vi "ControlProgram5.3.vi"() -> ()   [LabVIEW 2016]
uses:
  <vilib>/Utility/error.llb/DialogType.ctl
  <vilib>/Utility/miscctls.llb/LVPoint32TypeDef.ctl
  <vilib>/DAQmx/write.llb/DAQmx Write (Digital Bool 1Line 1Point).vi
  <vilib>/DAQmx/create/channels.llb/DAQmx Create Channel (DO-Digital Output).vi
  <vilib>/platform/TimedLoop/XDataNode/XDataNode.xnode
  <vilib>/Platform/TimedLoop/XDataNode/nitl_modes.ctl
  <vilib>/Platform/TimedLoop/XDataNode/XDNodeRunTimeDep.lvlib
  <vilib>/Platform/TimedLoop/XDataNode/wakeup.ctl
  <vilib>/Platform/TimedLoop/XDataNode/timing_clust.ctl
  <vilib>/DAQmx/create/channels.llb/DAQmx Create Channel (AI-Voltage-Basic).vi
  <vilib>/DAQmx/create/channels.llb/DAQmx Create Channel (AO-Voltage-Basic).vi
  <vilib>/DAQmx/write.llb/DAQmx Write (Analog 1D DBL NChan 1Samp).vi
  <resource>/objmgr/daqmx.rc
  <vilib>/Analysis/NI_AALBase.lvlib
  <vilib>/Analysis/baseanly.llb/Mean (DBL).vi
  <vilib>/Instr/_visa.llb/VISA Configure Serial Port (Instr).vi
  <vilib>/DAQmx/read.llb/DAQmx Read (Analog 2D DBL NChan NSamp).vi
  <vilib>/Utility/inputDevices.llb/closeMouse.vi
  <vilib>/Utility/inputDevices.llb/mouseAcquire.vi
  <vilib>/DAQmx/configure/timing.llb/DAQmx Timing (Sample Clock).vi
panel:
  out "Numeric 2":i32
  out "Numeric":i32
  in  "dt":dbl
  out "Flush Sample Start Time":u32
  out "Sample flush time (s)":dbl=100.0
  in  "Inject Sample":bool
  out "Chart Freq (Hz)":dbl
  out "Cal values":T1={"AX alpha"=672.9952101249002, "BX alpha"=822.8320399167465, "AX kappa"=0.3432739170419873, "BX kappa"=0.22087046979741862, "AX offset"=-0.002065833400375715, "BX offset"=0.010483360643544744, "AY alpha"=702.0654168010462, "BY alpha"=773.6701766674906, "AY kappa"=0.33643150106915, "BY kappa"=0.2444549177225145, "AY offset"=-0.1177594339643395, "BY offset"=0.06470506082263472}
  in  "Inject Pump 1":bool
  in  "Inject Pump 2":bool
  in  "Tab Control 2":T2(tab)
  in  "Force FB script":bool
  in  "Got ADig bead":bool
  in  "Move Cap. 2 (ADig Top)":bool
  in  "Dump beads":bool
  in  "Got DNA bead":bool
  in  "Flow on\ncap 2?":bool=TRUE
  in  "Flow on\ncap 1?":bool=TRUE
  in  "Flow on\ndump?":bool=TRUE
  in  "Delta after tether":dbl=2.4
  in  "TA Cancel Save?":bool
  in  "Min fish\ndelta (V)":dbl=2.8 min=0.0 max=10.0 step=0.1
  in  "Max fish\ndelta (V)":dbl=3.8 min=0.0 max=10.0 step=0.1
  in  "Fish Speed (ms)":i32=3000
  in  "Wait (ms)":i32=1500
  in  "# attempts":dbl=10.0
  in  "Cutoff force (pN)":dbl=5.0
  in  "Raster after\n tether?":bool=TRUE
  out "Tether":bool
  out "Attempt #":i32
  in  "Flow on\nwhile fish?":bool=TRUE
  in  "Flow on\nafter raster?":bool=TRUE
  in  "Offset @ Delta (V)":dbl=2.4
  in  "Cal @ Delta (V)":dbl=5.0
  in  "Cal stage position":i32=3
  in  "Conv Y (nm/V)":dbl=505.0
  in  "Conv X (nm/V)":dbl=892.0
  out "Cal Final Sampling Rate":dbl
  in  "Cal Averaging":i32=1
  in  "Wait before dip (s)":dbl=3.0
  in  "Start dipping after?":bool
  in  "Start trap delta (V)":dbl=3.85
  in  "Cancel dwell":bool
  in  "Pause dwell":bool
  in  "Return position":dbl=3.0
  in  "Dip duration":dbl=15.0
  in  "Dip position":dbl=4.0
  in  "Dip":bool
  out "Dip time":i32
  in  "Stop":bool=TRUE
  in  "?":T3(tab)=enum."Mouse control"
  in  "Save N sets":bool
  in  "N sets":i32=200
  in  "Cal sets to save":i32=500
  in  "Reset data stream":bool
  out "Buffer Overflow":bool
  out "Stage moving":bool
  in  "Comment":string="wtUvrD 0.5 uM ATP"
  in  "Raster scan":bool
  out "Saving":bool
  in  "Save cal":bool
  in  "Save Data":bool
  in  "Stop saving":bool
  out "Calibrating":bool
  out "Progress":dbl(slide) scale=0.0..100.0
  in  "Read Cal":bool
  in  "Fish":bool
  in  "Averaging Number":i32=1250
  out "Final Sampling Rate":dbl=100.0
  in  "Trap position":cluster{"X":dbl, "Y":dbl}={"X"=1.6, "Y"=4.95}
  in  "Trap delta":dbl=5.1 min=0.0 max=10.0 step=0.1
  in  "Fixed X":dbl=1.6
  in  "Fixed Y":dbl=0.7
  in  "Shutter 1 (B)":bool
  in  "Shutter 2 (A)":bool
  in  "Pulling direction":bool=TRUE
  out "Raster scanning...":bool
  out "Current file name":path
  in  "AX alpha":dbl format="%#_3p"
  in  "BX alpha":dbl format="%#_3g"
  in  "AX kappa":dbl format="%#_3g"
  in  "BX kappa":dbl format="%#_3g"
  in  "AX offset":dbl format="%#_3g"
  in  "BX offset":dbl format="%#_3g"
  in  "AY alpha":dbl format="%#_3g"
  in  "BY alpha":dbl format="%#_3g"
  in  "AY kappa":dbl format="%#_3g"
  in  "BY kappa":dbl format="%#_3g"
  in  "AY offset":dbl format="%#_3g"
  in  "BY offset":dbl format="%#_3g"
  out "Buffer status":u8(slide) scale=0.0..100.0
  in  "dump spot":string="Dump beads spot"
  in  "up flow spot":string="Upper flow spot"
  in  "low flow spot":string="Lower flow spot"
  in  "up cap":string="Upper capillary (ADig beads)"
  in  "bottom cap":string="Lower capillary (DNA beads)"
  in  "Move to Position 5":bool
  in  "Set Position 5":bool
  in  "Saved stage positions":dbl[][](array[numeric])=[[1.0, 0.0, 0.0, 0.0], [2.0, 0.28481, -2.63158, -0.02256], [3.0, 1.27978, -0.73974, 0.0], [4.0, 1.27978, -2.1978, 0.0], [5.0, 0.03306, -2.63158, -0.02256]]
  in  "Set Position 2":bool
  in  "Move to Position 2":bool
  in  "Set Position 1":bool
  in  "Move to Position 1":bool
  in  "Set Position 4":bool
  in  "Move to Position 4":bool
  in  "Set Position 3":bool
  in  "Move to Position 3":bool
  out "Stage error":errorcluster
  in  "Clear Volume":bool
  out "Sample Flush Meter":u8(slide) scale=0.0..100.0
  out "Flushing Sample":bool
  in  "Flush Sample":bool
  in  "Normal \nRate (ul/hr)  3":dbl=100.0
  in  "Normal \nVolume (ul) 3":dbl=300.0
  in  "Normal \nVolume (ul) 2":dbl
  in  "Normal \nRate (ul/hr)":dbl
  in  "Normal \nVolume (ul)":dbl
  in  "Flush\nRate (ul/min)":dbl
  in  "Flush\nVolume (ul)":dbl
  in  "Flush \nRate (ul/min)  2":dbl
  in  "Flush Pump 2":bool
  in  "Flush\nVolume (ul)  2":dbl
  in  "Flush Pump 1":bool
  in  "Normal \nRate (ul/hr)  2":dbl
  in  "Write Wait":i32=1000
  in  "Flush \nRate (ul/min)  3":dbl=100.0
  in  "Flush\nVolume (ul)  3":dbl=100.0
  out "error out":errorcluster
  in  "Use Mouse to Move Trap?":bool
  in  "Pause Mouse/Mirror Connection":bool
  out "Reference Voltage":cluster{dbl, dbl}={0.0, -0.0}
  out "Saved voltage":cluster{dbl, dbl}
  out "Real Coordinates":cluster{"Horizontal":i32, "Vertical":i32}={"Horizontal"=145, "Vertical"=-1746}
  out "CoordinatesMousePressed":T4
  out "Sum error":dbl(knob) scale=-1.0..1.0
  out "Trap sep":waveform(dbl)[](graph)
  in  "Set reading to\nsetpoint":bool
  in  "Offset Y (nm)":dbl format="%0.2f"
  in  "Offset X (nm)":dbl format="%0.2f"
  in  "Remove offsets":bool
  in  "Force Feedback":bool
  out "Feedback Output Voltage 2":cluster{dbl, dbl} {"?" format="%#_4g"; "?" format="%#_4g"}
  in  "Max value X":dbl=10.0 format="%.1f"
  in  "Min value X":dbl format="%0.1f"
  in  "Max value Y":dbl=10.0 format="%.1f"
  in  "Min value Y":dbl format="%.1g"
  in  "Offset":cluster{"Off Y":dbl, "Off X":dbl}={"Off Y"=1.5, "Off X"=0.17}
  in  "Setpoint voltage":cluster{"SP Y":dbl, "SP X":dbl}={"SP Y"=0.6, "SP X"=0.0}
  in  "Feedback const":T5={"Ki_B_Y"=0.5, "Ki_B_X"=0.0, "Kp Y"=1.0, "Kp X"=0.0}
  out "Mean Trap Pos X 2 (nm)":dbl format="%0.2f"
  out "Mean Trp Pos Y 2 (nm)":dbl format="%0.2f"
  out "T2 X RMS (A)":dbl format="%0.2f"
  out "T2 Y RMS (A)":dbl format="%0.2f"
  in  "Scan range (nm)":dbl=500.0
  in  "Scan speed (nm/s)":dbl=100.0
  in  "Step size (nm)":dbl=1.0
  in  "Save scans":bool=TRUE
  in  "# scans":i32=1
  in  "Load param":bool
  in  "Scan Parameters":T6(array[cluster])=[{"Label"="Offset", "Max delta 2"=3.8, "Start delta 2"=2.4, "Speed (ms) 2"=10000, "# scans 2"=1}]
  in  "Trap delta\nafter":dbl=3.6
  in  "Stop raster":bool
  out "Scan range (V)":dbl
  out "Scan steps (mirror)":u64
  out "Scan increment (V)":dbl
  out "Time per step (ms)":dbl
  out "Total raster time (s)":dbl
  out "N sets to be saved":dbl
  out "Continue to display?":bool
  out "Video Error":errorcluster
  in  "# Samples/channel (in)":i32=40000 format="%.2f"
  out "Buffer size\n(Samples/channel)":u32
  out "DAQ rate\n(Samples/s)":dbl format="%#_6p"
  out "# Samples/channel":i32=1250
  out "# Samples/channel/s":dbl
  out "AvailSampPerChan":u32
  out "Data update period (s/set)":dbl format="%#_6p"
  out "AvailSampPerChan 2":u32
  in  "PC samp per channel":i32=1000
  in  "Sampling Rate":dbl=125000.0 format="%0.0p"
  in  "DAQ Rate2":dbl=1000000.0 format="%#_6p"
  out "Data period (s)":dbl format="%#_6p"
  in  "Tether break\nforce (pN)":dbl=1.0
  in  "Path":path=path "D:/data"
  in  "Save file index":dbl
  out "Mirror task":refnum<k21>
  in  "HWP1":string="Half waveplate 1: differential trap power"
  in  "HWP0":string="Half waveplate 0: total trap power"
  in  "Move 1":bool
  in  "\"Degrees\" 1":dbl
  in  "Move 0":bool
  in  "\"Degrees\" 0":dbl
  out "Chamber":T7(plugin-control)
  out "Deflection":T4
  in  "Sampling Rate":dbl=125000.0 format="%0.2f"
  in  "Averaging Number":i32=12500
  in  "DAQ Rate":dbl=1000000.0
  out "Final Sampling Rate":dbl
  in  "Tab Control":T8(tab)
  in  "Downsamp\nfact":dbl=250.0
  out "Bead sep":waveform(dbl)[](graph)
  out "Force (pN)":waveform(dbl)[](graph)
  out "Mean force (pN)":dbl format="%0.2f"
  out "Force noise (pN)":dbl format="%0.2f"
  out "Mean Bead Sep\n(nm)":dbl format="%0.2f"
  out "Bead Sep Noise\n(A)":dbl format="%0.2f"
  out "PSD 2":cluster{dbl[], dbl[]}(graph)
  out "PSD 1":cluster{dbl[], dbl[]}(graph)
  out "PSD 1 Sum":dbl(slide) scale=0.0..10.0
  out "PSD 2 Sum":dbl(slide) scale=0.0..10.0
  in  "Start":bool
  out "All signals":waveform(dbl)[](graph)
  # "Bead Calibration"
  # "X"
  # "Y"
  # "Pump #1 Controls"
  # "Pump #2 Controls"
  # "Sample Pump Controls"
  # "Retract the pumps manually. Change it back to INFUSE when you're done. Suck it up, don't whine."
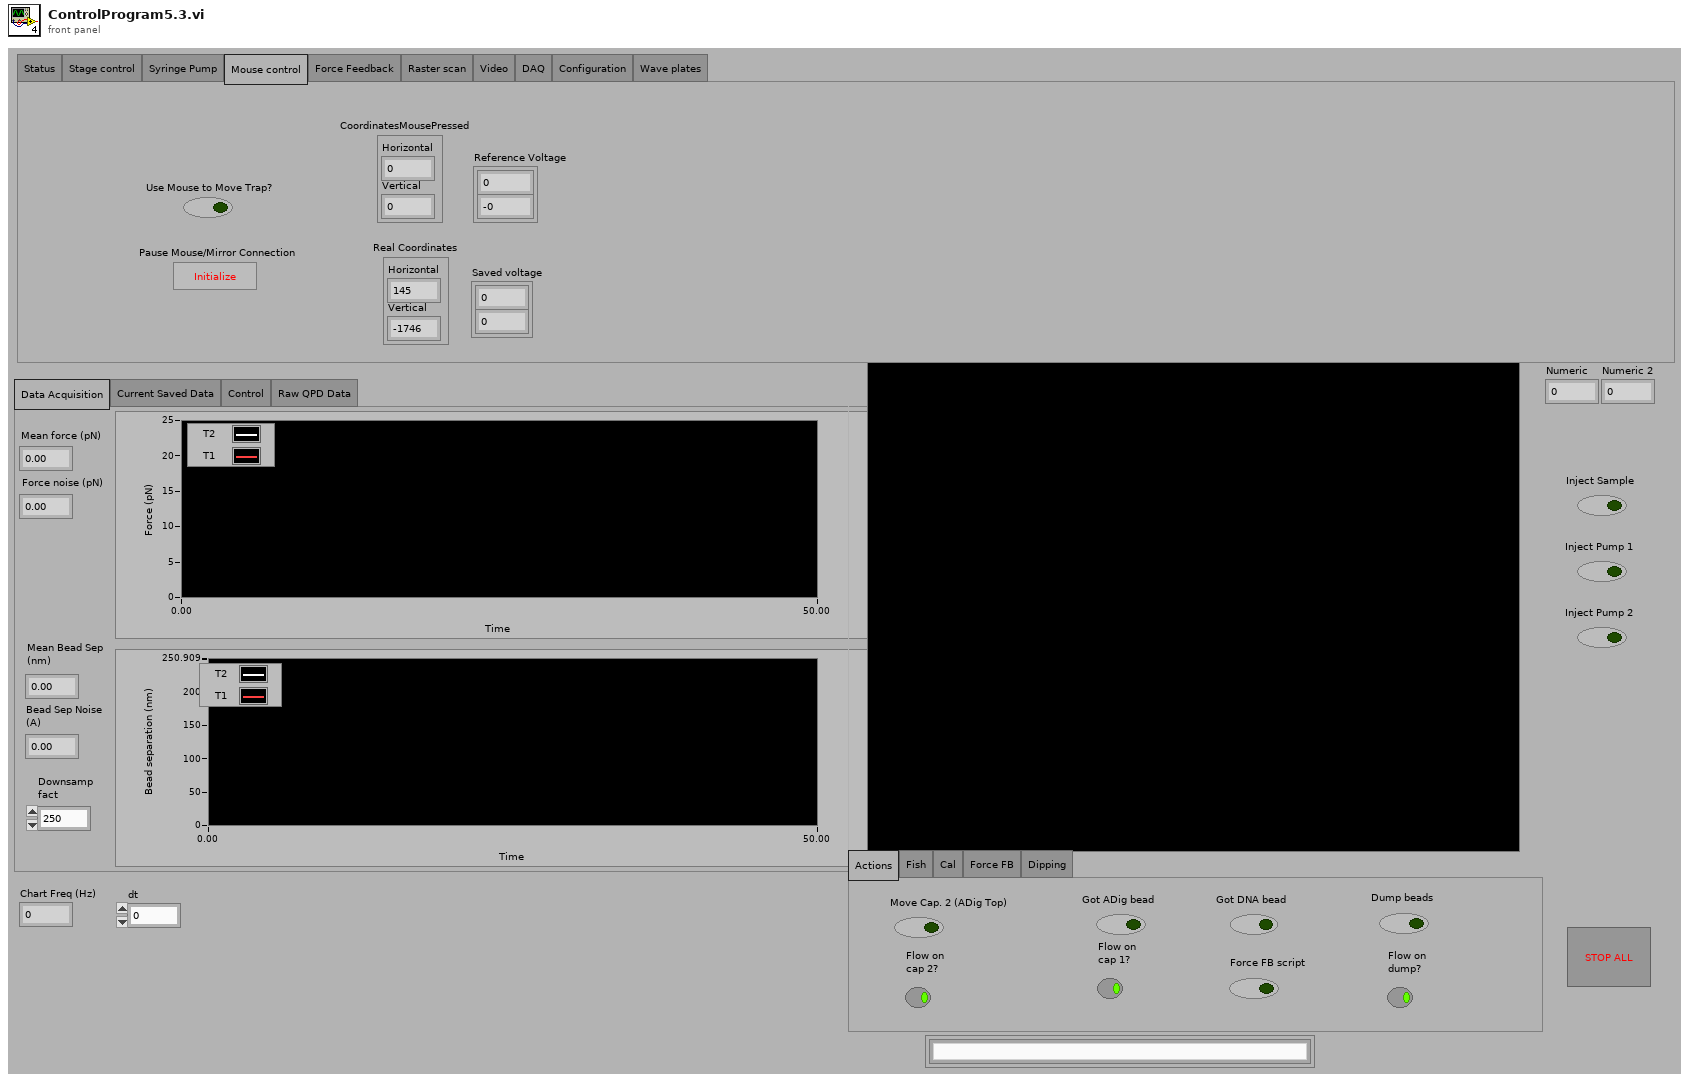
[diagram p1: front panel]
types:
  T1 = cluster{"AX alpha":dbl, "BX alpha":dbl, "AX kappa":dbl, "BX kappa":dbl, "AX offset":dbl, "BX offset":dbl, "AY alpha":dbl, "BY alpha":dbl, "AY kappa":dbl, "BY kappa":dbl, "AY offset":dbl, "BY offset":dbl}
  T2 = enum32{"Actions", "Fish", "Cal", "Force FB", "Dipping"}
  T3 = enum32{"Status", "Stage control", "Syringe Pump", "Mouse control", "Force Feedback", "Raster scan", "Video", "DAQ", "Configuration", "Wave plates"}
  T4 = typedef "LVPoint32TypeDef.ctl" = cluster{"Horizontal":i32, "Vertical":i32}
  T5 = cluster{"Ki_B_Y":dbl, "Ki_B_X":dbl, "Kp Y":dbl, "Kp X":dbl}
  T6 = cluster{"Label":string, "Max delta 2":dbl, "Start delta 2":dbl, "Speed (ms) 2":i32, "# scans 2":i32}[]
  T7 = typedef "IMAQ Image.ctl" = refnum<image>
  T8 = enum32{"Data Acquisition", "Current Saved Data", "Control", "Raw QPD Data"}
  T9 = enum16{"open", "replace", "create", "open or create", "replace or create", "replace or create with confirmation"}
  T10 = enum16{"big-endian, network order", "native, host order", "little-endian"}
  T11 = cluster{string, string, string, string, string, string, string, string}
  T12 = typedef "XDNodeRunTimeDep.lvlib/timing_clust.ctl" = cluster{"Expected End [f-1]":u64, "Actual End [f-1]":u64, "Finished Late? [f-1]":bool, "Expected End [i-1]":u64, "Actual End [i-1]":u64, "Finished Late? [i-1]":bool, "Expected Start [i]":u64, "Actual Start [i]":u64, "Expected Start [f]":u64, "Actual Start [f]":u64, "Source Name":string, "Structure Name":string, "Period":i64, "Deadline":i64, "Offset":i64, "Start":i64, "Priority":i32, "Timeout":i32, "Mode":T13, "Wakeup Reason":T14, "Error":errorcluster, "Source Type":string, "Secondary Source Type":string, "Global End Time":u64, "Global Start Time":u64, "Frame Duration":u64, "Iteration Duration":u64, "Assigned CPU":i32, "I/O Scan Engine Mode":u32}
  T13 = typedef "XDNodeRunTimeDep.lvlib/nitl_modes.ctl" = enum32{"No Change", "Process missed periods, maintain original phase", "Discard missed periods, maintain original phase", "Process missed periods, ignore original phase", "Discard missed periods, ignore original phase"}
  T14 = typedef "XDNodeRunTimeDep.lvlib/wakeup.ctl" = enum32{"Normal", "Aborted", "Asynchronous wakeup", "Timing source error", "Timed loop error", "Timeout"}
  T15 = typedef "DialogType.ctl" = u16
  T16 = cluster{"button 1":bool, "button 2":bool, "button 3":bool, "button 4":bool}
  T17 = cluster{"[0]":dbl, "[1]":dbl, "[2]":dbl, "[3]":dbl, "[4]":dbl, "[5]":dbl, "[6]":dbl, "[7]":dbl, "[8]":dbl, "[9]":dbl, "[10]":dbl, "[11]":dbl}
  T18 = cluster{"Label":string, "Max delta 2":dbl, "Start delta 2":dbl, "Speed (ms) 2":i32, "# scans 2":i32}
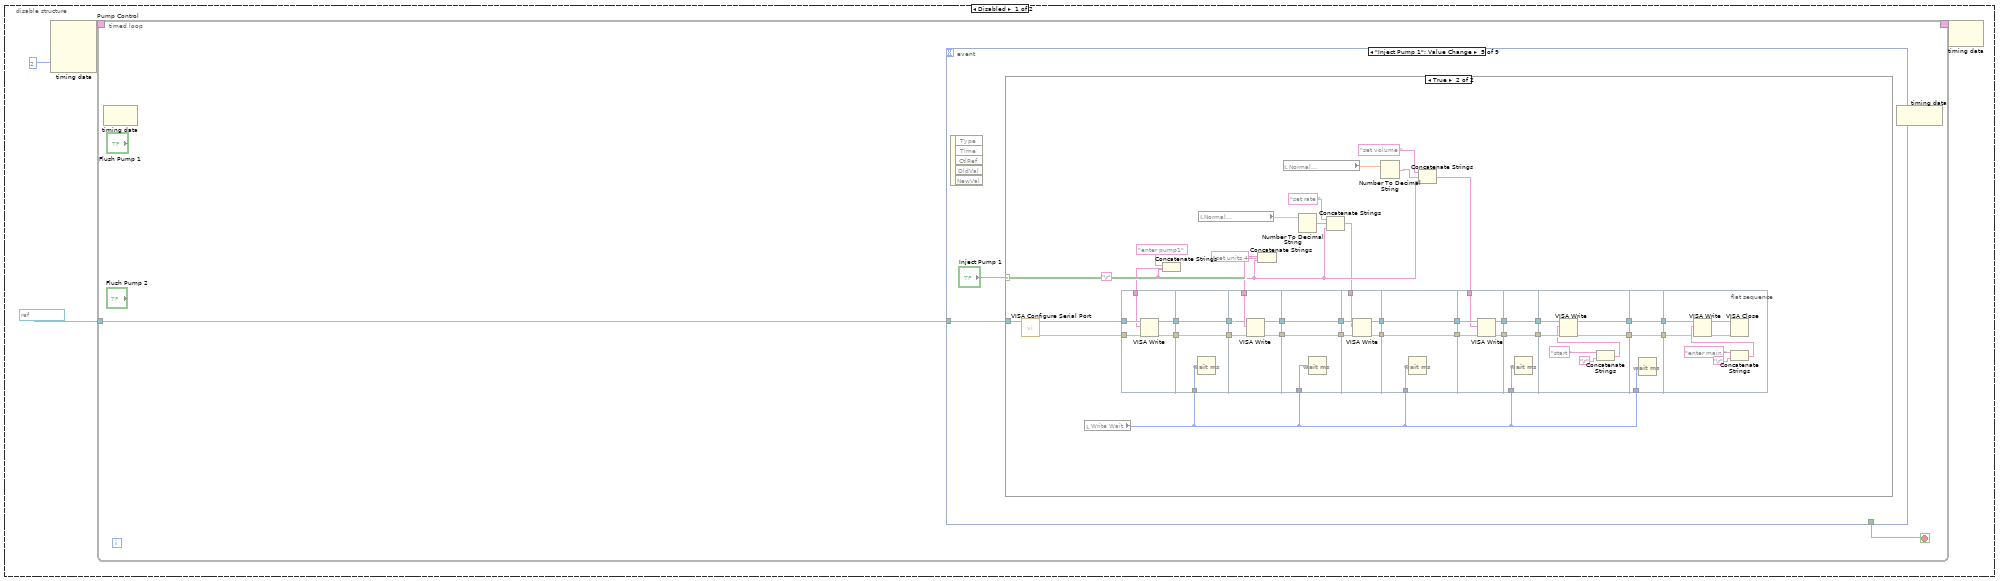
[diagram p2: hidden frame]
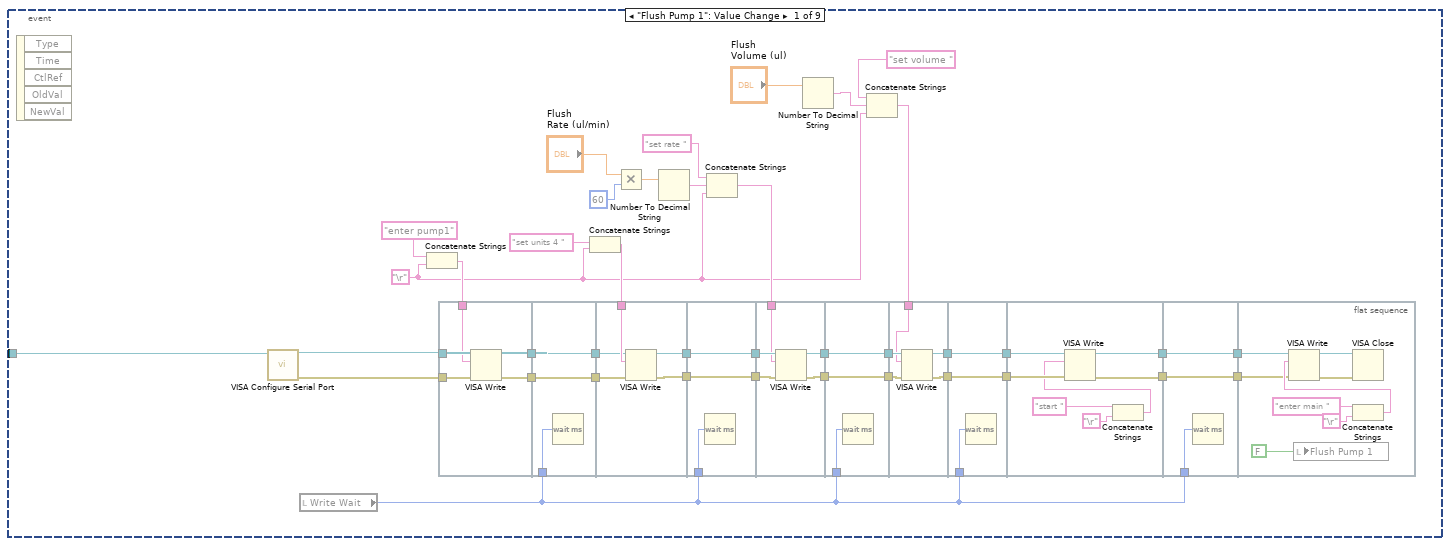
[diagram p3: hidden frame]
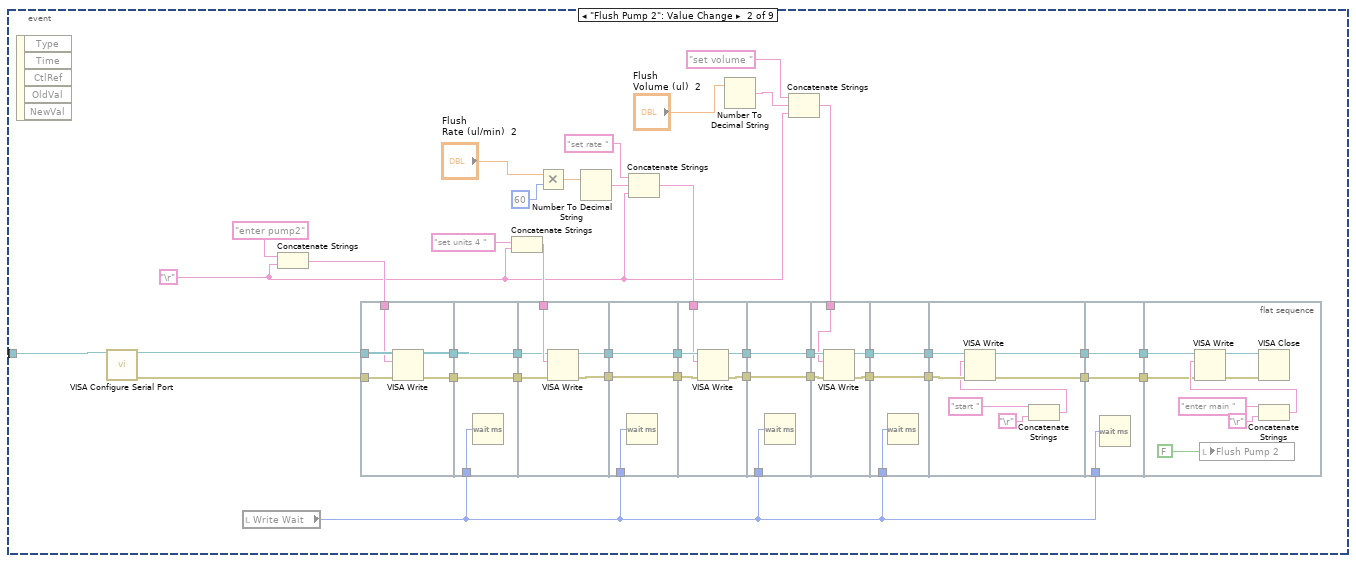
[diagram p4: hidden frame]
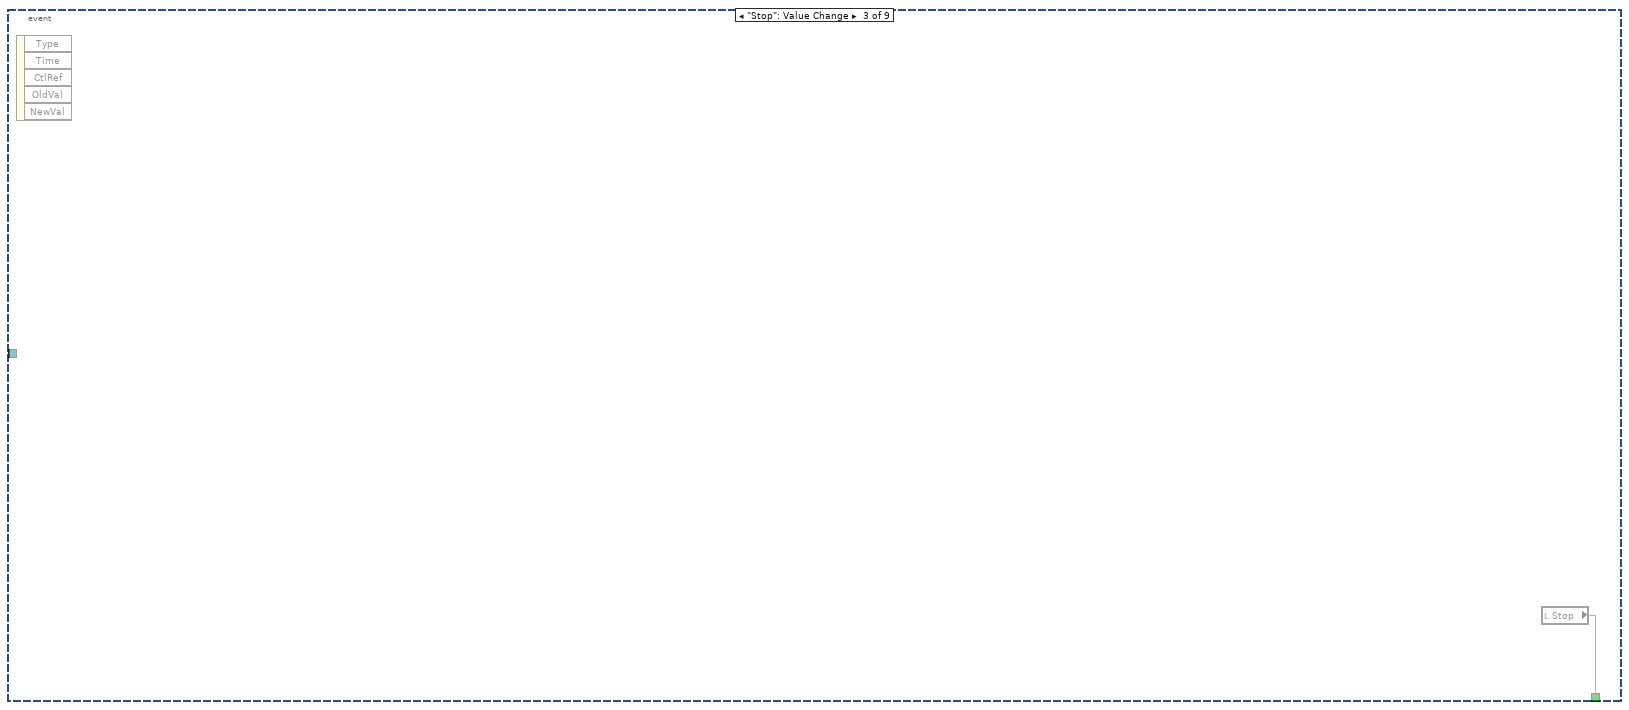
[diagram p5: hidden frame]
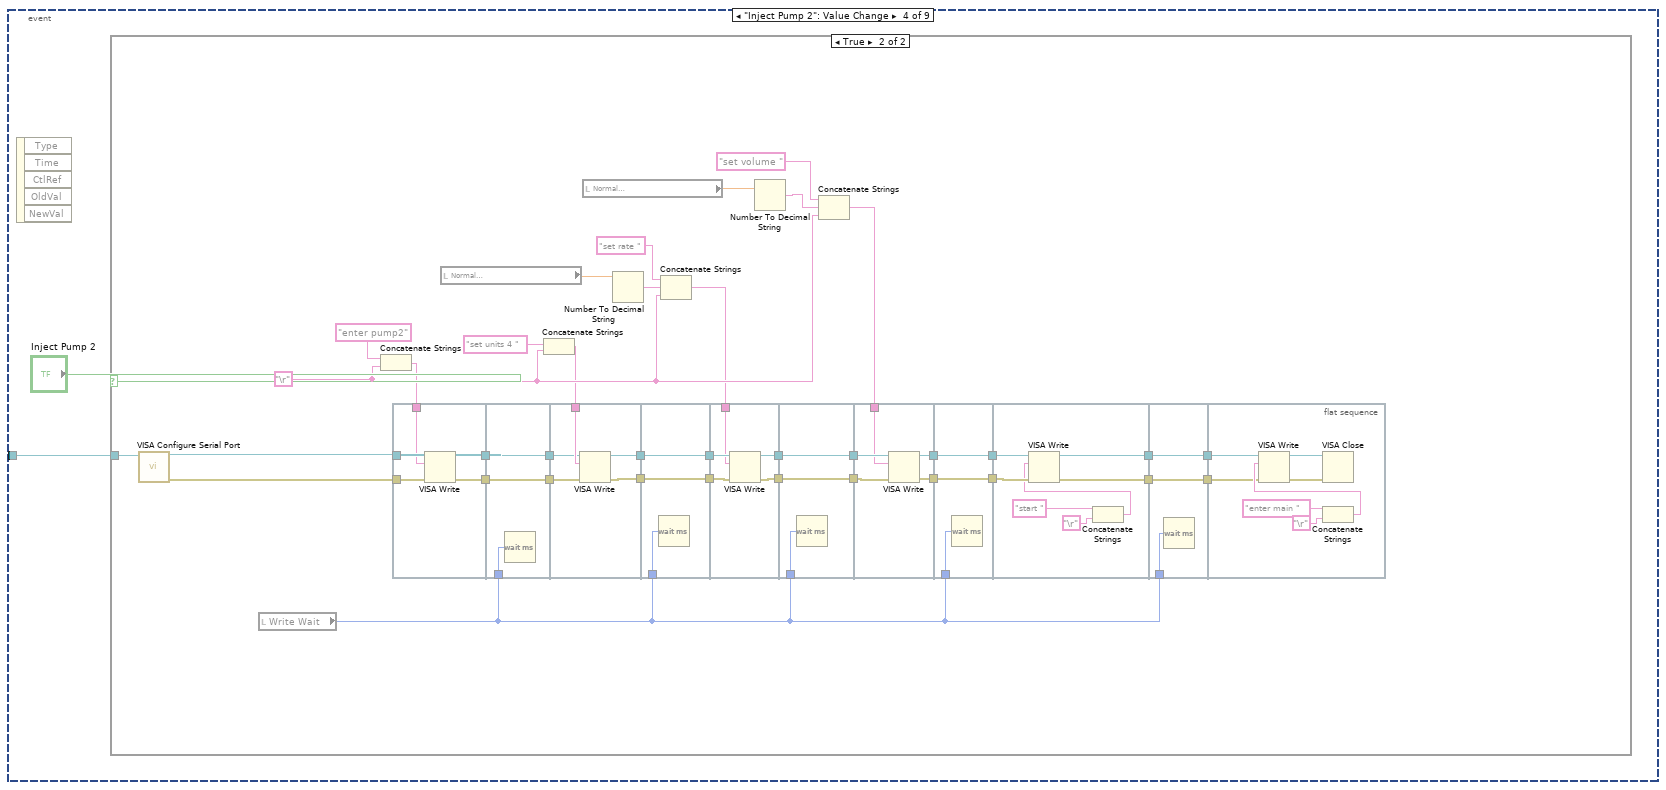
[diagram p6: hidden frame]
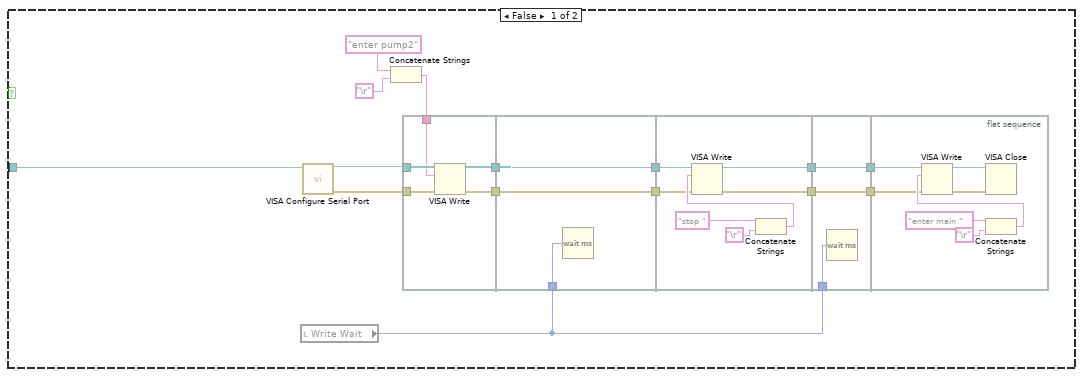
[diagram p7: hidden frame]
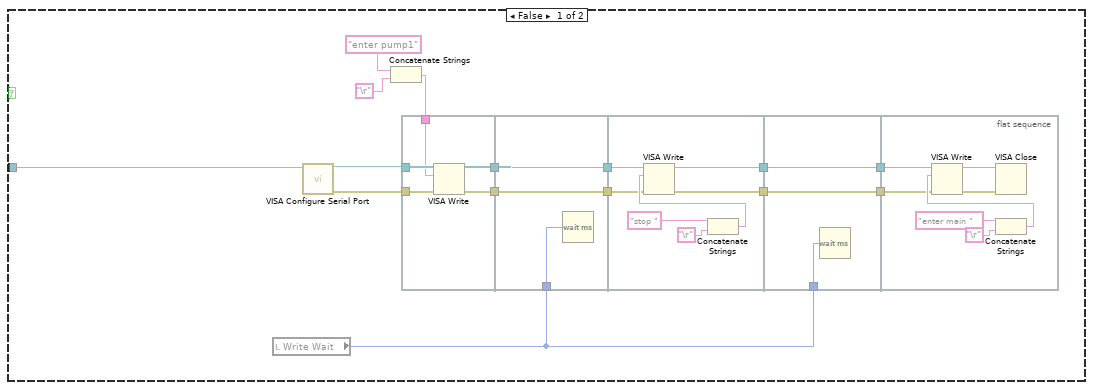
[diagram p8: hidden frame]
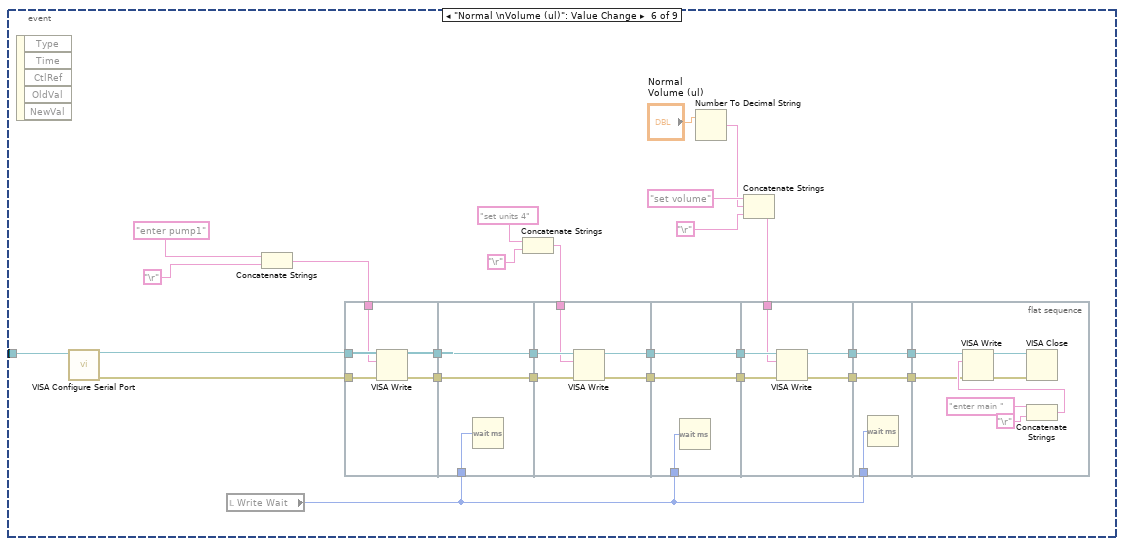
[diagram p9: hidden frame]
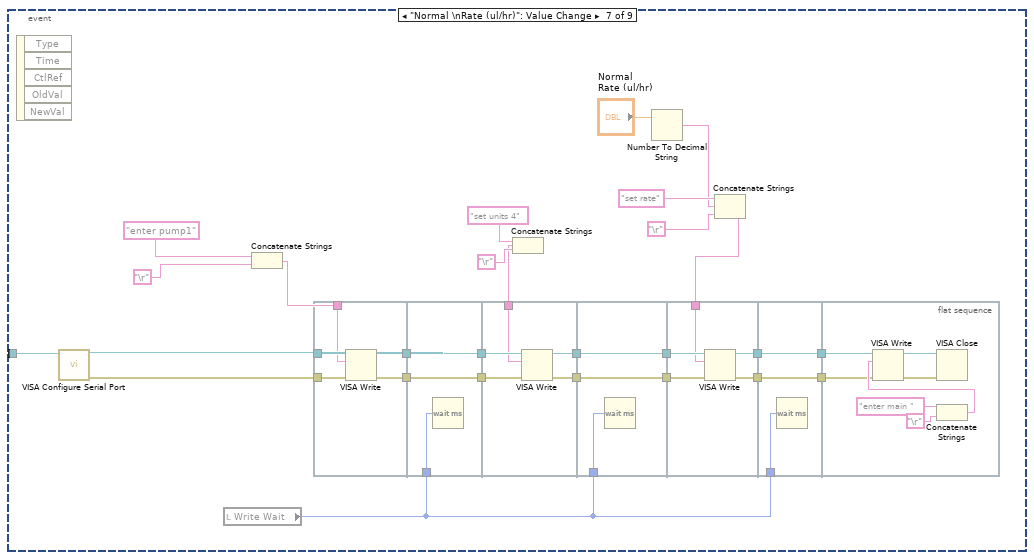
[diagram p10: hidden frame]
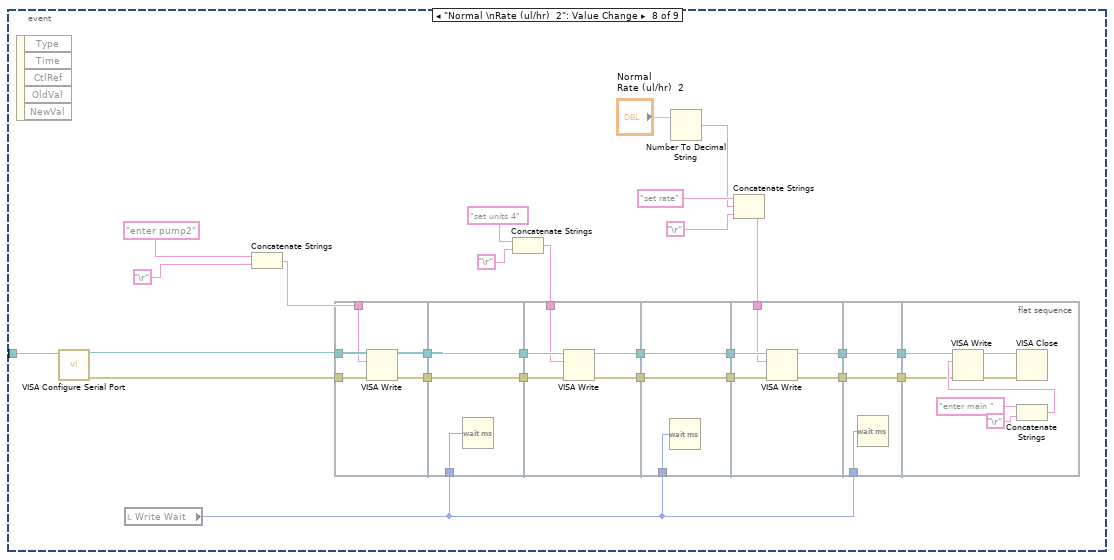
[diagram p11: hidden frame]
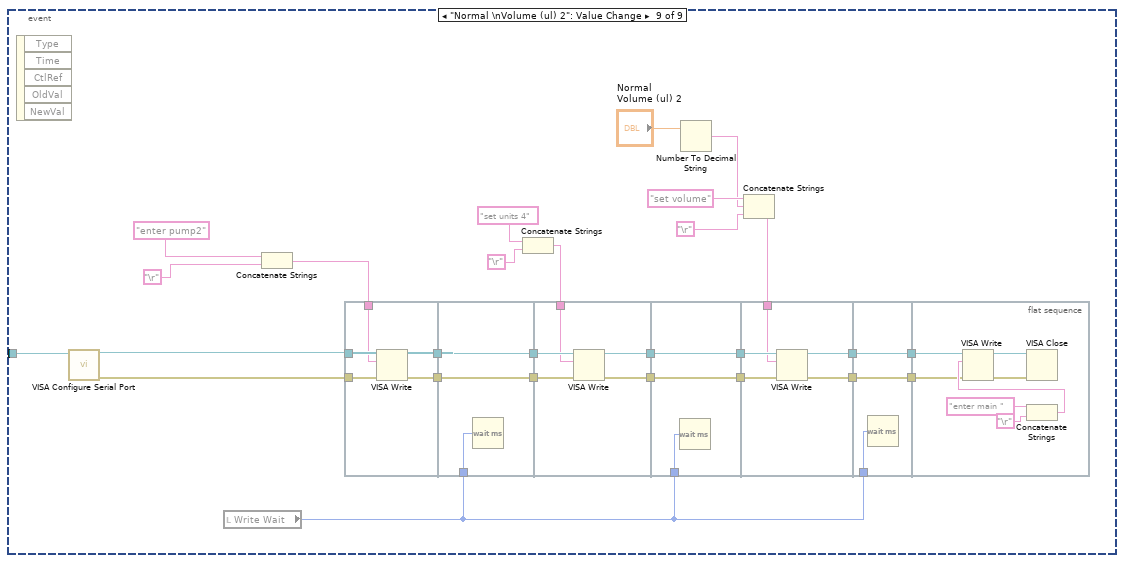
[diagram p12: hidden frame]
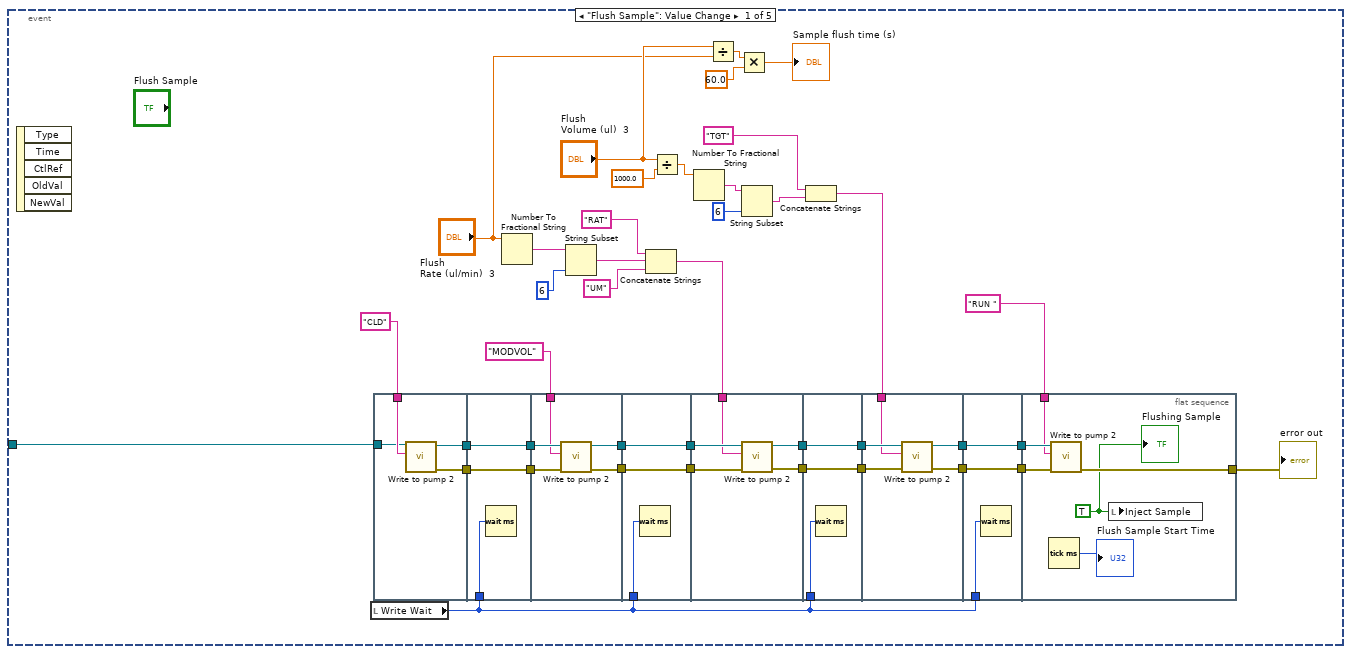
[diagram p13: hidden frame]
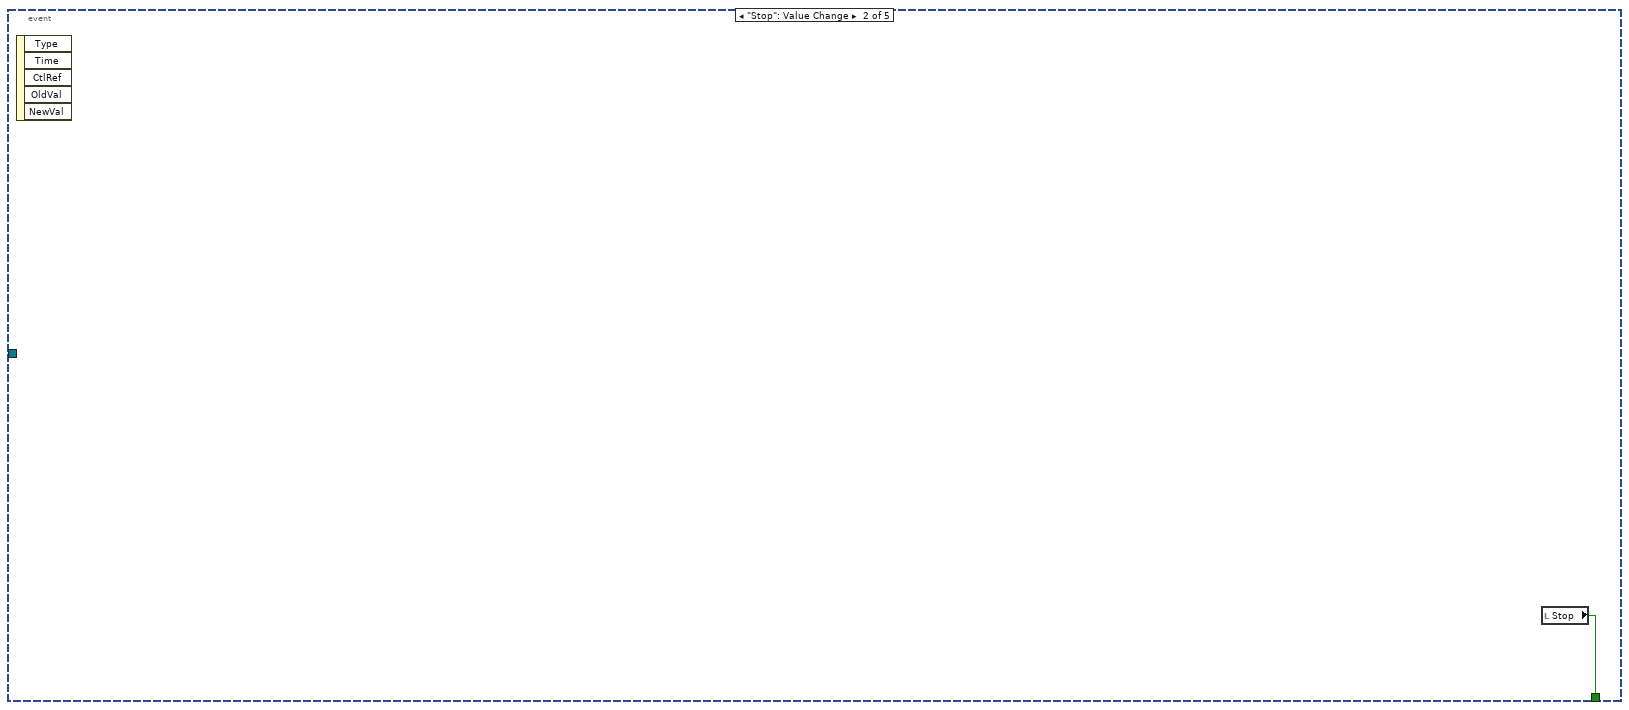
[diagram p14: hidden frame]
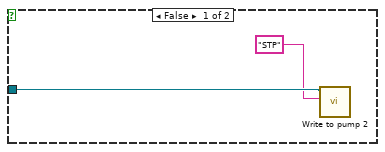
[diagram p15: hidden frame]
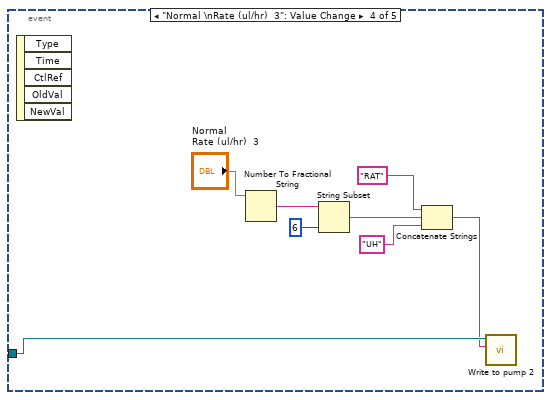
[diagram p16: hidden frame]
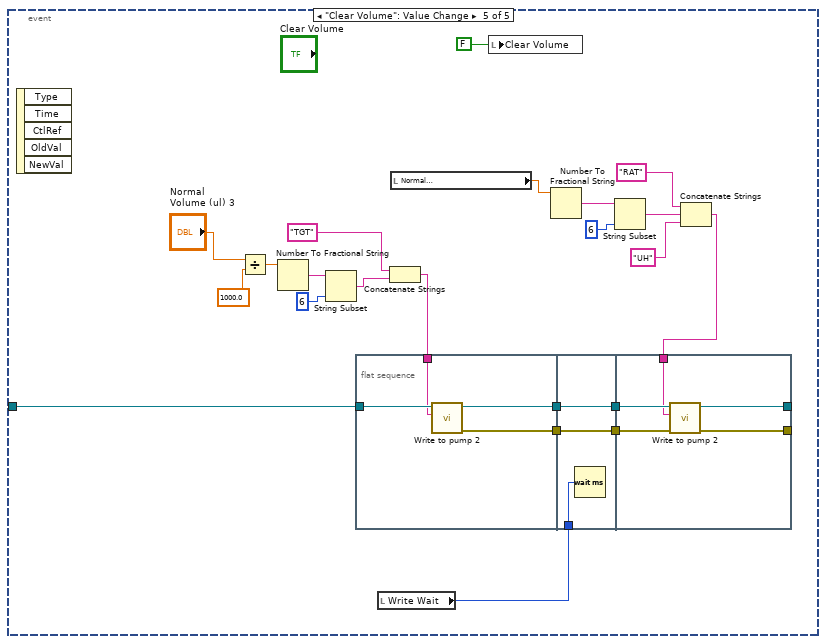
[diagram p17: hidden frame]
diagram:
  w42 = 10.0 ("Minimum Value")
  w43 = -10.0 ("Minimum Value")
  w45 = -2.0 ("Minimum Value")
  w46 = 2.0 ("Maximum Value")
  w71 = 10123 items=["Finite Samples"=10178, "Continuous Samples"=10123] ("sample mode")
  w92 = tag "Dev1/port2/line1"  # Shutter 2
  w95 = tag "Dev1/port1/line4"  # Shutter 1
  # "Create channels for movable mirror"
  # "Create channels for detectors"
  n1 = call-poly <vilib>:"DAQmx Create Virtual Channel.vi"("maximum value"=w46, "minimum value"=w45, "physical channels"=tag "Dev1/ai0" ("Physical Channel")) -> ("task out"=w47:refnum<k21>, "error out"=w70:errorcluster)  [unwired: 11 in]
  n2 = call-poly <vilib>:"DAQmx Create Virtual Channel.vi"("task in"=w47, "maximum value"=w46, "minimum value"=w45, "physical channels"=tag "Dev1/ai1", "error in"=w70) -> ("task out"=w68:refnum<k21>, "error out"=w67:errorcluster)  [unwired: 9 in]
  n3 = call-poly <vilib>:"DAQmx Create Virtual Channel.vi"("task in"=w68, "maximum value"=w46, "minimum value"=w45, "physical channels"=tag "Dev1/ai2", "error in"=w67) -> ("task out"=w59:refnum<k21>, "error out"=w58:errorcluster)  [unwired: 9 in]
  n4 = call-poly <vilib>:"DAQmx Create Virtual Channel.vi"("task in"=w59, "maximum value"=w46, "minimum value"=w45, "physical channels"=tag "Dev1/ai3" ("Physical Channel"), "error in"=w58) -> ("task out"=w44:refnum<k21>, "error out"=w64:errorcluster)  [unwired: 9 in]
  n5 = call-poly <vilib>:"DAQmx Create Virtual Channel.vi"("task in"=w44, "maximum value"=w42, "minimum value"=w43, "physical channels"=tag "Dev1/ai4", "error in"=w64) -> ("task out"=w62:refnum<k21>, "error out"=w61:errorcluster)  [unwired: 9 in]
  n6 = call-poly <vilib>:"DAQmx Create Virtual Channel.vi"("task in"=w62, "maximum value"=w42, "minimum value"=w43, "physical channels"=tag "Dev1/ai5", "error in"=w61) -> ("task out"=w57:refnum<k21>, "error out"=w56:errorcluster)  [unwired: 9 in]
  n7 = call-poly <vilib>:"DAQmx Create Virtual Channel.vi"("task in"=w57, "maximum value"=w42, "minimum value"=w43, "physical channels"=tag "Dev1/ai6", "error in"=w56) -> ("task out"=w51:refnum<k21>, "error out"=w49:errorcluster)  [unwired: 9 in]
  n8 = call-poly <vilib>:"DAQmx Create Virtual Channel.vi"("task in"=w51, "maximum value"=w42, "minimum value"=w43, "physical channels"=tag "Dev1/ai7", "error in"=w49) -> ("task out"=w50:refnum<k21>, "error out"=w48:errorcluster)  [unwired: 9 in]
  n9 = call-poly <vilib>:"DAQmx Timing.vi"("task/channels in"=w50, "sample mode"=w71, "samples per channel"="PC samp per channel", "rate"="Sampling Rate", "error in"=w48) -> ("task out"=w54:refnum<k21>, "error out"=w53:errorcluster)  [unwired: 9 in]
  n10 = call-poly <vilib>:"DAQmx Create Virtual Channel.vi"("maximum value"="Max value Y", "minimum value"="Min value Y", "physical channels"=tag "Dev1/ao1" ("Trap X Axis")) -> ("task out"=w39:refnum<k21>, "error out"=w41:errorcluster)  [unwired: 11 in]
  n11 = property class="DAQmx Timing"(reference=w54, error in=w53, "More:AI Convert:Rate"="DAQ Rate2") -> (reference out=w6:refnum<k21>, error out=w5:errorcluster, "SampClk.Rate"=→"DAQ rate\n(Samples/s)":dbl)
  n12 = call-poly <vilib>:"DAQmx Create Virtual Channel.vi"("task in"=w39, "maximum value"="Max value X", "minimum value"="Min value X", "physical channels"=tag "Dev1/ao0" ("Trap Y Axis"), "error in"=w41) -> ("task out"=w30:refnum<k21>, "error out"=w29:errorcluster)  [unwired: 9 in]
  "Mirror task" <- w30
  n13 = property class="DAQmx Buffer"(reference=w6, error in=w5) -> (reference out=w3:refnum<k21>, error out=w2:errorcluster, "Input.OnbrdBufSize"=→"Buffer size\n(Samples/channel)":u32)
  n14 = call <vilib>:"DAQmx Start Task.vi"("task/channels in"=w3, "error in"=w2) -> ("task out"=w31:refnum<k21>)  [unwired: 12 in, 1 out]
  n15 = while {
    tunnel: [w415] -> w77
    tunnel: [w307] -> w78
    tunnel: [w423] -> w76
    tunnel: [w420] -> w73
    tunnel: w31 -> [w120]
    tunnel: w30 -> [w416]
    tunnel: w29 -> [w421]
    stop <- w420 stop-if-true
    w151 = "NI_ChannelName" ("name")
    w227 = -1
    # "Rewire everything"
    # "Invert these because changed\nfrom PSD to QPD"
    # "Trap Y"
    # "Trap X"
    # "Convert to\npN"
    # "Convert to\nnm"
    # "Subtract\noffset"
    # "Normalize by\nsum"
    # "B sum"
    # "BX"
    # "BY"
    # "AX"
    # "AY"
    # "A sum"
    # "Close files when done saving"
    n16 = property class="DAQmx Read"(reference=w120) -> (reference out=w119:refnum<k21>, "AvailSampPerChan"=→"AvailSampPerChan 2":u32)  [unwired: 1 in, 1 out]
    n17 = local read "Averaging Number"() -> (w115:i32)
    n18 = local read "Averaging Number"() -> (w121:i32)
    "# Samples/channel" <- w121
    n19 = local read "Sampling Rate"() -> (w419:dbl)
    n20 = call-poly <vilib>:"DAQmx Read.vi"("task/channels in"=w119, "number of samples per channel"=w115, "timeout"=10.0) -> ("task out"=w306:refnum<k21>, "data"=w116:dbl[][], "error out"=w230:errorcluster)  [unwired: 10 in]
    n21 = Unbundle By Name(w230) -> ("status"=w355:bool)
    n22 = Divide(x=w419, y="Cal Averaging") -> (x/y=→"Cal Final Sampling Rate":dbl)
    n23 = Divide(x=w419, y=w121) -> (x/y=→"Final Sampling Rate" →"# Samples/channel/s":dbl)
    n24 = case shown="True" w355 {
      frame False {
      }
      frame True {
        n25 = call <vilib>:"Beep.vi"() -> ()  [unwired: 12 in]
        "Buffer Overflow" <- TRUE
      }
    }
    n26 = local read "Buffer size\n(Samples/channel)"() -> (w302:u32)
    n27 = property class="DAQmx Read"(reference=w306) -> (reference out=w305:refnum<k21>, "AvailSampPerChan"=w303:u32)  [unwired: 1 in, 1 out]
    "AvailSampPerChan" <- w303
    n28 = local read "Cal values"() -> (w347:T1)
    n29 = Index Array(array=w116, index (row)=4) -> (element=w219:dbl[])  [unwired: 1 in]
    n30 = Index Array(array=w116, index (row)=0) -> (element=w229:dbl[])  [unwired: 1 in]
    n31 = Index Array(array=w116, index (row)=2) -> (element=w224:dbl[])  [unwired: 1 in]
    n32 = Index Array(array=w116, index (row)=1) -> (element=w228:dbl[])  [unwired: 1 in]
    n33 = Index Array(array=w116, index (row)=3) -> (element=w222:dbl[])  [unwired: 1 in]
    n34 = Index Array(array=w116, index (row)=6) -> (element=w221:dbl[])  [unwired: 1 in]
    n35 = Index Array(array=w116, index (row)=7) -> (element=w220:dbl[])  [unwired: 1 in]
    n36 = Index Array(array=w116, index (row)=5) -> (element=w218:dbl[])  [unwired: 1 in]
    n37 = Divide(x=w303, y=w302) -> (x/y=→"Buffer status":dbl)
    n38 = Unbundle(w347) -> ("AX alpha"=w335:dbl, "BX alpha"=w331:dbl, "AX kappa"=w327:dbl, "BX kappa"=w323:dbl, "AX offset"=w341:dbl, "BX offset"=w339:dbl, "AY alpha"=w338:dbl, "BY alpha"=w333:dbl, "AY kappa"=w329:dbl, "BY kappa"=w325:dbl, "AY offset"=w345:dbl, "BY offset"=w343:dbl)
    n39 = Multiply(x=w228, y=w227) -> (x*y=w223:dbl[])
    n40 = Multiply(x=w229, y=w227) -> (x*y=w225:dbl[])
    n41 = local write "AX alpha"(w335) -> ()
    n42 = local write "BY offset"(w343) -> ()
    n43 = Build Array(w225, w224, w223, w222, w221, w220, w219, w218) -> (w148:dbl[][])
    n44 = local write "BX alpha"(w331) -> ()
    n45 = case shown="True" "Reset data stream" {
      selector: "Reset data stream" -> [_ w466]
      tunnel: w305 -> [w458 w464]
      tunnel: [w458 w462] -> w307
      tunnel: w230 -> [w457 w461]
      tunnel: [w457 w459] -> _
      frame False {
      }
      frame True {
        n46 = Not(x=w466) -> (.not. x?=w465:bool)
        n47 = call <vilib>:"DAQmx Stop Task.vi"("task/channels in"=w464, "error in"=w461) -> ("task out"=w463:refnum<k21>, "error out"=w460:errorcluster)  [unwired: 12 in]
        n48 = local write "Reset data stream"(w465) -> ()
        n49 = local write "Buffer Overflow"(w465) -> ()
        n50 = call <vilib>:"DAQmx Start Task.vi"("task/channels in"=w463, "error in"=w460) -> ("task out"=w462:refnum<k21>, "error out"=w459:errorcluster)  [unwired: 12 in]
      }
    }
    n51 = call-poly <vilib>:"Mean.vi"("X"=w218) -> ("mean"=w361:dbl)  [unwired: 1 out]
    n52 = local write "AY offset"(w345) -> ()
    n53 = call-poly <vilib>:"Mean.vi"("X"=w219) -> ("mean"=w362:dbl)  [unwired: 1 out]
    n54 = call-poly <vilib>:"Mean.vi"("X"=w224) -> ("mean"=w368:dbl)  [unwired: 1 out]
    n55 = call-poly <vilib>:"Mean.vi"("X"=w222) -> ("mean"=w366:dbl)  [unwired: 1 out]
    n56 = call-poly <vilib>:"Mean.vi"("X"=w221) -> ("mean"=w365:dbl)  [unwired: 1 out]
    n57 = call-poly <vilib>:"Mean.vi"("X"=w220) -> ("mean"=w364:dbl)  [unwired: 1 out]
    n58 = local read "Averaging Number"() -> (w114:i32)
    n59 = local write "BY kappa"(w325) -> ()
    n60 = local write "AX kappa"(w327) -> ()
    n61 = call-poly <vilib>:"Mean.vi"("X"=w223) -> ("mean"=w367:dbl)  [unwired: 1 out]
    n62 = local write "AY kappa"(w329) -> ()
    n63 = call-poly <vilib>:"Mean.vi"("X"=w225) -> ("mean"=w369:dbl)  [unwired: 1 out]
    n64 = local read "DAQ rate\n(Samples/s)"() -> (w126:dbl)
    n65 = Build Array(w362, w361) -> (w360:dbl[])
    n66 = local write "BX kappa"(w323) -> ()
    n67 = local write "BY alpha"(w333) -> ()
    n68 = local write "AX offset"(w341) -> ()
    n69 = local write "BX offset"(w339) -> ()
    n70 = local write "AY alpha"(w338) -> ()
    n71 = Build Array(w369, w368, w367, w366, w365, w364) -> (w358:dbl[])
    n72 = Divide(x=w114, y=w126) -> (x/y=w123:dbl)
    "Data update period (s/set)" <- w123
    n73 = Reciprocal(x=w126) -> (1/x=w127:dbl)
    "Data period (s)" <- w127
    n74 = Divide(x=w369, y=w365) -> (x/y=w399:dbl)
    n75 = Divide(x=w368, y=w365) -> (x/y=w400:dbl)
    n76 = Divide(x=w367, y=w364) -> (x/y=w407:dbl)
    n77 = Divide(x=w366, y=w364) -> (x/y=w408:dbl)
    n78 = Subtract(x=w399, y="AY offset") -> (x-y=w381:dbl)
    n79 = Subtract(x=w400, y="AX offset") -> (x-y=w382:dbl)
    n80 = Subtract(x=w407, y="BY offset") -> (x-y=w380:dbl)
    n81 = Subtract(x=w408, y="BX offset") -> (x-y=w383:dbl)
    n82 = Subtract(x=w407, y=w399) -> (x-y=w397:dbl)
    n83 = Subtract(x=w408, y=w400) -> (x-y=w398:dbl)
    n84 = feedback #1(0.0) -> (w301:dbl)
    n85 = Multiply(x="Downsamp\nfact", y=w127) -> (x*y=w128:dbl)
    n86 = Multiply(x=w381, y="AY alpha") -> (x*y=w315:dbl)
    n87 = Multiply(x=w382, y="AX alpha") -> (x*y=w313:dbl)
    n88 = Multiply(x=w383, y="BX alpha") -> (x*y=w314:dbl)
    n89 = Multiply(x=w380, y="BY alpha") -> (x*y=w316:dbl)
    n90 = Add(x=w123, y=w301) -> (x+y=w299:dbl)
    n91 = feedback-in #1(w299) -> ()
    n92 = Square(x=w315) -> (x^2=w391:dbl)
    n93 = Square(x=w313) -> (x^2=w392:dbl)
    n94 = Square(x=w316) -> (x^2=w393:dbl)
    n95 = Square(x=w314) -> (x^2=w394:dbl)
    n96 = Bundle(w397, w398) -> (w117:cluster{dbl, dbl})  [unwired: 1 in]
    n97 = case shown="True" "Set reading to\nsetpoint" {
      tunnel: w117 -> [_ w455]
      frame False {
      }
      frame True {
        n98 = local write "Set reading to\nsetpoint"(FALSE ("Set reading to\nsetpoint")) -> ()
        n99 = local read "Trap position"() -> (w454:cluster{"X":dbl, "Y":dbl})
        n100 = property on="Setpoint voltage" class="Clust (strict)"("Val(Sgnl)"=w455) -> ()  [unwired: 2 in, 2 out]
        n101 = Unbundle(w454) -> ("X"=w453:dbl, "Y"=w452:dbl)
        n102 = Bundle("Y"=w452, "X"=w453) -> (w451:cluster{"Y":dbl, "X":dbl})  [unwired: 1 in]
        n103 = property on="Offset" class="Clust (strict)"("Val(Sgnl)"=w451) -> ()  [unwired: 2 in, 2 out]
      }
    }
    n104 = Reciprocal(x=w128) -> (1/x=→"Chart Freq (Hz)":dbl)
    n105 = To Time Stamp(1:w299) -> (0:w298:timestamp)
    n106 = Add(x=w391, y=w392) -> (x+y=w395:dbl)
    n107 = Add(x=w393, y=w394) -> (x+y=w406:dbl)
    n108 = Multiply(x=w313, y="AX kappa") -> (x*y=w309:dbl)
    n109 = Bundle("A y", "A x", "B y", "B x", "A sum", "B sum", "Trap x", "Trap y") -> (w289:T11)  [unwired: 1 in]
    n110 = Multiply(x=w314, y="BX kappa") -> (x*y=w310:dbl)
    n111 = Square Root(x=w395) -> (sqrt(x)=w411:dbl)
    n112 = Square Root(x=w406) -> (sqrt(x)=w410:dbl)
    n113 = Multiply(x=w315, y="AY kappa") -> (x*y=w311:dbl)
    n114 = Multiply(x=w316, y="BY kappa") -> (x*y=w312:dbl)
    n115 = Subtract(x=w361, y="Fixed Y") -> (x-y=w396:dbl)
    n116 = Subtract(x=w362, y="Fixed X") -> (x-y=w401:dbl)
    n117 = Cluster To Array(cluster=w289) -> (array=w288:string[])
    n118 = for {
      tunnel: w148 -> [w443] mode=indexing
      tunnel: w128 -> [_]
      tunnel: "Downsamp\nfact" -> [w448]
      tunnel: [w446] -> w204 mode=indexing
      tunnel: w298 -> [w450]
      tunnel: w288 -> [w445] mode=indexing
      tunnel: "NI_ChannelName" ("name") -> [w444]
      n119 = call "Downsample 1D array.vi"("Ave N"=w448, "Arrray In"=w443) -> ("Array Out"=w449:dbl[])  [unwired: 9 in]
      n120 = Bundle By Name("Y"=w449, "dt"="dt", "t0"=w450) -> (w447:waveform(dbl))  [unwired: 1 in]
      n121 = Set Waveform Attribute(5:w445, 6:w444, 7:w447) -> (3:w446:waveform(dbl))  [unwired: 1 in, 2 out]
    }
    "All signals" <- w204
    n122 = Square(x=w311) -> (x^2=w384:dbl)
    n123 = Square(x=w309) -> (x^2=w385:dbl)
    n124 = Square(x=w312) -> (x^2=w386:dbl)
    n125 = Square(x=w310) -> (x^2=w387:dbl)
    n126 = Add(x=w384, y=w385) -> (x+y=w388:dbl)
    n127 = Add(x=w386, y=w387) -> (x+y=w389:dbl)
    n128 = Multiply(x=w396, y="Conv Y (nm/V)") -> (x*y=w318:dbl)
    n129 = Multiply(x=w401, y="Conv X (nm/V)") -> (x*y=w319:dbl)
    n130 = feedback #2() -> (w356:cluster{"B_Y":dbl, "B_X":dbl})  [unwired: 1 in]
    n131 = case shown="True" "Force Feedback" {
      tunnel: [w734 w750] -> w415
      tunnel: [w733 w749] -> w423
      tunnel: w117 -> [_ w748]
      tunnel: [cluster{"B_Y":dbl, "B_X":dbl} {"B_Y"=0.0, "B_X"=0.0} ("Sum error past") w740] -> w357
      tunnel: w356 -> [_ w747]
      tunnel: w416 -> [w734 w743]
      tunnel: w421 -> [w733 w742]
      frame False {
        # "Force feedback"
      }
      frame True {
        n132 = call "ForceFeedback2.vi"("PSD/Mirror Voltages"=w748, "Sum error"=w747, "task/channels in"=w743, "error in"=w742, "Desired voltage"="Setpoint voltage", "Feedback const"="Feedback const", "offset"="Offset") -> ("task out"=w750:refnum<k21>, "Sum error past"=w740:cluster{"B_Y":dbl, "B_X":dbl}, "Output Voltage"=→"Feedback Output Voltage 2":cluster{dbl, dbl}, "error out"=w749:errorcluster)  [unwired: 8 in, 1 out]
        n133 = local read "Pulling direction"() -> (w739:bool)
        n134 = Unbundle(w740) -> ("B_Y"=w737:dbl, "B_X"=w736:dbl)
        n135 = Select(t=w737, s=w739, f=w736) -> (s? t:f=→"Sum error":dbl)
      }
    }
    n136 = feedback-in #2(w357) -> ()
    n137 = Square Root(x=w388) -> (sqrt(x)=w317:dbl)
    n138 = Square Root(x=w389) -> (sqrt(x)=w412:dbl)
    n139 = Add(x=w317, y=w412) -> (x+y=w390:dbl)
    n140 = Build Array(w399, w400, w407, w408, w365, w364, w317, w412, w411, w410, w319, w318) -> ()  [unwired: 1 out]
    n141 = Divide(x=w390, y=2.0) -> (x/y=w354:dbl)
    n142 = Index Array(array=w204, index=6) -> (element=w153:waveform(dbl))
    n143 = Index Array(array=w204, index=7) -> (element=w155:waveform(dbl))
    n144 = local read "Fixed X"() -> (w208:dbl)
    n145 = local read "Fixed Y"() -> (w210:dbl)
    n146 = Unbundle By Name(w153) -> ("Y"=w212:dbl[])
    n147 = Unbundle By Name(w155) -> ("Y"=w211:dbl[])
    n148 = Index Array(array=w204, index=0) -> (element=w161:waveform(dbl))
    n149 = Index Array(array=w204, index=1) -> (element=w285:waveform(dbl))
    n150 = Index Array(array=w204, index=4) -> (element=w279:waveform(dbl))
    n151 = Subtract(x=w212, y=w208) -> (x-y=w209:dbl[])
    n152 = Subtract(x=w211, y=w210) -> (x-y=w206:dbl[])
    n153 = Unbundle By Name(w161) -> ("Y"=w277:dbl[])
    n154 = Unbundle By Name(w285) -> ("Y"=w276:dbl[])
    n155 = Unbundle By Name(w279) -> ("Y"=w275:dbl[])
    n156 = Index Array(array=w204, index=5) -> (element=w278:waveform(dbl))
    n157 = local read "Conv X (nm/V)"() -> (w207:dbl)
    n158 = local read "Conv Y (nm/V)"() -> (w205:dbl)
    n159 = Index Array(array=w204, index=2) -> (element=w158:waveform(dbl))
    n160 = Index Array(array=w204, index=3) -> (element=w282:waveform(dbl))
    n161 = Set Waveform Attribute(5:"T2 X", 6:w151, 7:w153) -> (3:w152:waveform(dbl))  [unwired: 1 in, 2 out]
    n162 = Set Waveform Attribute(5:"T2 Y", 6:w151, 7:w155) -> (3:w154:waveform(dbl))  [unwired: 1 in, 2 out]
    n163 = Unbundle By Name(w278) -> ("Y"=w272:dbl[])
    n164 = Unbundle By Name(w158) -> ("Y"=w274:dbl[])
    n165 = Unbundle By Name(w282) -> ("Y"=w273:dbl[])
    n166 = local read "Saving"() -> (w320:bool)
    n167 = local read "Tether"() -> (w321:bool)
    n168 = Divide(x=w277, y=w275) -> (x/y=w176:dbl[])
    n169 = Divide(x=w276, y=w275) -> (x/y=w174:dbl[])
    n170 = local read "AY offset"() -> (w263:dbl)
    n171 = local read "AX offset"() -> (w261:dbl)
    n172 = Multiply(x=w209, y=w207) -> (x*y=w145:dbl[])
    n173 = Multiply(x=w206, y=w205) -> (x*y=w147:dbl[])
    n174 = Less?(x=w354, y="Tether break\nforce (pN)") -> (x < y?=w352:bool)
    n175 = Divide(x=w273, y=w272) -> (x/y=w175:dbl[])
    n176 = Subtract(x=w174, y=w261) -> (x-y=w264:dbl[])
    n177 = local read "BY offset"() -> (w268:dbl)
    n178 = local read "BX offset"() -> (w271:dbl)
    n179 = Subtract(x=w176, y=w263) -> (x-y=w265:dbl[])
    n180 = Divide(x=w274, y=w272) -> (x/y=w177:dbl[])
    n181 = local read "AY alpha"() -> (w262:dbl)
    n182 = local read "AX alpha"() -> (w260:dbl)
    n183 = Compound Arithmetic op=AND(w320, w321, w352) -> (w351:bool)
    n184 = call-poly <vilib>:"Mean.vi"("X"=w147) -> ("mean"=w187:dbl)  [unwired: 1 out]
    "Mean Trp Pos Y 2 (nm)" <- w187
    n185 = Subtract(x=w177, y=w176) -> (x-y=w173:dbl[])
    n186 = Subtract(x=w175, y=w174) -> (x-y=w172:dbl[])
    n187 = Subtract(x=w145, y="Offset X (nm)") -> (x-y=w144:dbl[])
    n188 = Subtract(x=w147, y="Offset Y (nm)") -> (x-y=w146:dbl[])
    n189 = Subtract(x=w177, y=w268) -> (x-y=w270:dbl[])
    n190 = Subtract(x=w175, y=w271) -> (x-y=w269:dbl[])
    n191 = Subtract(x=w187, y=w147) -> (x-y=w186:dbl[])
    n192 = call-poly <vilib>:"Mean.vi"("X"=w145) -> ("mean"=w191:dbl)  [unwired: 1 out]
    "Mean Trap Pos X 2 (nm)" <- w191
    n193 = Build Array(w173, w172) -> (w170:dbl[][])
    n194 = Index Array(array=w170, index (row)=0) -> (element=w168:dbl[])  [unwired: 1 in]
    n195 = Index Array(array=w170, index (row)=1) -> (element=w167:dbl[])  [unwired: 1 in]
    n196 = call-poly <vilib>:"Mean.vi"("X"=w168) -> ("mean"=w166:dbl)  [unwired: 1 out]
    n197 = call-poly <vilib>:"Mean.vi"("X"=w167) -> ("mean"=w165:dbl)  [unwired: 1 out]
    n198 = Bundle("mean"=w166, "mean"=w165) -> ()  [unwired: 1 in, 1 out]
    n199 = local read "BY alpha"() -> (w267:dbl)
    n200 = local read "BX alpha"() -> (w266:dbl)
    n201 = Multiply(x=w265, y=w262) -> (x*y=w253:dbl[])
    n202 = Multiply(x=w264, y=w260) -> (x*y=w252:dbl[])
    n203 = Square(x=w186) -> (x^2=w185:dbl[])
    n204 = Subtract(x=w191, y=w145) -> (x-y=w190:dbl[])
    n205 = Bundle By Name(cluster=w154, "Y"=w146) -> (w202:waveform(dbl))
    n206 = case shown="True" w351 {
      selector: w351 -> [_ w469]
      frame False {
      }
      frame True {
        n207 = call <vilib>:"Beep.vi"() -> ()  [unwired: 12 in]
        n208 = Not(x=w469) -> (.not. x?=w467:bool)
        n209 = local write "Tether"(w467) -> ()
        n210 = local write "Force Feedback"(w467) -> ()
        n211 = property on="Stop saving" class="Bool (strict)"("Val(Sgnl)"="TA Cancel Save?") -> ()  [unwired: 2 in, 2 out]
      }
    }
    n212 = Bundle By Name(cluster=w152, "Y"=w144) -> (w203:waveform(dbl))
    n213 = Square(x=w190) -> (x^2=w189:dbl[])
    n214 = call-poly <vilib>:"Mean.vi"("X"=w185) -> ("mean"=w184:dbl)  [unwired: 1 out]
    n215 = Square(x=w253) -> (x^2=w259:dbl[])
    n216 = Multiply(x=w270, y=w267) -> (x*y=w251:dbl[])
    n217 = Square(x=w252) -> (x^2=w258:dbl[])
    n218 = Multiply(x=w269, y=w266) -> (x*y=w250:dbl[])
    n219 = call-poly <vilib>:"Mean.vi"("X"=w189) -> ("mean"=w188:dbl)  [unwired: 1 out]
    n220 = Build Array(w203, w202) -> (w108:waveform(dbl)[])
    "Trap sep" <- w108
    n221 = local read "Flushing Sample"() -> (w113:bool)
    n222 = Square Root(x=w184) -> (sqrt(x)=w183:dbl)
    n223 = Square(x=w251) -> (x^2=w257:dbl[])
    n224 = Square(x=w250) -> (x^2=w256:dbl[])
    n225 = Add(x=w259, y=w258) -> (x+y=w255:dbl[])
    n226 = Square Root(x=w188) -> (sqrt(x)=w181:dbl)
    n227 = Multiply(x=w183, y=10) -> (x*y=→"T2 Y RMS (A)":dbl)
    n228 = Square Root(x=w255) -> (sqrt(x)=w140:dbl[])
    n229 = Add(x=w257, y=w256) -> (x+y=w254:dbl[])
    n230 = Set Waveform Attribute(5:"T2", 6:"NI_ChannelName" ("name"), 7:w161) -> (3:w160:waveform(dbl))  [unwired: 1 in, 2 out]
    n231 = Set Waveform Attribute(5:"T1", 6:"NI_ChannelName" ("name"), 7:w158) -> (3:w157:waveform(dbl))  [unwired: 1 in, 2 out]
    n232 = Square Root(x=w254) -> (sqrt(x)=w139:dbl[])
    n233 = Multiply(x=w181, y=10) -> (x*y=→"T2 X RMS (A)":dbl)
    n234 = Bundle By Name(cluster=w160, "Y"=w140) -> (w164:waveform(dbl))
    n235 = case shown="True" w113 {
      frame False {
      }
      frame True {
        n236 = local read "Flush Sample Start Time"() -> (w434:u32)
        n237 = local read "Sample flush time (s)"() -> (w427:dbl)
        n238 = Tick Count (ms)() -> (millisecond timer value=w435:u32)
        n239 = Subtract(x=w435, y=w434) -> (x-y=w425:u32)
        n240 = Multiply(x=u32 1000, y=w427) -> (x*y=w426:dbl)
        n241 = Divide(x=w425, y=w426) -> (x/y=w430:dbl)
        n242 = Greater?(x=w425, y=w426) -> (0:w433:bool)
        n243 = Not(x=w433) -> (.not. x?=w432:bool)
        n244 = Boolean To (0,1)(Boolean=w432) -> (0, 1=w431:i16)
        n245 = Compound Arithmetic op=MULTIPLY(w431, w430, 100.0 ("value")) -> (→"Sample Flush Meter":dbl)
        n246 = case shown="True" w433 {
          frame False {
          }
          frame True {
            w437 = FALSE ("Inject Sample")
            n247 = property on="Clear Volume" class="Bool (strict)"("Val(Sgnl)"=TRUE ("Value (Signaling)")) -> ()  [unwired: 2 in, 2 out]
            n248 = local write "Inject Sample"(w437) -> ()
            n249 = local write "Flushing Sample"(w437) -> ()
          }
        }
      }
    }
    n250 = Bundle By Name(cluster=w157, "Y"=w139) -> (w232:waveform(dbl))
    n251 = Add(x=w140, y=w139) -> (x+y=w138:dbl[])
    n252 = case shown="True" "Remove offsets" {
      selector: "Remove offsets" -> [_ w440]
      frame False {
      }
      frame True {
        n253 = local read "Mean Trp Pos Y 2 (nm)"() -> (w438:dbl)
        n254 = Not(x=w440) -> (.not. x?=w441:bool)
        n255 = local read "Mean Trap Pos X 2 (nm)"() -> (w439:dbl)
        n256 = local write "Remove offsets"(w441) -> ()
        n257 = local write "Offset Y (nm)"(w438) -> ()
        n258 = local write "Offset X (nm)"(w439) -> ()
      }
    }
    n259 = Build Array(w164, w232) -> (→"Bead sep":waveform(dbl)[])
    n260 = local read "AY kappa"() -> (w249:dbl)
    n261 = local read "AX kappa"() -> (w248:dbl)
    n262 = Divide(x=w138, y=2) -> (x/y=w136:dbl[])
    n263 = local read "BX kappa"() -> (w246:dbl)
    n264 = local read "BY kappa"() -> (w247:dbl)
    n265 = call-poly <vilib>:"Mean.vi"("X"=w136) -> ("mean"=w135:dbl)  [unwired: 1 out]
    "Mean Bead Sep\n(nm)" <- w135
    n266 = local read "Calibrating"() -> (w413:bool)
    n267 = Multiply(x=w253, y=w249) -> (x*y=w242:dbl[])
    n268 = Multiply(x=w252, y=w248) -> (x*y=w243:dbl[])
    n269 = Square(x=w242) -> (x^2=w241:dbl[])
    n270 = Square(x=w243) -> (x^2=w240:dbl[])
    n271 = Subtract(x=w136, y=w135) -> (x-y=w134:dbl[])
    n272 = Multiply(x=w251, y=w247) -> (x*y=w244:dbl[])
    n273 = Multiply(x=w250, y=w246) -> (x*y=w245:dbl[])
    n274 = Add(x=w241, y=w240) -> (x+y=w237:dbl[])
    n275 = Square(x=w134) -> (x^2=w133:dbl[])
    n276 = Square Root(x=w237) -> (sqrt(x)=w201:dbl[])
    n277 = Square(x=w244) -> (x^2=w239:dbl[])
    n278 = Square(x=w245) -> (x^2=w238:dbl[])
    n279 = call-poly <vilib>:"Mean.vi"("X"=w133) -> ("mean"=w132:dbl)  [unwired: 1 out]
    n280 = Add(x=w239, y=w238) -> (x+y=w236:dbl[])
    n281 = Bundle By Name(cluster=w160, "Y"=w201) -> (w235:waveform(dbl))
    n282 = local read "Saving"() -> (w350:bool)
    n283 = Or(x=w413, y=w350) -> ()  [unwired: 1 out]
    n284 = Square Root(x=w132) -> (sqrt(x)=w131:dbl)
    n285 = Square Root(x=w236) -> (sqrt(x)=w200:dbl[])
    n286 = And(x="Save scans", y="Raster scan") -> (x .and. y?=w111:bool)
    n287 = Multiply(x=10, y=w131) -> (x*y=→"Bead Sep Noise\n(A)":dbl)
    n288 = Bundle By Name(cluster=w157, "Y"=w200) -> (w234:waveform(dbl))
    n289 = Add(x=w201, y=w200) -> (x+y=w199:dbl[])
    n290 = Build Array(w235, w234) -> (→"Force (pN)":waveform(dbl)[])
    n291 = flat-sequence {
      tunnel: w413 -> [w509]
      tunnel: w350 -> [_]
      tunnel: w413 -> [_]
      tunnel: w350 -> [_]
      tunnel: w148 -> [w496]
      tunnel: [w496] -> w371
      tunnel: w230 -> [w495]
      tunnel: [w495] -> w370
      tunnel: w358 -> [w494]
      tunnel: [w494] -> w363
      tunnel: w360 -> [w493]
      tunnel: [w493] -> w359
      tunnel: [w490] -> w349
      tunnel: [w487] -> w348
      tunnel: [w484] -> w217
      tunnel: [w483] -> w216
      tunnel: [w480] -> w215
      tunnel: w111 -> [w477]
      tunnel: ["Save Data"] -> w109
      tunnel: w371 -> [w656]
      tunnel: w370 -> [w655]
      tunnel: w363 -> [_]
      tunnel: w359 -> [_]
      tunnel: w349 -> [w654]
      tunnel: w348 -> [w653]
      tunnel: w217 -> [w652]
      tunnel: w216 -> [w651]
      tunnel: w215 -> [w650]
      tunnel: w109 -> [w648]
      tunnel: w108 -> [w647]
      frame #0 {
        w475 = 0.0
        # "1: old trap\n0: fleezers"
        # "Create files if saving data"
        n292 = local read "Save N sets"() -> (w479:bool)
        n293 = local read "Sampling Rate"() -> (w507:dbl)
        n294 = Or(x=w479, y="Save Data") -> (x .or. y?=w478:bool)
        n295 = Build Array(w478, "Save cal", w477) -> (w498:bool[])
        n296 = Compound Arithmetic op=OR("Save Data", "Save cal", w477) -> (w500:bool)
        n297 = Boolean Array To Number(Boolean array=w498) -> (number=w497:u32)
        n298 = local read "Trap position"() -> (w504:cluster{"X":dbl, "Y":dbl})
        n299 = local read "Fixed X"() -> (w474:dbl)
        n300 = local read "Fixed Y"() -> (w473:dbl)
        n301 = Unbundle(w504) -> ("X"=w472:dbl, "Y"=w471:dbl)
        n302 = Build Array(w472, w471, w474, w473, w475, w475) -> (w503:dbl[])
        n303 = feedback #3(refnum<k0> refnum) -> (w488:refnum<file>)
        n304 = feedback #4() -> (w485:dbl)  [unwired: 1 in]
        n305 = feedback #5(FALSE) -> (w481:bool)
        n306 = feedback #6(0) -> (w501:i32)
        n307 = feedback #7(refnum<k0> refnum) -> (w491:refnum<file>)
        n308 = case shown="True" w500 {
          tunnel: w509 -> [_ _]
          tunnel: 9 -> [_ w551]
          tunnel: w507 -> [_ w550]
          tunnel: 6 -> [_ w549]
          tunnel: 5 -> [_ w548]
          tunnel: w503 -> [_ w547]
          tunnel: [w514 1] -> w484
          tunnel: w501 -> [w515 _]
          tunnel: w497 -> [_ w522]
          tunnel: [w513 w520] -> w490
          tunnel: w491 -> [w513 _]
          tunnel: [w512 w519] -> w487
          tunnel: w488 -> [w512 _]
          tunnel: 1.0 -> [_ w518]
          tunnel: [w511 w517] -> w483
          tunnel: w485 -> [w511 _]
          tunnel: [w510 w516] -> w480
          tunnel: w481 -> [w510 _]
          frame False {
            n309 = Increment(x=w515) -> (x+1=w514:i32)
          }
          frame True {
            w523 = FALSE ("Save Data")
            w529 = FALSE
            w530 = T10."big-endian, network order" ("byte order (0:big-endian, network order)")
            n310 = local write "Save cal"(w523) -> ()
            n311 = local write "Save Data"(w523) -> ()
            n312 = case shown="4" w522 {
              tunnel: w551 -> [w598 w616 w646]
              tunnel: w550 -> [w576 w615 w621]
              tunnel: w549 -> [w597 w613 w642]
              tunnel: w548 -> [w596 w612 w641]
              tunnel: w547 -> [w594 w609 w638]
              tunnel: [w593 w608 w627] -> w544
              tunnel: [w595 w605 w626] -> w516
              tunnel: ["Averaging Number" 200 w624] -> _
              tunnel: w518 -> [w581 w600 w623]
              tunnel: [w577 "Cal sets to save" w618] -> w517
              frame 1, Default {
                w595 = TRUE
                w582 = 0.0
                # "Time trace"
                n313 = local read "Averaging Number"() -> (w592:i32)
                n314 = Boolean To (0,1)(Boolean=w595) -> (0, 1=w587:i16)
                n315 = Increment(x=w587) -> (x+1=w586:i16)
                n316 = Divide(x=w576, y=w592) -> (x/y=w591:dbl)
                n317 = To Double Precision Float(number=w586) -> (double precision float=w585:dbl)
                n318 = Reciprocal(x=w591) -> (1/x=w590:dbl)
                n319 = Reciprocal(x=w576) -> (1/x=w575:dbl)
                n320 = Build Array(w598, w575, w590, w597, w596, 0 ("f")) -> (w589:dbl[])
                n321 = Build Array(w585, w581, w582, w582, w582) -> (w588:dbl[])
                n322 = Build Array (concatenate)(w589, w594, w588) -> (w593:dbl[])
                n323 = Select(t="N sets", s="Save N sets", f=2147483647) -> (s? t:f=w577:i32)
              }
              frame 2 {
                w605 = FALSE
                w603 = 0.0
                # "Calibration file"
                n324 = Reciprocal(x=w615) -> (1/x=w614:dbl)
                n325 = Boolean To (0,1)(Boolean=w605) -> (0, 1=w607:i16)
                n326 = To Double Precision Float(number=w607) -> (double precision float=w606:dbl)
                n327 = Build Array(w616, w614, w614, w613, w612, 1) -> (w610:dbl[])
                n328 = Build Array(w606, w600, w603, w603, w603) -> (w604:dbl[])
                n329 = Build Array (concatenate)(w610, w609, w604) -> (w608:dbl[])
                "Calibrating" <- TRUE ("Calibrating")
              }
              frame 4 {
                w634 = 0.0
                w626 = TRUE
                # "Not using ncycles"
                # "FX curve"
                n330 = local read "Averaging Number"() -> (w645:i32)
                n331 = Boolean To (0,1)(Boolean=w626) -> (0, 1=w637:i16)
                n332 = Increment(x=w637) -> (x+1=w636:i16)
                n333 = local write "Raster scan"(FALSE ("Raster scan")) -> ()
                n334 = To Double Precision Float(number=w636) -> (double precision float=w635:dbl)
                n335 = Divide(x=w621, y=w645) -> (x/y=w644:dbl)
                n336 = Reciprocal(x=w644) -> (1/x=w643:dbl)
                n337 = Build Array(w635, w623, w634, w634, w634) -> (w633:dbl[])
                n338 = Reciprocal(x=w621) -> (1/x=w620:dbl)
                n339 = Build Array(w646, w620, w643, w642, w641, 2) -> (w639:dbl[])
                n340 = local read "Pulling direction"() -> (w631:bool)
                n341 = local read "Scan range (V)"() -> (w617:dbl)
                n342 = local read "Scan steps (mirror)"() -> (w619:u64)
                n343 = local read "# scans"() -> (w629:i32)
                n344 = Not(x=w631) -> (.not. x?=w630:bool)
                n345 = local read "N sets to be saved"() -> (w618:dbl)
                n346 = local read "Averaging Number"() -> (w624:i32)
                n347 = Boolean To (0,1)(Boolean=w630) -> (0, 1=w632:i16)
                n348 = Build Array(w632, w617, w619, 0, w629) -> (w628:dbl[])
                n349 = Build Array (concatenate)(w639, w638, w633, w628) -> (w627:dbl[])
              }
            }
            n350 = call "CreateSaveFile.vi"("Index In"="Save file index", "Ext"=".dat", "Insert"="", "Directory"="Path") -> ("Path Out"=w528:path)  [unwired: 6 in, 1 out]
            "Current file name" <- w528
            n351 = Open/Create/Replace File(file path (use dialog)=w528, operation (0:open)=T9."create", access (0:read/write)=enum16{"read/write", "read-only", "write-only"}."write-only") -> (refnum out=w537:refnum<file>, error out=w538:errorcluster)  [unwired: 3 in, 1 out]
            n352 = Array Size(array=w544) -> (size(s)=w546:i32)
            n353 = case shown="True" w516 {
              tunnel: w528 -> [_ w574]
              tunnel: [refnum<k0> refnum w553] -> w519
              frame False {
              }
              frame True {
                w560 = 0.0
                n354 = Path To String(path=w574) -> (string=w570:string)
                n355 = Build Array(w560, w560, w560, w560, w560, w560, w560, w560) -> (w557:dbl[])
                n356 = String Length(string=w570) -> (length=w573:i32)
                n357 = Array Size(array=w557) -> (size(s)=w559:i32)
                n358 = Subtract(x=w573, y=4) -> (x-y=w571:i32)
                n359 = To Double Precision Float(number=w559) -> (double precision float=w558:dbl)
                n360 = String Subset(string=w570, length (rest)=w571) -> (substring=w569:string)  [unwired: 1 in]
                n361 = Build Array (concatenate)(w558, w557) -> (w556:dbl[])
                n362 = Concatenate Strings(w569, "_pos.dat" ("string")) -> (w567:string)
                n363 = String To Path(string=w567) -> (path=w566:path)
                n364 = Open/Create/Replace File(file path (use dialog)=w566, operation (0:open)=T9."create", access (0:read/write)=enum16{"read/write", "read-only", "write-only"}."write-only") -> (refnum out=w562:refnum<file>, error out=w563:errorcluster)  [unwired: 3 in, 1 out]
                n365 = Deny Access(4:w563, 7:w562) -> (3:w561:refnum<file>)  [unwired: 1 in, 1 out]
                n366 = Write to Binary File(file (use dialog)=w561, data=w556, 5:FALSE ("prepend array or string size? (T)"), 9:T10."big-endian, network order" ("byte order (0:big-endian, network order)")) -> (refnum out=w553:refnum<file>)  [unwired: 2 in, 2 out]
              }
            }
            n367 = Deny Access(4:w538, 7:w537) -> (0:w527:errorcluster, 3:w536:refnum<file>)  [unwired: 1 in]
            n368 = String Length(string="Comment") -> (length=w543:i32)
            n369 = To Double Precision Float(number=w546) -> (double precision float=w545:dbl)
            n370 = To Double Precision Float(number=w543) -> (double precision float=w542:dbl)
            n371 = Build Array (concatenate)(w545, w544, w542) -> (w533:dbl[])
            n372 = Write to Binary File(file (use dialog)=w536, data=w533, error in=w527, 5:w529, 9:w530) -> (refnum out=w532:refnum<file>, error out=w526:errorcluster)  [unwired: 1 in, 1 out]
            n373 = Write to Binary File(file (use dialog)=w532, data="Comment", error in=w526, 5:w529, 9:w530) -> (refnum out=w520:refnum<file>)  [unwired: 1 in, 2 out]
            "Saving" <- TRUE
          }
        }
        n374 = feedback-in #3(w487) -> ()
        n375 = feedback-in #4(w483) -> ()
        n376 = feedback-in #5(w480) -> ()
        n377 = feedback-in #6(w484) -> ()
        n378 = feedback-in #7(w490) -> ()
      }
      frame #1 {
        n379 = local read "Saving"() -> (w649:bool)
        n380 = case shown="True" w649 {
          tunnel: w656 -> [_ w675]
          tunnel: w655 -> [_ w674]
          tunnel: w654 -> [_ w673]
          tunnel: w653 -> [_ w672]
          tunnel: w652 -> [_ w662]
          tunnel: w651 -> [_ w663]
          tunnel: w650 -> [_ w666]
          tunnel: w648 -> [_ w658]
          tunnel: w647 -> [_ w657]
          frame False {
            (unwired) FALSE ("Calibrating")
          }
          frame True {
            n381 = local read "Stop"() -> (w670:bool)
            n382 = Less Or Equal?(x=w662, y=w663) -> (x <= y?=w671:bool)
            n383 = Divide(x=w662, y=w663) -> (x/y=w661:dbl)
            n384 = Or(x=w670, y="Stop saving") -> (x .or. y?=w669:bool)
            n385 = Not(x=w669) -> (.not. x?=w668:bool)
            n386 = Multiply(x=100.0, y=w661) -> (x*y=w660:dbl)
            n387 = And(x=w671, y=w668) -> (x .and. y?=w667:bool)
            n388 = case shown="True" w667 {
              tunnel: w673 -> [w680 w689]
              tunnel: w674 -> [_ w688]
              tunnel: w675 -> [_ w687]
              tunnel: w672 -> [w679 w686]
              tunnel: w666 -> [w677 _]
              tunnel: [0.0 ("Progress") w685] -> w665
              tunnel: w660 -> [_ w685]
              tunnel: w658 -> [_ w682]
              tunnel: w657 -> [_ w683]
              frame False {
                w678 = FALSE
                n389 = Close File(refnum=w680) -> ()  [unwired: 1 in, 2 out]
                n390 = case shown="True" w677 {
                  tunnel: w679 -> [_ w681]
                  frame False {
                  }
                  frame True {
                    n391 = Close File(refnum=w681) -> ()  [unwired: 1 in, 2 out]
                  }
                }
                n392 = call <vilib>:"Beep.vi"() -> ()  [unwired: 12 in]
                n393 = local write "Saving"(w678) -> ()
                n394 = local write "Stop saving"(w678) -> ()
                n395 = local write "Calibrating"(w678) -> ()
              }
              frame True {
                n396 = local read "Calibrating"() -> (w684:bool)
                n397 = case shown="False" w684 {
                  tunnel: w689 -> [w716 w732]
                  tunnel: w688 -> [_ w731]
                  tunnel: w687 -> [w703 w725]
                  tunnel: w686 -> [w702 _]
                  tunnel: w683 -> [w694 _]
                  tunnel: w682 -> [_ _]
                  frame False {
                    n398 = local read "Averaging Number"() -> (w710:i32)
                    n399 = Array Subset(array=w703, index (row)=0 ("index"), length (row)=6 ("length")) -> (w699:dbl[][])  [unwired: 2 in]
                    n400 = Array Subset(array=w703, index (row)=6 ("index"), length (row)=2 ("length")) -> (w698:dbl[][])  [unwired: 2 in]
                    n401 = Array Size(array=w698) -> (size(s)=w709:i32[])
                    n402 = Array Size(array=w699) -> (size(s)=w706:i32[])
                    n403 = Index Array(array=w694, index=0) -> (element=w691:waveform(dbl))
                    n404 = Index Array(array=w694, index=1) -> (element=w690:waveform(dbl))
                    n405 = for {
                      tunnel: w699 -> [w720] mode=indexing
                      tunnel: w710 -> [w722]
                      tunnel: [w721] -> w697 mode=indexing
                      n406 = call "Downsample 1D array.vi"("Ave N"=w722, "Arrray In"=w720) -> ("Array Out"=w721:dbl[])  [unwired: 9 in]
                    }
                    n407 = Unbundle By Name(w691) -> ()  [unwired: 1 out]
                    n408 = Unbundle By Name(w690) -> ()  [unwired: 1 out]
                    n409 = Multiply Array Elements(1:w706) -> (0:w705:i32)
                    n410 = for {
                      tunnel: w698 -> [w719] mode=indexing
                      tunnel: w710 -> [w718]
                      tunnel: [w717] -> w701 mode=indexing
                      n411 = call "Downsample 1D array.vi"("Ave N"=w718, "Arrray In"=w719) -> ("Array Out"=w717:dbl[])  [unwired: 9 in]
                    }
                    n412 = Multiply Array Elements(1:w709) -> (0:w708:i32)
                    n413 = Divide(x=w705, y=w710) -> (x/y=w711:dbl)
                    n414 = Divide(x=w708, y=w710) -> (x/y=w707:dbl)
                    n415 = Transpose 2D Array(2D array=w697) -> (transposed array=w696:dbl[][])
                    n416 = Transpose 2D Array(2D array=w701) -> (transposed array=w695:dbl[][])
                    n417 = Reshape Array(w696, w711) -> (w700:dbl[])
                    n418 = Reshape Array(w695, w707) -> (w704:dbl[])
                    n419 = call <vilib>:"Write File+ [SGL].vi"("1D array"=w704, "refnum"=w702) -> ()  [unwired: 7 in, 3 out]
                    n420 = call <vilib>:"Write File+ [SGL].vi"("1D array"=w700, "refnum"=w716) -> ()  [unwired: 7 in, 3 out]
                  }
                  frame True {
                    n421 = Array Subset(array=w725, index (row)=0 ("index"), length (row)=6 ("length")) -> (w723:dbl[][])  [unwired: 2 in]
                    n422 = Transpose 2D Array(2D array=w723) -> (transposed array=w729:dbl[][])
                    n423 = Array Size(array=w723) -> (size(s)=w724:i32[])
                    n424 = Multiply Array Elements(1:w724) -> (0:w730:i32)
                    n425 = Reshape Array(w729, w730) -> (w728:dbl[])
                    n426 = call <vilib>:"Write File+ [SGL].vi"("1D array"=w728, "error in (no error)"=w731, "refnum"=w732) -> ()  [unwired: 6 in, 3 out]
                  }
                }
              }
            }
            "Progress" <- w665
          }
        }
      }
    }
    n427 = Divide(x=w199, y=2) -> (x/y=w196:dbl[])
    n428 = call-poly <vilib>:"Mean.vi"("X"=w196) -> ("mean"=w197:dbl)  [unwired: 1 out]
    "Mean force (pN)" <- w197
    n429 = Subtract(x=w197, y=w196) -> (x-y=w195:dbl[])
    n430 = Square(x=w195) -> (x^2=w194:dbl[])
    n431 = call-poly <vilib>:"Mean.vi"("X"=w194) -> ("mean"=w193:dbl)  [unwired: 1 out]
    n432 = Square Root(x=w193) -> (sqrt(x)=→"Force noise (pN)":dbl)
    n433 = local read "Stop"() -> (w420:bool)
  }
  n434 = local write "Progress"(u8 0 ("Progress")) -> ()
  n435 = local write "Calibrating"(FALSE ("Calibrating")) -> ()
  n436 = call "InitializeChamberImage.vi"() -> ("error out"=w101:errorcluster, "IMAQ Session Out"=w102:refnum<k11>, "Display Out"=w103:T7, "Acquired Image"=w9:T7)  [unwired: 8 in]
  n437 = node-c288(i64 10 ("Period"), 2 ("Processor")) -> (w15:T12)  [unwired: 2 in]
  n438 = timed-loop {
    tunnel: w103 -> [w760]
    tunnel: w102 -> [w759]
    tunnel: w101 -> [w758]
    tunnel: [w756] -> w100
    tunnel: [w755] -> w99
    timing: w15 -> [_]
    timing-out: [_] -> w14
    i -> [w757]
    stop <- w751 continue-if-true
    n439 = node-c288() -> ()  [unwired: 1 in, 1 out]
    n440 = call <vilib>:"IMAQ Copy Acquired Buffer.vi"("IMAQ Session In"=w759, "Image In"=w760, "Buffer Number"=w757, "error in (no error)"=w758) -> ("IMAQ Session Out"=w756:refnum<k11>, "Image Out"=→"Chamber":T7, "error out"=w755:errorcluster)  [unwired: 7 in, 2 out]
    "Video Error" <- w755
    n441 = local read "Stop"() -> (w753:bool)
    n442 = Unbundle By Name(w755) -> ("status"=w754:bool)
    n443 = Not Or(1:w753, 2:w754) -> (0:w751:bool)
    "Continue to display?" <- w751
    n444 = node-c288() -> ()  [unwired: 1 in, 1 out]
  }
  n445 = node-c288(w14) -> ()  [unwired: 1 out]
  n446 = call <vilib>:"IMAQ Close.vi"("error in (no error)"=w99, "IMAQ Session In"=w100) -> ("error out"=w107:errorcluster)  [unwired: 9 in]
  n447 = call "IMAQ Dispose"("error in (no error)"=w107) -> ("error out"=w106:errorcluster)  [unwired: 5 in]
  n448 = call-poly "VISA Configure Serial Port"("VISA resource name"=refnum<visa-resource-name> "COM3") -> ("VISA resource name out"=w21:refnum<visa-resource-name>, "error out"=w20:errorcluster)  [unwired: 13 in]
  n449 = node-c288(i64 100 ("Period"), 2 ("Processor")) -> (w23:T12)  [unwired: 2 in]
  n450 = call "IMAQ Dispose"("Image"=w9, "error in (no error)"=w106) -> ("error out"=w105:errorcluster)  [unwired: 4 in]
  n451 = timed-loop {
    timing: w23 -> [_]
    timing-out: [_] -> w22
    tunnel: w21 -> [w763]
    tunnel: w20 -> [w765]
    tunnel: [w763] -> w19
    stop <- w764 stop-if-true
    n452 = node-c288() -> ()  [unwired: 1 in, 1 out]
    n453 = event shown="[0] \"Got DNA bead\": Value Change" {
      selector: _ -> [_ _ _ _ _ _ _ _ _ _ _]
      dyn-events: _ -> [_ _ _ _ _ _ _ _ _ _ _]
      timeout: _ -> [_ _ _ _ _ _ _ _ _ _ _]
      tunnel: w763 -> [w772 w810 w830 w847 w864 w883 w903 _ _ _ _]
      tunnel: w765 -> [w771 w809 w829 w846 w863 w882 w902 _ _ _ _]
      tunnel: [_ _ _ _ _ _ _ _ _ _ w956] -> w764
      event "Got DNA bead": Value Change {
        n454 = event-data() -> ()  [unwired: 1 in, 5 out]
        n455 = flat-sequence {
          tunnel: w772 -> [w775]
          tunnel: w771 -> [w773]
          tunnel: [w790] -> w770
          tunnel: w770 -> [w793]
          tunnel: [w793] -> w769
          tunnel: w769 -> [w795]
          tunnel: [w795] -> w768
          tunnel: w768 -> [w799]
          tunnel: [w799] -> w767
          tunnel: w767 -> [w801]
          tunnel: [w801] -> w766
          tunnel: w766 -> [w803]
          frame #0 {
            n456 = local read "Saved stage positions"() -> (w776:dbl[][])
            n457 = disable-structure shown="Disabled" {
              frame Disabled {
                n458 = property on="Inject Pump 2" class="Bool (strict)"("Val(Sgnl)"=FALSE ("Inject Pump 2")) -> ()  [unwired: 2 in, 2 out]
              }
              frame Enabled {
              }
            }
            n459 = local write "Stage moving"(TRUE ("Stage moving")) -> ()
            n460 = property on="Trap delta" class="DigNum (strict)"("Val(Sgnl)"="Cal @ Delta (V)") -> ()  [unwired: 2 in, 2 out]
            n461 = call "move to saved stage position.vi"("error in"=w773, "Stage VISA resource name in"=w775, "Position"="Cal stage position", "Saved Stage Positions"=w776) -> ()  [unwired: 2 out]
          }
          frame #1 {
            n462 = local write "Stage moving"(FALSE ("Stage moving")) -> ()
            n463 = property on="Inject Sample" class="Bool (strict)"("Val(Sgnl)"=FALSE ("Value (Signaling)")) -> ()  [unwired: 2 in, 2 out]
            n464 = call <vilib>:"Beep.vi"() -> ()  [unwired: 12 in]
          }
          frame #2 {
            n465 = Wait (ms)(milliseconds to wait=u32 1000) -> ()  [unwired: 1 out]
          }
          frame #3 {
            n466 = property on="Save cal" class="Bool (strict)"("Val(Sgnl)"=TRUE ("Value (Signaling)")) -> ()  [unwired: 2 in, 2 out]
          }
          frame #4 {
            n467 = Wait (ms)(milliseconds to wait=u32 2000) -> ()  [unwired: 1 out]
          }
          frame #5 {
            n468 = while {
              stop <- w786 stop-if-true
              n469 = local read "Saving"() -> (w787:bool)
              n470 = Not(x=w787) -> (.not. x?=w786:bool)
              n471 = Wait (ms)(milliseconds to wait=u32 100) -> ()  [unwired: 1 out]
            }
          }
          frame #6 {
            n472 = Wait (ms)(milliseconds to wait=u32 2000) -> ()  [unwired: 1 out]
            n473 = property on="Trap delta" class="DigNum (strict)"("Val(Sgnl)"="Offset @ Delta (V)") -> ()  [unwired: 2 in, 2 out]
          }
          frame #7 {
            # "Only continue if there is no buffer\noverflow error"
            n474 = local read "Buffer Overflow"() -> (w791:bool)
            n475 = Not(x=w791) -> (.not. x?=w790:bool)
            n476 = case shown="True" w790 {
              frame False {
              }
              frame True {
                n477 = property on="Raster scan" class="Bool (strict)"("Val(Sgnl)"=TRUE ("Value (Signaling)")) -> ()  [unwired: 2 in, 2 out]
              }
            }
          }
          frame #8 {
            n478 = case shown="True" w793 {
              frame False {
              }
              frame True {
                n479 = Wait (ms)(milliseconds to wait=u32 2000) -> ()  [unwired: 1 out]
              }
            }
          }
          frame #9 {
            n480 = case shown="True" w795 {
              frame False {
              }
              frame True {
                n481 = while {
                  stop <- w797 stop-if-true
                  n482 = local read "Saving"() -> (w798:bool)
                  n483 = Not(x=w798) -> (.not. x?=w797:bool)
                  n484 = Wait (ms)(milliseconds to wait=u32 100) -> ()  [unwired: 1 out]
                }
              }
            }
          }
          frame #10 {
            n485 = case shown="True" w799 {
              frame False {
              }
              frame True {
                n486 = property on="Read Cal" class="Bool (strict)"("Val(Sgnl)"=TRUE ("Value (Signaling)")) -> ()  [unwired: 2 in, 2 out]
              }
            }
          }
          frame #11 {
            n487 = case shown="True" w801 {
              frame False {
              }
              frame True {
                n488 = Wait (ms)(milliseconds to wait=u32 1000) -> ()  [unwired: 1 out]
              }
            }
          }
          frame #12 {
            n489 = case shown="True" w803 {
              frame False {
              }
              frame True {
                n490 = property on="Fish" class="Bool (strict)"("Val(Sgnl)"=TRUE ("Value (Signaling)")) -> ()  [unwired: 2 in, 2 out]
                n491 = case shown="True" "Flow on\nwhile fish?" {
                  frame False {
                  }
                  frame True {
                    n492 = property on="Inject Sample" class="Bool (strict)"("Val(Sgnl)"=TRUE ("Value (Signaling)")) -> ()  [unwired: 2 in, 2 out]
                  }
                }
              }
            }
          }
        }
      }
      event "Dump beads": Value Change {
        n493 = event-data() -> ()  [unwired: 1 in, 5 out]
        n494 = flat-sequence {
          tunnel: w809 -> [w813]
          tunnel: w810 -> [w814]
          tunnel: [w814] -> w808
          tunnel: [w813] -> w807
          tunnel: w808 -> [w817]
          tunnel: w807 -> [w816]
          frame #0 {
            w811 = FALSE ("Fish")
            n495 = local read "Saving"() -> (w812:bool)
            n496 = local write "Pause dwell"(w811) -> ()
            n497 = local write "Force Feedback"(w811) -> ()
            n498 = local write "Dump beads"(w811) -> ()
            n499 = property on="Stop saving" class="Bool (strict)"("Val(Sgnl)"=w812) -> ()  [unwired: 2 in, 2 out]
            n500 = local write "Fish"(w811) -> ()
          }
          frame #1 {
            n501 = local read "Saved stage positions"() -> (w819:dbl[][])
            n502 = case shown="True" "Flow on\ndump?" {
              frame False {
              }
              frame True {
                n503 = property on="Inject Sample" class="Bool (strict)"("Val(Sgnl)"=TRUE ("Value (Signaling)")) -> ()  [unwired: 2 in, 2 out]
              }
            }
            n504 = local write "Stage moving"(TRUE ("Stage moving")) -> ()
            n505 = call "move to saved stage position.vi"("error in"=w816, "Stage VISA resource name in"=w817, "Position"=5, "Saved Stage Positions"=w819) -> ()  [unwired: 2 out]
          }
          frame #2 {
            n506 = local read "Shutter 1 (B)"() -> (w824:bool)
            n507 = local read "Shutter 2 (A)"() -> (w823:bool)
            n508 = call <vilib>:"Beep.vi"() -> ()  [unwired: 12 in]
            n509 = case shown="True" w824 {
              frame False {
              }
              frame True {
                n510 = property on="Shutter 1 (B)" class="Bool (strict)"("Val(Sgnl)"=FALSE ("Value (Signaling)")) -> ()  [unwired: 2 in, 2 out]
              }
            }
            n511 = case shown="True" w823 {
              frame False {
              }
              frame True {
                n512 = property on="Shutter 2 (A)" class="Bool (strict)"("Val(Sgnl)"=FALSE) -> ()  [unwired: 2 in, 2 out]
              }
            }
            n513 = local write "Stage moving"(FALSE ("Stage moving")) -> ()
            n514 = local write "Tether"(FALSE ("Tether")) -> ()
          }
          frame #3 {
            n515 = property on="Move Cap. 2 (ADig Top)" class="Bool (strict)"("Val(Sgnl)"=TRUE ("Value (Signaling)")) -> ()  [unwired: 2 in, 2 out]
          }
        }
      }
      event "Move Cap. 2 (ADig Top)": Value Change {
        n516 = event-data() -> ()  [unwired: 1 in, 5 out]
        n517 = flat-sequence {
          tunnel: w830 -> [w834]
          tunnel: w829 -> [w833]
          frame #0 {
            n518 = local read "Saved stage positions"() -> (w832:dbl[][])
            n519 = case shown="True" "Flow on\ncap 2?" {
              frame False {
              }
              frame True {
                n520 = property on="Inject Sample" class="Bool (strict)"("Val(Sgnl)"=TRUE ("Value (Signaling)")) -> ()  [unwired: 2 in, 2 out]
              }
            }
            n521 = local write "Move Cap. 2 (ADig Top)"(FALSE ("Move Cap. 2 (ADig Top)")) -> ()
            n522 = local write "Stage moving"(TRUE ("Stage moving")) -> ()
            n523 = call "move to saved stage position.vi"("error in"=w833, "Stage VISA resource name in"=w834, "Position"=2, "Saved Stage Positions"=w832) -> ()  [unwired: 2 out]
          }
          frame #1 {
            # "Make sure you don't reverse\nwhich is ON and OFF"
            n524 = local read "Cal @ Delta (V)"() -> (w841:dbl)
            n525 = local write "Stage moving"(FALSE ("Stage moving")) -> ()
            n526 = call <vilib>:"Beep.vi"() -> ()  [unwired: 12 in]
            n527 = property on="Trap delta" class="DigNum (strict)"("Val(Sgnl)"=w841) -> ()  [unwired: 2 in, 2 out]
            n528 = disable-structure shown="Disabled" {
              frame Disabled {
                n529 = property on="Inject Pump 1" class="Bool (strict)"("Val(Sgnl)"=TRUE ("Inject Pump 2")) -> ()  [unwired: 2 in, 2 out]
              }
              frame Enabled {
              }
            }
            n530 = local read "Shutter 2 (A)"() -> (w840:bool)
            n531 = case shown="False" w840 {
              frame False {
                n532 = property on="Shutter 2 (A)" class="Bool (strict)"("Val(Sgnl)"=TRUE ("Value (Signaling)")) -> ()  [unwired: 2 in, 2 out]
              }
              frame True {
              }
            }
            n533 = property on="Inject Sample" class="Bool (strict)"("Val(Sgnl)"=FALSE ("Value (Signaling)")) -> ()  [unwired: 2 in, 2 out]
          }
        }
      }
      event "Got ADig bead": Value Change {
        n534 = event-data() -> ()  [unwired: 1 in, 5 out]
        n535 = flat-sequence {
          tunnel: w847 -> [w851]
          tunnel: w846 -> [w850]
          frame #0 {
            n536 = local read "Saved stage positions"() -> (w853:dbl[][])
            n537 = property on="Inject Pump 1" class="Bool (strict)"("Val(Sgnl)"=FALSE ("Inject Pump 2")) -> ()  [unwired: 2 in, 2 out]
            n538 = case shown="True" "Flow on\ncap 1?" {
              frame False {
              }
              frame True {
                n539 = property on="Inject Sample" class="Bool (strict)"("Val(Sgnl)"=TRUE ("Value (Signaling)")) -> ()  [unwired: 2 in, 2 out]
              }
            }
            n540 = local write "Stage moving"(TRUE ("Stage moving")) -> ()
            n541 = call "move to saved stage position.vi"("error in"=w850, "Stage VISA resource name in"=w851, "Position"=1, "Saved Stage Positions"=w853) -> ()  [unwired: 2 out]
          }
          frame #1 {
            n542 = local read "Shutter 1 (B)"() -> (w857:bool)
            n543 = disable-structure shown="Disabled" {
              frame Disabled {
                n544 = property on="Inject Pump 2" class="Bool (strict)"("Val(Sgnl)"=TRUE ("Inject Pump 2")) -> ()  [unwired: 2 in, 2 out]
              }
              frame Enabled {
              }
            }
            n545 = local write "Stage moving"(FALSE ("Stage moving")) -> ()
            n546 = case shown="False" w857 {
              frame False {
                n547 = property on="Shutter 1 (B)" class="Bool (strict)"("Val(Sgnl)"=TRUE ("Value (Signaling)")) -> ()  [unwired: 2 in, 2 out]
              }
              frame True {
              }
            }
            n548 = property on="Inject Sample" class="Bool (strict)"("Val(Sgnl)"=FALSE ("Value (Signaling)")) -> ()  [unwired: 2 in, 2 out]
            n549 = call <vilib>:"Beep.vi"() -> ()  [unwired: 12 in]
          }
        }
        n550 = local write "Got ADig bead"(FALSE ("Got ADig bead")) -> ()
      }
      event "Set Position 1", "Set Position 2", "Set Position 3", "Set Position 4", "Set Position 5": Value Change {
        n551 = event-data() -> ()  [unwired: 1 in, 5 out]
        n552 = Build Array("Set Position 1", "Set Position 2", "Set Position 3", "Set Position 4", "Set Position 5") -> (w876:bool[])
        n553 = Boolean Array To Number(Boolean array=w876) -> (number=w875:u32)
        n554 = call "Read Stage Position.vi"("error in"=w863, "VISA resource name in"=w864) -> ("Current Position"=w861:cluster{dbl, dbl, dbl}, "error out"=→"Stage error":errorcluster)  [unwired: 1 in, 1 out]
        n555 = Logarithm Base 2(1:w875) -> (0:w869:dbl)
        n556 = Cluster To Array(cluster=w861) -> (array=w871:dbl[])
        n557 = Increment(x=w869) -> (x+1=w872:dbl)
        n558 = Build Array (concatenate)(w872, w871) -> (w870:dbl[])
        n559 = Replace Array Subset(array="Saved stage positions", new element=w870, index (row)=w869) -> (w873:dbl[][])  [unwired: 1 in]
        n560 = local write "Saved stage positions"(w873) -> ()
      }
      event "Move to Position 2", "Move to Position 4", "Move to Position 3", "Move to Position 5", "Move to Position 1": Value Change {
        n561 = event-data() -> ()  [unwired: 1 in, 5 out]
        n562 = Build Array("Move to Position 1", "Move to Position 2", "Move to Position 3", "Move to Position 4", "Move to Position 5") -> (w886:bool[])
        n563 = Boolean Array To Number(Boolean array=w886) -> (number=w885:u32)
        n564 = Logarithm Base 2(1:w885) -> (0:w884:dbl)
        n565 = flat-sequence {
          tunnel: w884 -> [w891]
          tunnel: w883 -> [w890]
          tunnel: w882 -> [w889]
          frame #0 {
            n566 = local read "Saved stage positions"() -> (w892:dbl[][])
            n567 = Increment(x=w891) -> (x+1=w888:dbl)
            n568 = call "move to saved stage position.vi"("error in"=w889, "Stage VISA resource name in"=w890, "Position"=w888, "Saved Stage Positions"=w892) -> ()  [unwired: 2 out]
            "Stage moving" <- TRUE ("Stage moving")
          }
          frame #1 {
            n569 = call <vilib>:"Beep.vi"() -> ()  [unwired: 12 in]
            n570 = local write "Stage moving"(FALSE ("Stage moving")) -> ()
          }
        }
      }
      event "Dip": Value Change {
        n571 = event-data() -> ()  [unwired: 1 in, 5 out]
        n572 = local write "Dip"(FALSE ("Dip")) -> ()
        n573 = flat-sequence {
          tunnel: w903 -> [w905]
          tunnel: w902 -> [w904]
          tunnel: [w906] -> w900
          tunnel: [w905] -> w898
          tunnel: [w904] -> w896
          tunnel: [w914] -> w901
          tunnel: w900 -> [w914]
          tunnel: [w913] -> w899
          tunnel: w898 -> [w913]
          tunnel: [w912] -> w897
          tunnel: w896 -> [w912]
          tunnel: w901 -> [w933]
          tunnel: w899 -> [w932]
          tunnel: w897 -> [w931]
          frame #0 {
            n574 = local read "Saved stage positions"() -> (w906:dbl[][])
            n575 = local write "Stage moving"(TRUE) -> ()
            n576 = call "move to saved stage position.vi"("error in"=w904, "Stage VISA resource name in"=w905, "Position"="Dip position", "Saved Stage Positions"=w906) -> ()  [unwired: 2 out]
          }
          frame #1 {
            n577 = node-c288() -> (w911:T12)  [unwired: 4 in]
            n578 = timed-loop {
              timing: w911 -> [_]
              timing-out: [_] -> w910
              i -> [w924]
              stop <- w915 stop-if-true
              n579 = node-c288() -> ()  [unwired: 1 in, 1 out]
              n580 = Greater Or Equal?(x=w924, y="Dip duration") -> (x >= y?=w920:bool)
              n581 = local read "Dump beads"() -> (w917:bool)
              n582 = Or(x=w920, y="Cancel dwell") -> (x .or. y?=w918:bool)
              n583 = Not(x="Pause dwell") -> (.not. x?=w921:bool)
              n584 = node-c288() -> ()  [unwired: 1 in, 1 out]
              n585 = And(x=w921, y=w918) -> (x .and. y?=w916:bool)
              n586 = Or(x=w916, y=w917) -> (x .or. y?=w915:bool)
              "Dip time" <- w924
            }
            n587 = local write "Stage moving"(FALSE ("Stage moving")) -> ()
            n588 = node-c288(w910) -> ()  [unwired: 1 out]
          }
          frame #2 {
            n589 = local write "Cancel dwell"(FALSE ("Cancel dwell")) -> ()
            n590 = call "move to saved stage position.vi"("error in"=w931, "Stage VISA resource name in"=w932, "Position"="Return position", "Saved Stage Positions"=w933) -> ()  [unwired: 2 out]
          }
          frame #3 {
            n591 = local write "Stage moving"(FALSE ("Stage moving")) -> ()
          }
        }
      }
      event "Force FB script": Value Change {
        n592 = event-data() -> ()  [unwired: 1 in, 5 out]
        n593 = flat-sequence {
          frame #0 {
            n594 = disable-structure shown="Disabled" {
              frame Disabled {
                n595 = local read "# Samples/channel"() -> (w937:i32)
                n596 = local write "# Samples/channel (in)"(w937) -> ()
              }
              frame Enabled {
              }
            }
            n597 = local write "Force FB script"(FALSE ("Force FB script")) -> ()
            n598 = property on="Trap delta" class="DigNum (strict)"("Val(Sgnl)"="Start trap delta (V)") -> ()  [unwired: 2 in, 2 out]
          }
          frame #1 {
            n599 = Wait (ms)(milliseconds to wait=u32 500) -> ()  [unwired: 1 out]
          }
          frame #2 {
            n600 = property on="Set reading to\nsetpoint" class="Bool (strict)"("Val(Sgnl)"=TRUE ("Value (Signaling)")) -> ()  [unwired: 2 in, 2 out]
          }
          frame #3 {
            n601 = Wait (ms)(milliseconds to wait=u32 300) -> ()  [unwired: 1 out]
          }
          frame #4 {
            n602 = local write "Force Feedback"(TRUE ("Force Feedback")) -> ()
            n603 = property on="Tabs" class="TabCtl (strict)"("Val(Sgnl)"=T3."Force Feedback" ("Value (Signaling)")) -> ()  [unwired: 2 in, 2 out]
          }
          frame #5 {
            n604 = property on="Save Data" class="Bool (strict)"("Val(Sgnl)"=TRUE ("Value (Signaling)")) -> ()  [unwired: 2 in, 2 out]
          }
          frame #6 {
            n605 = Multiply(x="Wait before dip (s)", y=1000) -> (x*y=w944:dbl)
            n606 = Wait (ms)(milliseconds to wait=w944) -> ()  [unwired: 1 out]
          }
          frame #7 {
            n607 = case shown="True" "Start dipping after?" {
              selector: "Start dipping after?" -> [_ w949]
              frame False {
              }
              frame True {
                n608 = property on="Dip" class="Bool (strict)"("Val(Sgnl)"=w949) -> ()  [unwired: 2 in, 2 out]
              }
            }
            n609 = property on="Remove offsets" class="Bool (strict)"("Val(Sgnl)"=TRUE ("Value (Signaling)")) -> ()  [unwired: 2 in, 2 out]
          }
        }
      }
      event "Move 0": Value Change {
        n610 = event-data() -> ()  [unwired: 1 in, 5 out]
        n611 = local write "Move 0"(FALSE) -> ()
        n612 = call "HalfWavePlate.vi"("Degrees"="\"Degrees\" 0", "Motor"=0) -> ()  [unwired: 1 in]
      }
      event "Move 1": Value Change {
        n613 = event-data() -> ()  [unwired: 1 in, 5 out]
        n614 = local write "Move 1"(FALSE) -> ()
        n615 = call "HalfWavePlate.vi"("Degrees"="\"Degrees\" 1", "Motor"=1) -> ()  [unwired: 1 in]
      }
      event "Stop": Value Change {
        n616 = event-data() -> ()  [unwired: 1 in, 5 out]
        n617 = local read "Stop"() -> (w956:bool)
      }
    }
    n618 = node-c288() -> ()  [unwired: 1 in, 1 out]
  }
  n619 = call <vilib>:"Simple Error Handler.vi"("error in (no error)"=w105) -> ()  [unwired: 4 in, 5 out]
  n620 = node-c288(2 ("Processor")) -> (w75:T12)  [unwired: 3 in]
  n621 = node-c288(2 ("Processor")) -> (w27:T12)  [unwired: 3 in]
  n622 = timed-loop {
    timing: w75 -> [_]
    timing-out: [_] -> w74
    stop <- w959 stop-if-true
    n623 = node-c288() -> ()  [unwired: 1 in, 1 out]
    n624 = case shown="\"Current Saved Data\"" "Tab Control" {
      frame "Control" {
        n625 = case shown="True" "Start" {
          frame False {
          }
          frame True {
            w972 = T15 3 items=["no dialog", "OK message", "continue or stop message", "OK message + warnings", "continue/stop + warnings"] ("type of dialog (OK msg:1)")
            n626 = call "InitializeAcquireFF.vi"("DAQ Rate"="DAQ Rate", "Averaging Number"="Averaging Number", "Sampling Rate"="Sampling Rate") -> ("error out"=w966:errorcluster, "task out"=w965:refnum<k21>, "Final Sampling Rate"=→"Final Sampling Rate":dbl)  [unwired: 4 in, 2 out]
            n627 = while {
              tunnel: [w984] -> w971
              tunnel: [w983] -> w964
              tunnel: "Averaging Number" -> [w982]
              tunnel: w966 -> [w981]
              tunnel: w965 -> [w979]
              stop <- w980 continue-if-true
              n628 = call "Acquire2_QPD.vi"("task/channels in"=w979, "Save Data?"=FALSE ("Take Data?"), "Averaging Number"=w982, "error in"=w981) -> ("PSD 1"=→"PSD 1":cluster{dbl[], dbl[]}, "PSD 1 Sum"=→"PSD 1 Sum":dbl, "PSD 2"=→"PSD 2":cluster{dbl[], dbl[]}, "PSD 2 Sum"=→"PSD 2 Sum":dbl, "task out"=w984:refnum<k21>, "error out"=w983:errorcluster)  [unwired: 14 in, 4 out]
              n629 = local read "Start"() -> (w980:bool)
            }
            n630 = call <vilib>:"DAQmx Clear Task.vi"("task in"=w971, "error in"=w964) -> ("error out"=w973:errorcluster)  [unwired: 13 in]
            n631 = call <vilib>:"Simple Error Handler.vi"("type of dialog (OK msg:1)"=w972, "error in (no error)"=w973) -> ()  [unwired: 3 in, 5 out]
          }
        }
      }
      frame "Current Saved Data" {
      }
      frame "Data Acquisition" {
      }
      frame "Raw QPD Data" {
      }
    }
    n632 = local read "Stop"() -> (w959:bool)
    n633 = node-c288() -> ()  [unwired: 1 in, 1 out]
  }
  n634 = call-poly <vilib>:"DAQmx Create Virtual Channel.vi"("lines"=w92) -> ("task out"=w91:refnum<k21>)  [unwired: 13 in, 1 out]
  n635 = call-poly <vilib>:"DAQmx Create Virtual Channel.vi"("lines"=w95) -> ("task out"=w94:refnum<k21>)  [unwired: 13 in, 1 out]
  n636 = timed-loop {
    timing: w27 -> [_]
    timing-out: [_] -> w26
    stop <- w985 stop-if-true
    n637 = node-c288() -> ()  [unwired: 1 in, 1 out]
    n638 = event shown="[0] \"Pause Mouse/Mirror Connection\": Value Change" {
      selector: _ -> [_ _]
      dyn-events: _ -> [_ _]
      timeout: _ -> [_ _]
      tunnel: [w1078 _] -> w986
      tunnel: [_ w1079] -> w985
      event "Pause Mouse/Mirror Connection": Value Change {
        n639 = event-data() -> ("NewVal"=w1078:bool)  [unwired: 1 in]
      }
      event "Stop": Value Change {
        n640 = event-data() -> ("NewVal"=w1079:bool)  [unwired: 1 in]
      }
    }
    n641 = case shown="True" w986 {
      frame False {
      }
      frame True {
        n642 = call "InitializeMouseControl.vi"() -> ("error out 2"=w995:errorcluster, "task out"=w996:refnum<k21>, "error out"=w998:errorcluster, "device ID"=w997:refnum<k1>)  [unwired: 8 in]
        n643 = while {
          tunnel: w998 -> [w1010]
          tunnel: w997 -> [w1009]
          tunnel: w996 -> [w1008]
          tunnel: w995 -> [w1007]
          tunnel: [w1006] -> w993
          tunnel: [w1005] -> w992
          tunnel: [w1004] -> w989
          tunnel: [w1003] -> w990
          stop <- w1002 stop-if-true
          n644 = case shown="True" "Use Mouse to Move Trap?" {
            tunnel: w1009 -> [w1017 w1040]
            tunnel: w1010 -> [w1016 w1039]
            tunnel: w1008 -> [w1015 w1038]
            tunnel: w1007 -> [w1014 w1037]
            tunnel: [w1017 w1036] -> w1004
            tunnel: [w1016 w1035] -> w1003
            tunnel: [w1015 w1034] -> w1006
            tunnel: [w1014 w1033] -> w1005
            frame False {
              (unwired) FALSE ("button 1")
            }
            frame True {
              w1028 = 0.0 ("y")
              w1030 = 10
              n645 = local read "Deflection"() -> (w1041:T4)
              n646 = call-poly <vilib>:"Acquire Input Data.vi"("device ID"=w1040, "error in (no error)"=w1039) -> ("device ID"=w1036:refnum<k1>, "button info"=w1054:T16, "error out"=w1035:errorcluster)  [unwired: 14 in, 1 out]
              n647 = Unbundle By Name(w1041) -> ("Horizontal"=w1043:i32, "Vertical"=w1042:i32)
              n648 = local read "Saved voltage"() -> (w1019:cluster{dbl, dbl})
              n649 = Divide(x=w1043, y=30) -> (x/y=w1046:dbl)
              n650 = Divide(x=w1042, y=-20) -> (x/y=w1047:dbl)
              n651 = Unbundle By Name(w1054) -> ("button 1"=w1032:bool, "button 2"=w1048:bool)
              n652 = Bundle(w1046, w1047) -> (w1024:cluster{dbl, dbl})  [unwired: 1 in]
              n653 = local write "Reference Voltage"(w1024) -> ()
              n654 = Add(x=w1024, y=w1019) -> (x+y=w1052:cluster{dbl, dbl})
              n655 = case shown="True" w1032 {
                frame False {
                  n656 = stacked-sequence {
                    frame #0 {
                      n657 = local write "CoordinatesMousePressed"(T4 {"Horizontal"=0, "Vertical"=0} ("Coords when pressed")) -> ()
                      n658 = local write "Deflection"(T4 {"Horizontal"=0, "Vertical"=0} ("deflaction")) -> ()
                    }
                  }
                }
                frame True {
                  n659 = local read "CoordinatesMousePressed"() -> (w1077:T4)
                  n660 = local read "Real Coordinates"() -> (w1076:cluster{"Horizontal":i32, "Vertical":i32})
                  n661 = Subtract(x=w1076, y=w1077) -> (x-y=w1075:T4)
                  n662 = local write "Deflection"(w1075) -> ()
                }
              }
              n663 = Unbundle(w1052) -> (w1029:dbl, w1020:dbl)
              n664 = case shown="True" w1048 {
                frame False {
                }
                frame True {
                  n665 = local read "Reference Voltage"() -> (w1058:cluster{dbl, dbl})
                  n666 = local read "Saved voltage"() -> (w1056:cluster{dbl, dbl})
                  n667 = Add(x=w1058, y=w1056) -> (x+y=→"Saved voltage":cluster{dbl, dbl})
                  n668 = local read "Real Coordinates"() -> (w1057:cluster{"Horizontal":i32, "Vertical":i32})
                  n669 = local write "CoordinatesMousePressed"(w1057) -> ()
                }
              }
              n670 = Less?(x=w1029, y=w1030) -> (x < y?=w1027:bool)
              n671 = Greater?(x=w1029, y=w1028) -> (0:w1026:bool)
              n672 = Greater?(x=w1020, y=w1028) -> (0:w1022:bool)
              n673 = Less?(x=w1020, y=w1030) -> (x < y?=w1023:bool)
              n674 = And(x=w1022, y=w1023) -> (x .and. y?=w1021:bool)
              n675 = And(x=w1027, y=w1026) -> (x .and. y?=w1025:bool)
              n676 = case shown="False" w1021 {
                tunnel: [w1068 w1072] -> w1031
                tunnel: w1020 -> [w1066 w1072]
                frame False {
                  n677 = Greater?(x=w1066, y=10.0) -> (0:w1069:bool)
                  n678 = case shown="True" w1069 {
                    tunnel: [0.0 10.0] -> w1068
                    frame False {
                    }
                    frame True {
                    }
                  }
                }
                frame True {
                }
              }
              n679 = case shown="False" w1025 {
                tunnel: w1029 -> [w1060 w1065]
                tunnel: [w1061 w1065] -> w1053
                frame False {
                  n680 = Greater?(x=w1060, y=10.0) -> (0:w1062:bool)
                  n681 = case shown="True" w1062 {
                    tunnel: [0.0 10.0] -> w1061
                    frame False {
                    }
                    frame True {
                    }
                  }
                }
                frame True {
                }
              }
              n682 = Bundle(w1053, w1031) -> (w1018:cluster{dbl, dbl})  [unwired: 1 in]
              n683 = Cluster To Array(cluster=w1018) -> (array=w1049:dbl[])
              n684 = call-poly <vilib>:"DAQmx Write.vi"("task/channels in"=w1038, "data"=w1049, "error in"=w1037) -> ("task out"=w1051:refnum<k21>, "error out"=w1050:errorcluster)  [unwired: 10 in, 1 out]
              n685 = call <vilib>:"DAQmx Is Task Done.vi"("task/channels in"=w1051, "error in"=w1050) -> ("task out"=w1034:refnum<k21>, "error out"=w1033:errorcluster)  [unwired: 11 in, 1 out]
            }
          }
          n686 = event shown="[0] \"Pane\": Mouse Move" {
            selector: _ -> [_ _ _]
            dyn-events: _ -> [_ _ _]
            timeout: _ -> [_ _ _]
            event Mouse Move {
              n687 = event-data() -> ("Coords"=w1012:T4)  [unwired: 1 in]
              n688 = local write "Real Coordinates"(w1012) -> ()
            }
            event Mouse Down {
              n689 = event-data() -> ("Coords"=w1013:T4)  [unwired: 1 in]
              n690 = local write "CoordinatesMousePressed"(w1013) -> ()
            }
            event "Pause Mouse/Mirror Connection": Value Change {
              n691 = event-data() -> ()  [unwired: 1 in, 3 out]
            }
          }
          n692 = local read "Stop"() -> (w999:bool)
          n693 = Not(x="Pause Mouse/Mirror Connection") -> (.not. x?=w1000:bool)
          n694 = Or(x=w1000, y=w999) -> (x .or. y?=w1002:bool)
        }
        n695 = call <vilib>:"DAQmx Clear Task.vi"("task in"=w993, "error in"=w992) -> ("error out"=w994:errorcluster)  [unwired: 13 in]
        n696 = call <vilib>:"Simple Error Handler.vi"("error in (no error)"=w994) -> ()  [unwired: 4 in, 5 out]
        n697 = call-poly <vilib>:"Close Input Device.vi"("error in (no error)"=w990, "device ID"=w989) -> ("error out"=w991:errorcluster)  [unwired: 8 in]
        n698 = call <vilib>:"Simple Error Handler.vi"("error in (no error)"=w991) -> ()  [unwired: 4 in, 5 out]
      }
    }
    n699 = node-c288() -> ()  [unwired: 1 in, 1 out]
  }
  n700 = node-c288(i64 100 ("Period")) -> (w89:T12)  [unwired: 3 in]
  n701 = timed-loop {
    tunnel: w91 -> [w1082]
    tunnel: [w1081] -> w90
    tunnel: w94 -> [w1084]
    tunnel: [w1083] -> w93
    timing: w89 -> [_]
    timing-out: [_] -> w88
    stop <- w1080 stop-if-true
    n702 = node-c288() -> ()  [unwired: 1 in, 1 out]
    n703 = event shown="[1] \"Shutter 2 (A)\": Value Change" {
      selector: _ -> [_ _ _]
      dyn-events: _ -> [_ _ _]
      timeout: _ -> [_ _ _]
      tunnel: w1084 -> [w1088 _ _]
      tunnel: [w1087 _ _] -> w1083
      tunnel: w1082 -> [_ w1108 _]
      tunnel: [_ w1106 _] -> w1081
      tunnel: [_ _ w1125] -> w1080
      event "Shutter 1 (B)": Value Change {
        n704 = event-data() -> ()  [unwired: 1 in, 1 out]
        n705 = flat-sequence {
          tunnel: [w1094] -> w1091
          tunnel: w1088 -> [w1093]
          tunnel: [w1098] -> w1090
          tunnel: [w1101] -> w1089
          tunnel: w1091 -> [w1096]
          tunnel: w1090 -> [w1105]
          tunnel: w1089 -> [w1103]
          tunnel: [w1102] -> w1087
          frame #0 {
            n706 = call-poly <vilib>:"DAQmx Write.vi"("task/channels in"=w1093, "data"=FALSE) -> ("task out"=w1094:refnum<k21>)  [unwired: 11 in, 2 out]
            n707 = Wait (ms)(milliseconds to wait=100) -> ()  [unwired: 1 out]
          }
          frame #1 {
            n708 = Or(x="Shutter 1 (B)", y=TRUE) -> (x .or. y?=w1098:bool)
            n709 = call-poly <vilib>:"DAQmx Write.vi"("task/channels in"=w1096, "data"=w1098) -> ("task out"=w1101:refnum<k21>)  [unwired: 11 in, 2 out]
            n710 = Wait (ms)(milliseconds to wait=100) -> ()  [unwired: 1 out]
          }
          frame #2 {
            n711 = Not(x=w1105) -> (.not. x?=w1104:bool)
            n712 = call-poly <vilib>:"DAQmx Write.vi"("task/channels in"=w1103, "data"=w1104) -> ("task out"=w1102:refnum<k21>)  [unwired: 11 in, 2 out]
          }
        }
      }
      event "Shutter 2 (A)": Value Change {
        n713 = event-data() -> ()  [unwired: 1 in, 1 out]
        n714 = flat-sequence {
          tunnel: w1108 -> [w1113]
          tunnel: [w1112] -> w1107
          tunnel: [w1117] -> w1110
          tunnel: [w1120] -> w1109
          tunnel: w1107 -> [w1115]
          tunnel: w1110 -> [w1124]
          tunnel: w1109 -> [w1122]
          tunnel: [w1121] -> w1106
          frame #0 {
            n715 = call-poly <vilib>:"DAQmx Write.vi"("task/channels in"=w1113, "data"=FALSE) -> ("task out"=w1112:refnum<k21>)  [unwired: 11 in, 2 out]
            n716 = Wait (ms)(milliseconds to wait=100) -> ()  [unwired: 1 out]
          }
          frame #1 {
            n717 = Or(x="Shutter 2 (A)", y=TRUE) -> (x .or. y?=w1117:bool)
            n718 = call-poly <vilib>:"DAQmx Write.vi"("task/channels in"=w1115, "data"=w1117) -> ("task out"=w1120:refnum<k21>)  [unwired: 11 in, 2 out]
            n719 = Wait (ms)(milliseconds to wait=100) -> ()  [unwired: 1 out]
          }
          frame #2 {
            n720 = Not(x=w1124) -> (.not. x?=w1123:bool)
            n721 = call-poly <vilib>:"DAQmx Write.vi"("task/channels in"=w1122, "data"=w1123) -> ("task out"=w1121:refnum<k21>)  [unwired: 11 in, 2 out]
          }
        }
      }
      event "Stop": Value Change {
        n722 = event-data() -> ("NewVal"=w1125:bool)  [unwired: 1 in, 5 out]
      }
    }
    n723 = node-c288() -> ()  [unwired: 1 in, 1 out]
  }
  n724 = node-c288(w88) -> ()  [unwired: 1 out]
  n725 = node-c288(w74) -> ()  [unwired: 1 out]
  n726 = call <vilib>:"DAQmx Clear Task.vi"("task in"=w90) -> ()  [unwired: 14 in, 1 out]
  n727 = call <vilib>:"DAQmx Clear Task.vi"("task in"=w93) -> ()  [unwired: 14 in, 1 out]
  n728 = node-c288(w26) -> ()  [unwired: 1 out]
  n729 = node-c288(w22) -> ()  [unwired: 1 out]
  n730 = local write "Tether"(FALSE ("Tether")) -> ()
  n731 = local read "Path"() -> (w81:path)
  n732 = node-c288(i64 1 ("Period"), 2 ("Processor")) -> (w87:T12)  [unwired: 2 in]
  n733 = VISA Close(VISA resource name=w19) -> (error out=w104:errorcluster)  [unwired: 1 in]
  n734 = timed-loop {
    timing: w87 -> [_]
    timing-out: [_] -> w86
    tunnel: w81 -> [w1127]
    stop <- w1126 stop-if-true
    n735 = node-c288() -> ()  [unwired: 1 in, 1 out]
    n736 = event shown="[5] \"Raster scan\": Value Change" {
      selector: _ -> [_ _ _ _ _ _ _ _ _ _]
      dyn-events: _ -> [_ _ _ _ _ _ _ _ _ _]
      timeout: _ -> [_ _ _ _ _ _ _ _ _ _]
      tunnel: w1127 -> [_ w1131 _ _ _ _ _ _ _ _]
      tunnel: [_ _ w1151 _ _ _ _ _ _ _] -> w1126
      event Timeout {
        n737 = event-data() -> ()  [unwired: 1 in, 2 out]
      }
      event "Read Cal": Value Change {
        n738 = event-data() -> ()  [unwired: 1 in, 6 out]
        n739 = Path To String(path=w1131) -> (string=w1130:string)
        n740 = Format Date/Time String(time format string (%c)="%y%m%d") -> (date/time string=w1132:string)  [unwired: 2 in]
        n741 = Concatenate Strings(w1130, "\\" ("string"), w1132, "\\" ("string"), "current.cal") -> (w1150:string)
        n742 = String To Path(string=w1150) -> (path=w1149:path)
        n743 = Open/Create/Replace File(file path (use dialog)=w1149, operation (0:open)=T9."open", access (0:read/write)=enum16{"read/write", "read-only", "write-only"}."read-only") -> (refnum out=w1145:refnum<file>, error out=w1146:errorcluster)  [unwired: 3 in, 1 out]
        n744 = Deny Access(4:w1146, 7:w1145) -> (0:w1144:errorcluster, 3:w1143:refnum<file>)  [unwired: 1 in]
        n745 = Read from Binary File(5:0.0, 8:w1144, 9:T10."big-endian, network order" ("byte order (0:big-endian, network order)"), 10:12 ("count"), 11:w1143) -> (0:w1139:errorcluster, 2:w1137:dbl[], 3:w1140:refnum<file>)  [unwired: 1 in, 1 out]
        n746 = Array To Cluster(array=w1137) -> (cluster=→"Cal values":T17)
        n747 = Close File(refnum=w1140, error in=w1139) -> ()  [unwired: 2 out]
        n748 = local write "Read Cal"(FALSE ("Read Cal")) -> ()
      }
      event "Stop": Value Change {
        n749 = event-data() -> ("NewVal"=w1151:bool)  [unwired: 1 in, 5 out]
      }
      event "Trap position": Value Change {
        # "Need to rotate so X and Y don't get mixed up."
        n750 = event-data() -> ()  [unwired: 1 in, 6 out]
        n751 = local read "Mirror task"() -> (w1152:refnum<k21>)
        n752 = Cluster To Array(cluster="Trap position") -> (array=w1155:dbl[])
        n753 = Rotate 1D Array(1:w1155, 2:1 ("n")) -> (0:w1153:dbl[])
        n754 = call-poly <vilib>:"DAQmx Write.vi"("task/channels in"=w1152, "data"=w1153) -> ("task out"=w1158:refnum<k21>, "error out"=w1157:errorcluster)  [unwired: 11 in, 1 out]
        n755 = call <vilib>:"DAQmx Stop Task.vi"("task/channels in"=w1158, "error in"=w1157) -> ("error out"=w1156:errorcluster)  [unwired: 12 in, 1 out]
        n756 = call <vilib>:"Simple Error Handler.vi"("error in (no error)"=w1156) -> ()  [unwired: 4 in, 5 out]
      }
      event "Trap delta": Value Change {
        n757 = event-data() -> ()  [unwired: 1 in, 6 out]
        n758 = local read "Pulling direction"() -> (w1161:bool)
        n759 = local read "Fixed Y"() -> (w1165:dbl)
        n760 = local read "Fixed X"() -> (w1164:dbl)
        n761 = Select(t=w1165, s=w1161, f=w1164) -> (s? t:f=w1163:dbl)
        n762 = Add(x="Trap delta", y=w1163) -> (x+y=w1160:dbl)
        n763 = case shown="True" w1161 {
          tunnel: w1160 -> [w1166 w1167]
          frame False {
            n764 = property on="X" class="DigNum (strict)"("Val(Sgnl)"=w1166) -> ()  [unwired: 2 in, 2 out]
          }
          frame True {
            n765 = property on="Y" class="DigNum (strict)"("Val(Sgnl)"=w1167) -> ()  [unwired: 2 in, 2 out]
          }
        }
      }
      event "Raster scan": Value Change {
        w1187 = T15 1 items=["no dialog", "OK message", "continue or stop message", "OK message + warnings", "continue/stop + warnings"] ("type of dialog (OK msg:1)")
        w1179 = 0.0 ("minimum value")
        w1178 = 10.0 ("maximum value")
        # "Grab offset in pulling\ndirection and add to \ndelta values"
        # "Send offset in direction\nof not-pulling to DAQ"
        n766 = event-data() -> ()  [unwired: 1 in, 6 out]
        n767 = call-poly <vilib>:"DAQmx Create Virtual Channel.vi"("maximum value"=w1178, "minimum value"=w1179, "physical channels"=tag "Dev1/ao0") -> ("task out"=w1192:refnum<k21>, "error out"=w1191:errorcluster)  [unwired: 11 in]
        n768 = local read "Fixed Y"() -> (w1181:dbl)
        n769 = local read "Fixed X"() -> (w1182:dbl)
        n770 = Select(t=w1182, s="Pulling direction", f=w1181) -> (s? t:f=w1172:dbl)
        n771 = Select(t=w1181, s="Pulling direction", f=w1182) -> (s? t:f=w1169:dbl)
        n772 = call-poly <vilib>:"DAQmx Create Virtual Channel.vi"("task in"=w1192, "maximum value"=w1178, "minimum value"=w1179, "physical channels"=tag "Dev1/ao1", "error in"=w1191) -> ("task out"=w1186:refnum<k21>, "error out"=w1185:errorcluster)  [unwired: 9 in]
        n773 = local read "Trap delta"() -> (w1171:dbl)
        n774 = Add(x=w1169, y=w1171) -> (x+y=w1170:dbl)
        n775 = while {
          tunnel: "Pulling direction" -> [w1217]
          tunnel: w1170 -> [w1216]
          tunnel: w1172 -> [w1207]
          tunnel: w1186 -> [w1215]
          tunnel: w1185 -> [w1214]
          tunnel: [w1211] -> w1190
          tunnel: [w1210] -> w1189
          tunnel: [w1206] -> w1168
          tunnel: "Trap delta\nafter" -> [w1203]
          tunnel: [w1203] -> w1183
          i -> [w1209]
          stop <- w1206 stop-if-true
          n776 = flat-sequence {
            tunnel: [w1224] -> w1213
            tunnel: [w1223] -> w1212
            tunnel: w1217 -> [w1222]
            tunnel: w1216 -> [w1228]
            tunnel: w1207 -> [w1227]
            tunnel: w1215 -> [w1226]
            tunnel: w1214 -> [w1225]
            tunnel: [w1218] -> w1200
            tunnel: w1213 -> [w1264]
            tunnel: w1212 -> [w1263]
            tunnel: [w1262] -> w1211
            tunnel: [w1261] -> w1210
            tunnel: w1207 -> [w1259]
            tunnel: w1200 -> [w1255]
            frame #0 {
              n777 = local read "Time per step (ms)"() -> (w1219:dbl)
              n778 = node-c288(w1219) -> (w1221:T12)  [unwired: 3 in]
              n779 = timed-loop {
                tunnel: w1228 -> [w1247]
                tunnel: w1227 -> [w1234]
                tunnel: w1226 -> [w1246]
                tunnel: w1225 -> [w1245]
                tunnel: [w1240] -> w1224
                tunnel: [w1241] -> w1223
                tunnel: w1222 -> [w1243]
                timing: w1221 -> [_]
                timing-out: [_] -> w1220
                tunnel: [w1229] -> w1218
                i -> [w1238]
                stop <- w1242 stop-if-true
                n780 = node-c288() -> ()  [unwired: 1 in, 1 out]
                n781 = local read "Scan increment (V)"() -> (w1231:dbl)
                n782 = local read "Scan steps (mirror)"() -> (w1230:u64)
                n783 = Multiply(x=w1231, y=w1238) -> (x*y=w1248:dbl)
                n784 = Add(x=w1247, y=w1248) -> (x+y=w1229:dbl)
                n785 = local read "Stop saving"() -> (w1232:bool)
                n786 = local read "Stop raster"() -> (w1233:bool)
                n787 = Build Array(w1234, w1229) -> (w1235:dbl[])
                n788 = Build Array(w1229, w1234) -> (w1237:dbl[])
                n789 = Greater Or Equal?(x=w1238, y=w1230) -> (x >= y?=w1239:bool)
                n790 = Select(t=w1235, s=w1243, f=w1237) -> (s? t:f=w1236:dbl[])
                n791 = Compound Arithmetic op=OR(w1239, w1233, w1232) -> (w1242:bool)
                n792 = call-poly <vilib>:"DAQmx Write.vi"("task/channels in"=w1246, "auto start"=TRUE, "data"=w1236, "error in"=w1245) -> ("task out"=w1240:refnum<k21>, "error out"=w1241:errorcluster)  [unwired: 9 in, 1 out]
                n793 = node-c288() -> ()  [unwired: 1 in, 1 out]
                "Numeric" <- w1238
              }
              n794 = node-c288(w1220) -> ()  [unwired: 1 out]
            }
            frame #1 {
              n795 = local read "Time per step (ms)"() -> (w1256:dbl)
              n796 = local read "Pulling direction"() -> (w1260:bool)
              n797 = node-c288(w1256) -> (w1258:T12)  [unwired: 3 in]
              n798 = timed-loop {
                tunnel: w1259 -> [w1269]
                tunnel: w1264 -> [w1284]
                tunnel: w1263 -> [w1277]
                tunnel: [w1271] -> w1262
                tunnel: [w1278] -> w1261
                tunnel: w1260 -> [w1280]
                timing: w1258 -> [_]
                timing-out: [_] -> w1257
                tunnel: w1255 -> [w1265]
                i -> [w1275]
                stop <- w1276 stop-if-true
                n799 = node-c288() -> ()  [unwired: 1 in, 1 out]
                n800 = local read "Scan increment (V)"() -> (w1266:dbl)
                n801 = Multiply(x=w1266, y=w1275) -> (x*y=w1274:dbl)
                n802 = Subtract(x=w1265, y=w1274) -> (x-y=w1273:dbl)
                n803 = Build Array(w1269, w1273) -> (w1279:dbl[])
                n804 = Build Array(w1273, w1269) -> (w1272:dbl[])
                n805 = local read "Scan steps (mirror)"() -> (w1267:u64)
                n806 = Select(t=w1279, s=w1280, f=w1272) -> (s? t:f=w1270:dbl[])
                n807 = local read "Stop raster"() -> (w1282:bool)
                n808 = local read "Stop saving"() -> (w1268:bool)
                n809 = call-poly <vilib>:"DAQmx Write.vi"("task/channels in"=w1284, "auto start"=TRUE, "data"=w1270, "error in"=w1277) -> ("task out"=w1271:refnum<k21>, "error out"=w1278:errorcluster)  [unwired: 9 in, 1 out]
                n810 = Greater Or Equal?(x=w1275, y=w1267) -> (x >= y?=w1283:bool)
                n811 = node-c288() -> ()  [unwired: 1 in, 1 out]
                n812 = Compound Arithmetic op=OR(w1283, w1282, w1268) -> (w1276:bool)
                "Numeric 2" <- w1275
              }
              n813 = node-c288(w1257) -> ()  [unwired: 1 out]
            }
          }
          n814 = local read "# scans"() -> (w1202:i32)
          n815 = local read "Stop saving"() -> (w1201:bool)
          n816 = Decrement(x=w1202) -> (x-1=w1204:i32)
          n817 = Greater Or Equal?(x=w1209, y=w1204) -> (x >= y?=w1208:bool)
          n818 = Compound Arithmetic op=OR(w1208, "Stop raster", w1201) -> (w1206:bool)
        }
        n819 = case shown="True" w1168 {
          tunnel: w1183 -> [_ w1195]
          frame False {
          }
          frame True {
            n820 = flat-sequence {
              tunnel: w1195 -> [w1198]
              tunnel: [w1198] -> w1196
              tunnel: w1196 -> [w1199]
              frame #0 {
                n821 = Wait (ms)(milliseconds to wait=u32 300) -> ()  [unwired: 1 out]
              }
              frame #1 {
                n822 = property on="Trap delta" class="DigNum (strict)"("Val(Sgnl)"=w1199) -> ()  [unwired: 2 in, 2 out]
              }
            }
          }
        }
        n823 = call <vilib>:"DAQmx Clear Task.vi"("task in"=w1190, "error in"=w1189) -> ("error out"=w1188:errorcluster)  [unwired: 13 in]
        n824 = Not(x=w1168) -> (.not. x?=w1184:bool)
        n825 = Not(x=w1168) -> (.not. x?=w1180:bool)
        n826 = call <vilib>:"Simple Error Handler.vi"("type of dialog (OK msg:1)"=w1187, "error in (no error)"=w1188) -> ()  [unwired: 3 in, 5 out]
        n827 = local write "Stop raster"(w1184) -> ()
        n828 = local write "Raster scanning..."(w1180) -> ()
        n829 = And(x=w1168, y="Flow on\nafter raster?") -> (x .and. y?=w1173:bool)
        n830 = case shown="True" w1173 {
          frame False {
          }
          frame True {
            n831 = property on="Inject Sample" class="Bool (strict)"("Val(Sgnl)"=TRUE ("Value (Signaling)")) -> ()  [unwired: 2 in, 2 out]
          }
        }
        "Raster scanning..." <- TRUE ("Raster scanning...")
      }
      event "Fish": Value Change {
        n832 = event-data() -> ()  [unwired: 1 in, 6 out]
        n833 = local read "Fish"() -> (w1292:bool)
        n834 = case shown="True" w1292 {
          frame False {
          }
          frame True {
            w1301 = 0.0 ("minimum value")
            w1302 = 10.0 ("maximum value")
            # "Grab offset in pulling\ndirection and add to \ndelta values"
            n835 = call-poly <vilib>:"DAQmx Create Virtual Channel.vi"("maximum value"=w1302, "minimum value"=w1301, "physical channels"=tag "Dev1/ao0") -> ("task out"=w1306:refnum<k21>, "error out"=w1305:errorcluster)  [unwired: 11 in]
            n836 = call-poly <vilib>:"DAQmx Create Virtual Channel.vi"("task in"=w1306, "maximum value"=w1302, "minimum value"=w1301, "physical channels"=tag "Dev1/ao1", "error in"=w1305) -> ("task out"=w1300:refnum<k21>, "error out"=w1299:errorcluster)  [unwired: 9 in]
            n837 = node-c288(i64 1 ("Period")) -> (w1308:T12)  [unwired: 3 in]
            n838 = timed-loop {
              timing: w1308 -> [_]
              timing-out: [_] -> w1307
              tunnel: w1300 -> [w1359]
              tunnel: w1299 -> [w1358]
              tunnel: [w1357] -> w1295
              tunnel: [w1356] -> w1294
              tunnel: [w1324] -> w1297
              tunnel: [w1338] -> w1293
              i -> [w1342]
              stop <- w1338 stop-if-true
              # "Send offset in direction\nof not-pulling to DAQ"
              n839 = node-c288() -> ()  [unwired: 1 in, 1 out]
              n840 = local read "Pulling direction"() -> (w1326:bool)
              n841 = local read "Fixed Y"() -> (w1328:dbl)
              n842 = local read "Fixed X"() -> (w1329:dbl)
              n843 = Select(t=w1328, s=w1326, f=w1329) -> (s? t:f=w1330:dbl)
              n844 = Add(x=w1330, y="Max fish\ndelta (V)") -> (x+y=w1332:dbl)
              n845 = Subtract(x="Max fish\ndelta (V)", y="Min fish\ndelta (V)") -> (x-y=w1334:dbl)
              n846 = Select(t=w1329, s=w1326, f=w1328) -> (s? t:f=w1327:dbl)
              n847 = Divide(x=w1334, y="Fish Speed (ms)") -> (x/y=w1335:dbl)
              n848 = flat-sequence {
                tunnel: w1326 -> [w1378]
                tunnel: w1327 -> [w1377]
                tunnel: w1359 -> [w1376]
                tunnel: w1358 -> [w1375]
                tunnel: w1335 -> [w1374]
                tunnel: w1332 -> [w1373]
                tunnel: "Fish Speed (ms)" -> [w1368]
                tunnel: [w1372] -> w1355
                tunnel: [w1371] -> w1354
                tunnel: [w1370] -> w1353
                tunnel: [w1369] -> w1352
                tunnel: [w1362] -> w1341
                tunnel: [w1361] -> w1325
                tunnel: [w1360] -> w1322
                tunnel: [w1425] -> w1351
                tunnel: w1355 -> [w1425]
                tunnel: [w1424] -> w1350
                tunnel: w1354 -> [w1424]
                tunnel: [w1423] -> w1349
                tunnel: w1353 -> [w1423]
                tunnel: [w1422] -> w1348
                tunnel: w1352 -> [w1422]
                tunnel: w1341 -> [w1421]
                tunnel: [w1421] -> w1340
                tunnel: w1325 -> [w1420]
                tunnel: [w1419] -> w1323
                tunnel: w1322 -> [w1419]
                tunnel: w1351 -> [w1436]
                tunnel: w1350 -> [w1435]
                tunnel: w1349 -> [w1434]
                tunnel: w1348 -> [w1433]
                tunnel: w1337 -> [w1432]
                tunnel: [w1431] -> w1357
                tunnel: [w1430] -> w1356
                tunnel: w1340 -> [w1429]
                tunnel: [w1428] -> w1324
                tunnel: w1323 -> [w1427]
                frame #0 {
                  n849 = local read "Mean force (pN)"() -> (w1367:dbl)
                  n850 = local read "Cutoff force (pN)"() -> (w1366:dbl)
                  n851 = Less Or Equal?(x=w1367, y=w1366) -> (x <= y?=w1364:bool)
                  n852 = And(x="Fish", y=w1364) -> (x .and. y?=w1365:bool)
                  n853 = case shown="True" w1365 {
                    selector: w1365 -> [w1380 _]
                    tunnel: w1378 -> [w1383 w1399]
                    tunnel: w1377 -> [_ w1398]
                    tunnel: w1376 -> [w1385 w1397]
                    tunnel: w1375 -> [w1384 w1396]
                    tunnel: w1374 -> [w1382 w1395]
                    tunnel: w1373 -> [w1381 w1394]
                    tunnel: [w1385 w1393] -> w1372
                    tunnel: [w1384 w1392] -> w1371
                    tunnel: [w1383 w1391] -> w1370
                    tunnel: [w1381 w1390] -> w1360
                    tunnel: [w1382 w1389] -> w1369
                    tunnel: w1368 -> [_ w1388]
                    tunnel: [w1380 w1387] -> w1362
                    tunnel: [FALSE w1386] -> w1361
                    frame False {
                    }
                    frame True {
                      n854 = while {
                        tunnel: w1399 -> [w1408]
                        tunnel: w1398 -> [w1407]
                        tunnel: w1397 -> [w1415]
                        tunnel: w1396 -> [w1414]
                        tunnel: w1395 -> [w1406]
                        tunnel: w1394 -> [w1412]
                        tunnel: [w1410] -> w1393
                        tunnel: [w1409] -> w1392
                        tunnel: [w1408] -> w1391
                        tunnel: [w1407] -> w1390
                        tunnel: [w1406] -> w1389
                        tunnel: w1388 -> [w1405]
                        tunnel: [w1400] -> w1387
                        tunnel: [w1400] -> w1386
                        i -> [w1404]
                        stop <- w1401 stop-if-true
                        n855 = Multiply(x=w1406, y=w1404) -> (x*y=w1413:dbl)
                        n856 = Subtract(x=w1412, y=w1413) -> (x-y=w1411:dbl)
                        n857 = Build Array(w1407, w1411) -> (w1418:dbl[])
                        n858 = Build Array(w1411, w1407) -> (w1417:dbl[])
                        n859 = Greater Or Equal?(x=w1404, y=w1405) -> (x >= y?=w1400:bool)
                        n860 = Select(t=w1418, s=w1408, f=w1417) -> (s? t:f=w1416:dbl[])
                        n861 = local read "Fish"() -> (w1402:bool)
                        n862 = Not(x=w1402) -> (.not. x?=w1403:bool)
                        n863 = call-poly <vilib>:"DAQmx Write.vi"("task/channels in"=w1415, "data"=w1416, "error in"=w1414) -> ("task out"=w1410:refnum<k21>, "error out"=w1409:errorcluster)  [unwired: 10 in, 1 out]
                        n864 = Compound Arithmetic op=OR(w1400, w1403) -> (w1401:bool)
                      }
                    }
                  }
                }
                frame #1 {
                  n865 = case shown="True" w1420 {
                    frame False {
                    }
                    frame True {
                      n866 = Wait (ms)(milliseconds to wait="Wait (ms)") -> ()  [unwired: 1 out]
                    }
                  }
                }
                frame #2 {
                  n867 = case shown="True" w1429 {
                    tunnel: w1436 -> [w1439 w1448]
                    tunnel: w1435 -> [w1438 w1447]
                    tunnel: w1434 -> [_ w1446]
                    tunnel: w1433 -> [_ w1445]
                    tunnel: w1432 -> [_ w1444]
                    tunnel: [w1439 w1443] -> w1431
                    tunnel: [w1438 w1442] -> w1430
                    tunnel: [FALSE w1441] -> w1428
                    tunnel: w1427 -> [_ w1440]
                    frame False {
                    }
                    frame True {
                      n868 = while {
                        tunnel: w1448 -> [w1476]
                        tunnel: w1447 -> [w1475]
                        tunnel: w1446 -> [w1458]
                        tunnel: w1445 -> [w1473]
                        tunnel: w1444 -> [w1472]
                        tunnel: [w1468] -> w1443
                        tunnel: [w1467] -> w1442
                        tunnel: [w1450] -> w1441
                        tunnel: w1440 -> [w1452]
                        i -> [w1459]
                        stop <- w1464 stop-if-true
                        # "If tether formed,\nimmediately change\nto new delta."
                        n869 = local read "Fixed Y"() -> (w1451:dbl)
                        n870 = local read "Fixed X"() -> (w1457:dbl)
                        n871 = local read "Cutoff force (pN)"() -> (w1460:dbl)
                        n872 = Multiply(x=w1473, y=w1459) -> (x*y=w1474:dbl)
                        n873 = local read "Mean force (pN)"() -> (w1461:dbl)
                        n874 = Add(x=w1472, y=w1474) -> (x+y=w1454:dbl)
                        n875 = Select(t=w1451, s=w1458, f=w1457) -> (s? t:f=w1456:dbl)
                        n876 = Greater?(x=w1461, y=w1460) -> (0:w1450:bool)
                        n877 = Add(x=w1456, y="Delta after tether") -> (x+y=w1455:dbl)
                        n878 = Select(t=w1455, s=w1450, f=w1454) -> (s? t:f=w1453:dbl)
                        n879 = local read "Fish Speed (ms)"() -> (w1466:i32)
                        n880 = case shown="True" w1450 {
                          tunnel: "Delta after tether" -> [_ w1477]
                          frame False {
                          }
                          frame True {
                            n881 = property on="Trap delta" class="DigNum (strict)"("Val(Sgnl)"=w1477) -> ()  [unwired: 2 in, 2 out]
                          }
                        }
                        n882 = Build Array(w1452, w1453) -> (w1471:dbl[])
                        n883 = Build Array(w1453, w1452) -> (w1470:dbl[])
                        n884 = Select(t=w1471, s=w1458, f=w1470) -> (s? t:f=w1469:dbl[])
                        n885 = local read "Fish"() -> (w1463:bool)
                        n886 = Greater Or Equal?(x=w1459, y=w1466) -> (x >= y?=w1465:bool)
                        n887 = Not(x=w1463) -> (.not. x?=w1462:bool)
                        n888 = call-poly <vilib>:"DAQmx Write.vi"("task/channels in"=w1476, "data"=w1469, "error in"=w1475) -> ("task out"=w1468:refnum<k21>, "error out"=w1467:errorcluster)  [unwired: 10 in, 1 out]
                        n889 = Compound Arithmetic op=OR(w1465, w1462, w1450) -> (w1464:bool)
                      }
                    }
                  }
                }
              }
              n890 = Add(x=w1330, y="Min fish\ndelta (V)") -> (x+y=w1337:dbl)
              n891 = Decrement(x="# attempts") -> (x-1=w1346:dbl)
              n892 = Greater Or Equal?(x=w1342, y=w1346) -> (x >= y?=w1345:bool)
              n893 = local read "Mean force (pN)"() -> (w1344:dbl)
              n894 = Greater?(x=w1344, y="Cutoff force (pN)") -> (0:w1339:bool)
              n895 = Compound Arithmetic op=OR(w1324, w1339, w1345) -> (w1338:bool)
              n896 = case shown="True" w1324 {
                frame False {
                }
                frame True {
                  n897 = call <vilib>:"Beep.vi"() -> ()  [unwired: 12 in]
                }
              }
              n898 = node-c288() -> ()  [unwired: 1 in, 1 out]
              "Tether" <- w1324
              "Attempt #" <- w1342
            }
            n899 = node-c288(w1307) -> ()  [unwired: 1 out]
            n900 = flat-sequence {
              tunnel: w1297 -> [w1316]
              tunnel: [w1316] -> w1296
              tunnel: w1295 -> [w1313]
              tunnel: w1294 -> [w1312]
              tunnel: w1293 -> [w1311]
              tunnel: w1296 -> [w1318]
              frame #0 {
                w1315 = T15 1 items=["no dialog", "OK message", "continue or stop message", "OK message + warnings", "continue/stop + warnings"] ("type of dialog (OK msg:1)")
                n901 = call <vilib>:"DAQmx Clear Task.vi"("task in"=w1313, "error in"=w1312) -> ("error out"=w1314:errorcluster)  [unwired: 13 in]
                n902 = Not(x=w1311) -> (.not. x?=w1310:bool)
                n903 = local write "Fish"(w1310) -> ()
                n904 = Wait (ms)(milliseconds to wait=u32 300) -> ()  [unwired: 1 out]
                n905 = call <vilib>:"Simple Error Handler.vi"("type of dialog (OK msg:1)"=w1315, "error in (no error)"=w1314) -> ()  [unwired: 3 in, 5 out]
              }
              frame #1 {
                n906 = And(x=w1318, y="Raster after\n tether?") -> (x .and. y?=w1319:bool)
                n907 = case shown="True" w1319 {
                  selector: w1319 -> [_ w1321]
                  frame False {
                  }
                  frame True {
                    n908 = property on="Raster scan" class="Bool (strict)"("Val(Sgnl)"=w1321) -> ()  [unwired: 2 in, 2 out]
                    n909 = property on="Inject Sample" class="Bool (strict)"("Val(Sgnl)"=FALSE ("Value (Signaling)")) -> ()  [unwired: 2 in, 2 out]
                  }
                }
              }
            }
          }
        }
      }
      event "Load param": Value Change {
        n910 = event-data() -> ()  [unwired: 1 in, 6 out]
        n911 = property on="Scan Parameters" class="Arr (strict)"() -> ("Index Values"=w1490:u32[])  [unwired: 2 in, 2 out]
        n912 = Index Array(array=w1490, index=0) -> (element=w1487:u32)
        n913 = Index Array(array="Scan Parameters", index=w1487) -> (element=w1486:T18)
        n914 = Unbundle(w1486) -> ("# scans 2"=w1485:i32)  [unwired: 4 out]
        n915 = local write "Load param"(FALSE ("Load param")) -> ()
        n916 = property on="# scans" class="DigNum (strict)"("Val(Sgnl)"=w1485) -> ()  [unwired: 2 in, 2 out]
      }
      event "Step size (nm)", "Scan speed (nm/s)", "# scans", "Pulling direction": Value Change {
        n917 = event-data() -> ()  [unwired: 1 in, 6 out]
        n918 = local read "Pulling direction"() -> (w1517:bool)
        n919 = Reciprocal(x="Scan speed (nm/s)") -> (1/x=w1509:dbl)
        n920 = local read "Conv Y (nm/V)"() -> (w1515:dbl)
        n921 = local read "Conv X (nm/V)"() -> (w1516:dbl)
        n922 = Multiply(x="Step size (nm)", y=w1509) -> (x*y=w1507:dbl)
        n923 = Divide(x="Scan range (nm)", y="Step size (nm)") -> (x/y=w1514:dbl)
        n924 = Absolute Value(x=w1514) -> (abs(x)=w1513:dbl)
        n925 = Multiply(x=w1507, y=1000.0) -> (x*y=w1494:dbl)
        n926 = Select(t=w1515, s=w1517, f=w1516) -> (s? t:f=w1505:dbl)
        n927 = Multiply(x="# scans", y=2) -> (x*y=w1492:i32)
        n928 = To Unsigned Quad Integer(1:w1513) -> (0:w1503:u64)
        "Scan steps (mirror)" <- w1503
        n929 = Divide(x="Scan range (nm)", y=w1505) -> (x/y=→"Scan range (V)":dbl)
        n930 = Multiply(x=w1503, y=w1494) -> (x*y=w1502:dbl)
        n931 = Divide(x="Step size (nm)", y=w1505) -> (x/y=→"Scan increment (V)":dbl)
        n932 = Round Toward +Infinity(x=w1494) -> (ceil(x): smallest int >= x=→"Time per step (ms)":dbl)
        n933 = local read "Data update period (s/set)"() -> (w1497:dbl)
        n934 = Multiply(x=w1492, y=w1502) -> (x*y=w1500:dbl)
        n935 = Divide(x=w1500, y=1000.0) -> (x/y=w1498:dbl)
        "Total raster time (s)" <- w1498
        n936 = Divide(x=w1498, y=w1497) -> (x/y=w1496:dbl)
        n937 = Round Toward -Infinity(1:w1496) -> (0:→"N sets to be saved":dbl)
      }
      event "Averaging Number": Value Change {
        n938 = event-data() -> ()  [unwired: 1 in, 6 out]
        n939 = local read "# Samples/channel (in)"() -> (w1521:i32)
        n940 = local read "Averaging Number"() -> (w1519:i32)
        n941 = Quotient & Remainder(x=w1521, y=w1519) -> (floor(x/y)=w1520:i32)  [unwired: 1 out]
        n942 = Multiply(x=w1520, y=w1519) -> (x*y=w1518:i32)
        n943 = local write "# Samples/channel (in)"(w1518) -> ()
      }
    }
    n944 = node-c288() -> ()  [unwired: 1 in, 1 out]
  }
  n945 = call <vilib>:"Simple Error Handler.vi"("error in (no error)"=w104) -> ()  [unwired: 4 in, 5 out]
  n946 = disable-structure shown="Enabled" {
    frame Disabled {
      n947 = node-c288(2 ("Processor")) -> (w1527:T12)  [unwired: 3 in]
      n948 = timed-loop "Pump Control" {
        timing: w1527 -> [_]
        timing-out: [_] -> w1526
        tunnel: refnum<visa-resource-name> "COM6" ("VISA resource name") -> [w1529]
        stop <- w1528 stop-if-true
        n949 = node-c288() -> ()  [unwired: 1 in, 1 out]
        n950 = event shown="[4] \"Inject Pump 1\": Value Change" {
          selector: _ -> [_ _ _ _ _ _ _ _ _]
          dyn-events: _ -> [_ _ _ _ _ _ _ _ _]
          timeout: _ -> [_ _ _ _ _ _ _ _ _]
          tunnel: w1529 -> [w1537 w1633 _ w1709 w1837 w1980 w2025 w2083 w2142]
          tunnel: [_ _ w1708 _ _ _ _ _ _] -> w1528
          event "Flush Pump 1": Value Change {
            w1538 = "\r"
            n951 = event-data() -> ()  [unwired: 1 in, 5 out]
            n952 = call-poly "VISA Configure Serial Port"("VISA resource name"=w1537) -> ("VISA resource name out"=w1551:refnum<visa-resource-name>, "error out"=w1552:errorcluster)  [unwired: 13 in]
            n953 = local read "Write Wait"() -> (w1530:i32)
            n954 = Concatenate Strings("enter pump1", w1538) -> (w1539:string)
            n955 = flat-sequence {
              tunnel: w1552 -> [w1571]
              tunnel: w1551 -> [w1573]
              tunnel: [w1572] -> w1568
              tunnel: [w1570] -> w1567
              tunnel: w1539 -> [w1569]
              tunnel: w1568 -> [w1576]
              tunnel: [w1576] -> w1566
              tunnel: w1567 -> [w1575]
              tunnel: [w1575] -> w1565
              tunnel: w1530 -> [w1574]
              tunnel: [w1581] -> w1564
              tunnel: w1544 -> [w1580]
              tunnel: [w1577] -> w1563
              tunnel: w1566 -> [w1579]
              tunnel: w1565 -> [w1578]
              tunnel: w1564 -> [w1584]
              tunnel: [w1584] -> w1562
              tunnel: [w1583] -> w1561
              tunnel: w1563 -> [w1583]
              tunnel: w1530 -> [w1582]
              tunnel: w1562 -> [w1589]
              tunnel: [w1588] -> w1560
              tunnel: w1547 -> [w1587]
              tunnel: w1561 -> [w1586]
              tunnel: [w1585] -> w1559
              tunnel: w1560 -> [w1592]
              tunnel: [w1592] -> w1558
              tunnel: [w1591] -> w1557
              tunnel: w1559 -> [w1591]
              tunnel: w1530 -> [w1590]
              tunnel: w1558 -> [w1597]
              tunnel: [w1596] -> w1556
              tunnel: w1550 -> [w1595]
              tunnel: w1557 -> [w1594]
              tunnel: [w1593] -> w1555
              tunnel: [w1600] -> w1554
              tunnel: w1556 -> [w1600]
              tunnel: [w1599] -> w1553
              tunnel: w1555 -> [w1599]
              tunnel: w1530 -> [w1598]
              tunnel: w1554 -> [w1605]
              tunnel: w1553 -> [w1602]
              tunnel: [w1604] -> w1533
              tunnel: [w1603] -> w1531
              tunnel: [w1610] -> w1534
              tunnel: w1533 -> [w1610]
              tunnel: [w1609] -> w1532
              tunnel: w1531 -> [w1609]
              tunnel: w1530 -> [w1608]
              tunnel: w1534 -> [w1612]
              tunnel: w1532 -> [w1611]
              frame #0 {
                n956 = VISA Write(VISA resource name=w1573, write buffer=w1569, error in (no error)=w1571) -> (VISA resource name out=w1572:refnum<visa-resource-name>, error out=w1570:errorcluster)  [unwired: 1 out]
              }
              frame #1 {
                n957 = Wait (ms)(milliseconds to wait=w1574) -> ()  [unwired: 1 out]
              }
              frame #2 {
                n958 = VISA Write(VISA resource name=w1579, write buffer=w1580, error in (no error)=w1578) -> (VISA resource name out=w1581:refnum<visa-resource-name>, error out=w1577:errorcluster)  [unwired: 1 out]
              }
              frame #3 {
                n959 = Wait (ms)(milliseconds to wait=w1582) -> ()  [unwired: 1 out]
              }
              frame #4 {
                n960 = VISA Write(VISA resource name=w1589, write buffer=w1587, error in (no error)=w1586) -> (VISA resource name out=w1588:refnum<visa-resource-name>, error out=w1585:errorcluster)  [unwired: 1 out]
              }
              frame #5 {
                n961 = Wait (ms)(milliseconds to wait=w1590) -> ()  [unwired: 1 out]
              }
              frame #6 {
                n962 = VISA Write(VISA resource name=w1597, write buffer=w1595, error in (no error)=w1594) -> (VISA resource name out=w1596:refnum<visa-resource-name>, error out=w1593:errorcluster)  [unwired: 1 out]
              }
              frame #7 {
                n963 = Wait (ms)(milliseconds to wait=w1598) -> ()  [unwired: 1 out]
              }
              frame #8 {
                n964 = Concatenate Strings("start ", "\r") -> (w1601:string)
                n965 = VISA Write(VISA resource name=w1605, write buffer=w1601, error in (no error)=w1602) -> (VISA resource name out=w1604:refnum<visa-resource-name>, error out=w1603:errorcluster)  [unwired: 1 out]
              }
              frame #9 {
                n966 = Wait (ms)(milliseconds to wait=w1608) -> ()  [unwired: 1 out]
              }
              frame #10 {
                n967 = local write "Flush Pump 1"(FALSE ("Flush Pump 1")) -> ()
                n968 = Concatenate Strings("enter main ", "\r") -> (w1616:string)
                n969 = VISA Write(VISA resource name=w1612, write buffer=w1616, error in (no error)=w1611) -> (VISA resource name out=w1615:refnum<visa-resource-name>, error out=w1614:errorcluster)  [unwired: 1 out]
                n970 = VISA Close(VISA resource name=w1615, error in (no error)=w1614) -> ()  [unwired: 1 out]
              }
            }
            n971 = Concatenate Strings("set units 4 ", w1538) -> (w1544:string)
            n972 = Multiply(x="Flush\nRate (ul/min)", y=60) -> (x*y=w1542:dbl)
            n973 = Number To Decimal String(number=w1542) -> (decimal integer string=w1545:string)  [unwired: 1 in]
            n974 = Concatenate Strings("set rate ", w1545, w1538) -> (w1547:string)
            n975 = Number To Decimal String(number="Flush\nVolume (ul)") -> (decimal integer string=w1549:string)  [unwired: 1 in]
            n976 = Concatenate Strings("set volume ", w1549, w1538) -> (w1550:string)
          }
          event "Flush Pump 2": Value Change {
            w1624 = "\r"
            n977 = event-data() -> ()  [unwired: 1 in, 5 out]
            n978 = call-poly "VISA Configure Serial Port"("VISA resource name"=w1633) -> ("VISA resource name out"=w1644:refnum<visa-resource-name>, "error out"=w1645:errorcluster)  [unwired: 13 in]
            n979 = local read "Write Wait"() -> (w1619:i32)
            n980 = Concatenate Strings("enter pump2", w1624) -> (w1625:string)
            n981 = flat-sequence {
              tunnel: w1645 -> [w1660]
              tunnel: w1644 -> [w1662]
              tunnel: [w1661] -> w1630
              tunnel: [w1659] -> w1628
              tunnel: w1625 -> [w1658]
              tunnel: w1630 -> [w1665]
              tunnel: [w1665] -> w1629
              tunnel: w1628 -> [w1664]
              tunnel: [w1664] -> w1627
              tunnel: w1619 -> [w1663]
              tunnel: [w1670] -> w1657
              tunnel: w1637 -> [w1669]
              tunnel: [w1666] -> w1656
              tunnel: w1629 -> [w1668]
              tunnel: w1627 -> [w1667]
              tunnel: w1657 -> [w1673]
              tunnel: [w1673] -> w1655
              tunnel: [w1672] -> w1654
              tunnel: w1656 -> [w1672]
              tunnel: w1619 -> [w1671]
              tunnel: w1655 -> [w1678]
              tunnel: [w1677] -> w1653
              tunnel: w1640 -> [w1676]
              tunnel: w1654 -> [w1675]
              tunnel: [w1674] -> w1652
              tunnel: w1653 -> [w1681]
              tunnel: [w1681] -> w1651
              tunnel: [w1680] -> w1650
              tunnel: w1652 -> [w1680]
              tunnel: w1619 -> [w1679]
              tunnel: w1651 -> [w1686]
              tunnel: [w1685] -> w1649
              tunnel: w1643 -> [w1684]
              tunnel: w1650 -> [w1683]
              tunnel: [w1682] -> w1648
              tunnel: [w1689] -> w1647
              tunnel: w1649 -> [w1689]
              tunnel: [w1688] -> w1646
              tunnel: w1648 -> [w1688]
              tunnel: w1619 -> [w1687]
              tunnel: w1647 -> [w1696]
              tunnel: w1646 -> [w1695]
              tunnel: [w1691] -> w1623
              tunnel: [w1690] -> w1621
              tunnel: w1623 -> [w1699]
              tunnel: [w1699] -> w1622
              tunnel: w1621 -> [w1698]
              tunnel: [w1698] -> w1620
              tunnel: w1619 -> [w1697]
              tunnel: w1622 -> [w1703]
              tunnel: w1620 -> [w1702]
              frame #0 {
                n982 = VISA Write(VISA resource name=w1662, write buffer=w1658, error in (no error)=w1660) -> (VISA resource name out=w1661:refnum<visa-resource-name>, error out=w1659:errorcluster)  [unwired: 1 out]
              }
              frame #1 {
                n983 = Wait (ms)(milliseconds to wait=w1663) -> ()  [unwired: 1 out]
              }
              frame #2 {
                n984 = VISA Write(VISA resource name=w1668, write buffer=w1669, error in (no error)=w1667) -> (VISA resource name out=w1670:refnum<visa-resource-name>, error out=w1666:errorcluster)  [unwired: 1 out]
              }
              frame #3 {
                n985 = Wait (ms)(milliseconds to wait=w1671) -> ()  [unwired: 1 out]
              }
              frame #4 {
                n986 = VISA Write(VISA resource name=w1678, write buffer=w1676, error in (no error)=w1675) -> (VISA resource name out=w1677:refnum<visa-resource-name>, error out=w1674:errorcluster)  [unwired: 1 out]
              }
              frame #5 {
                n987 = Wait (ms)(milliseconds to wait=w1679) -> ()  [unwired: 1 out]
              }
              frame #6 {
                n988 = VISA Write(VISA resource name=w1686, write buffer=w1684, error in (no error)=w1683) -> (VISA resource name out=w1685:refnum<visa-resource-name>, error out=w1682:errorcluster)  [unwired: 1 out]
              }
              frame #7 {
                n989 = Wait (ms)(milliseconds to wait=w1687) -> ()  [unwired: 1 out]
              }
              frame #8 {
                n990 = Concatenate Strings("start ", "\r") -> (w1694:string)
                n991 = VISA Write(VISA resource name=w1696, write buffer=w1694, error in (no error)=w1695) -> (VISA resource name out=w1691:refnum<visa-resource-name>, error out=w1690:errorcluster)  [unwired: 1 out]
              }
              frame #9 {
                n992 = Wait (ms)(milliseconds to wait=w1697) -> ()  [unwired: 1 out]
              }
              frame #10 {
                n993 = local write "Flush Pump 2"(FALSE ("Flush Pump 1")) -> ()
                n994 = Concatenate Strings("enter main ", "\r") -> (w1704:string)
                n995 = VISA Write(VISA resource name=w1703, write buffer=w1704, error in (no error)=w1702) -> (VISA resource name out=w1701:refnum<visa-resource-name>, error out=w1700:errorcluster)  [unwired: 1 out]
                n996 = VISA Close(VISA resource name=w1701, error in (no error)=w1700) -> ()  [unwired: 1 out]
              }
            }
            n997 = Concatenate Strings("set units 4 ", w1624) -> (w1637:string)
            n998 = Multiply(x="Flush \nRate (ul/min)  2", y=60) -> (x*y=w1635:dbl)
            n999 = Number To Decimal String(number=w1635) -> (decimal integer string=w1638:string)  [unwired: 1 in]
            n1000 = Concatenate Strings("set rate ", w1638, w1624) -> (w1640:string)
            n1001 = Number To Decimal String(number="Flush\nVolume (ul)  2") -> (decimal integer string=w1642:string)  [unwired: 1 in]
            n1002 = Concatenate Strings("set volume ", w1642, w1624) -> (w1643:string)
          }
          event "Stop": Value Change {
            n1003 = event-data() -> ()  [unwired: 1 in, 5 out]
            n1004 = local read "Stop"() -> (w1708:bool)
          }
          event "Inject Pump 2": Value Change {
            n1005 = event-data() -> ()  [unwired: 1 in, 5 out]
            n1006 = case shown="True" "Inject Pump 2" {
              tunnel: w1709 -> [w1712 w1754]
              frame False {
                n1007 = local read "Write Wait"() -> (w1711:i32)
                n1008 = call-poly "VISA Configure Serial Port"("VISA resource name"=w1712) -> ("VISA resource name out"=w1716:refnum<visa-resource-name>, "error out"=w1717:errorcluster)  [unwired: 13 in]
                n1009 = Concatenate Strings("enter pump2", "\r") -> (w1714:string)
                n1010 = flat-sequence {
                  tunnel: w1717 -> [w1728]
                  tunnel: w1716 -> [w1730]
                  tunnel: [w1729] -> w1725
                  tunnel: [w1727] -> w1724
                  tunnel: w1714 -> [w1726]
                  tunnel: w1725 -> [w1733]
                  tunnel: w1724 -> [w1732]
                  tunnel: [w1733] -> w1723
                  tunnel: [w1732] -> w1722
                  tunnel: w1711 -> [w1731]
                  tunnel: [w1737] -> w1721
                  tunnel: [w1736] -> w1720
                  tunnel: w1723 -> [w1735]
                  tunnel: w1722 -> [w1734]
                  tunnel: w1721 -> [w1743]
                  tunnel: [w1743] -> w1719
                  tunnel: w1720 -> [w1742]
                  tunnel: [w1742] -> w1718
                  tunnel: w1711 -> [w1741]
                  tunnel: w1719 -> [w1747]
                  tunnel: w1718 -> [w1746]
                  frame #0 {
                    n1011 = VISA Write(VISA resource name=w1730, write buffer=w1726, error in (no error)=w1728) -> (VISA resource name out=w1729:refnum<visa-resource-name>, error out=w1727:errorcluster)  [unwired: 1 out]
                  }
                  frame #1 {
                    n1012 = Wait (ms)(milliseconds to wait=w1731) -> ()  [unwired: 1 out]
                  }
                  frame #2 {
                    n1013 = Concatenate Strings("stop ", "\r") -> (w1740:string)
                    n1014 = VISA Write(VISA resource name=w1735, write buffer=w1740, error in (no error)=w1734) -> (VISA resource name out=w1737:refnum<visa-resource-name>, error out=w1736:errorcluster)  [unwired: 1 out]
                  }
                  frame #3 {
                    n1015 = Wait (ms)(milliseconds to wait=w1741) -> ()  [unwired: 1 out]
                  }
                  frame #4 {
                    n1016 = Concatenate Strings("enter main ", "\r") -> (w1748:string)
                    n1017 = VISA Write(VISA resource name=w1747, write buffer=w1748, error in (no error)=w1746) -> (VISA resource name out=w1745:refnum<visa-resource-name>, error out=w1744:errorcluster)  [unwired: 1 out]
                    n1018 = VISA Close(VISA resource name=w1745, error in (no error)=w1744) -> ()  [unwired: 1 out]
                  }
                }
              }
              frame True {
                w1767 = "\r"
                n1019 = call-poly "VISA Configure Serial Port"("VISA resource name"=w1754) -> ("VISA resource name out"=w1756:refnum<visa-resource-name>, "error out"=w1755:errorcluster)  [unwired: 13 in]
                n1020 = local read "Write Wait"() -> (w1751:i32)
                n1021 = Concatenate Strings("enter pump2", w1767) -> (w1766:string)
                n1022 = flat-sequence {
                  tunnel: w1755 -> [w1790]
                  tunnel: w1756 -> [w1792]
                  tunnel: [w1791] -> w1787
                  tunnel: [w1789] -> w1786
                  tunnel: w1766 -> [w1788]
                  tunnel: w1787 -> [w1795]
                  tunnel: [w1795] -> w1785
                  tunnel: w1786 -> [w1794]
                  tunnel: [w1794] -> w1784
                  tunnel: w1751 -> [w1793]
                  tunnel: [w1800] -> w1783
                  tunnel: w1763 -> [w1799]
                  tunnel: [w1796] -> w1782
                  tunnel: w1785 -> [w1798]
                  tunnel: w1784 -> [w1797]
                  tunnel: w1783 -> [w1803]
                  tunnel: [w1803] -> w1781
                  tunnel: [w1802] -> w1780
                  tunnel: w1782 -> [w1802]
                  tunnel: w1751 -> [w1801]
                  tunnel: w1781 -> [w1808]
                  tunnel: [w1807] -> w1779
                  tunnel: w1760 -> [w1806]
                  tunnel: w1780 -> [w1805]
                  tunnel: [w1804] -> w1778
                  tunnel: w1779 -> [w1811]
                  tunnel: [w1811] -> w1777
                  tunnel: [w1810] -> w1776
                  tunnel: w1778 -> [w1810]
                  tunnel: w1751 -> [w1809]
                  tunnel: w1777 -> [w1816]
                  tunnel: [w1815] -> w1775
                  tunnel: w1757 -> [w1814]
                  tunnel: w1776 -> [w1813]
                  tunnel: [w1812] -> w1774
                  tunnel: [w1819] -> w1773
                  tunnel: w1775 -> [w1819]
                  tunnel: [w1818] -> w1772
                  tunnel: w1774 -> [w1818]
                  tunnel: w1751 -> [w1817]
                  tunnel: w1773 -> [w1826]
                  tunnel: w1772 -> [w1825]
                  tunnel: [w1821] -> w1771
                  tunnel: [w1820] -> w1770
                  tunnel: w1771 -> [w1829]
                  tunnel: [w1829] -> w1769
                  tunnel: w1770 -> [w1828]
                  tunnel: [w1828] -> w1768
                  tunnel: w1751 -> [w1827]
                  tunnel: w1769 -> [w1833]
                  tunnel: w1768 -> [w1832]
                  frame #0 {
                    n1023 = VISA Write(VISA resource name=w1792, write buffer=w1788, error in (no error)=w1790) -> (VISA resource name out=w1791:refnum<visa-resource-name>, error out=w1789:errorcluster)  [unwired: 1 out]
                  }
                  frame #1 {
                    n1024 = Wait (ms)(milliseconds to wait=w1793) -> ()  [unwired: 1 out]
                  }
                  frame #2 {
                    n1025 = VISA Write(VISA resource name=w1798, write buffer=w1799, error in (no error)=w1797) -> (VISA resource name out=w1800:refnum<visa-resource-name>, error out=w1796:errorcluster)  [unwired: 1 out]
                  }
                  frame #3 {
                    n1026 = Wait (ms)(milliseconds to wait=w1801) -> ()  [unwired: 1 out]
                  }
                  frame #4 {
                    n1027 = VISA Write(VISA resource name=w1808, write buffer=w1806, error in (no error)=w1805) -> (VISA resource name out=w1807:refnum<visa-resource-name>, error out=w1804:errorcluster)  [unwired: 1 out]
                  }
                  frame #5 {
                    n1028 = Wait (ms)(milliseconds to wait=w1809) -> ()  [unwired: 1 out]
                  }
                  frame #6 {
                    n1029 = VISA Write(VISA resource name=w1816, write buffer=w1814, error in (no error)=w1813) -> (VISA resource name out=w1815:refnum<visa-resource-name>, error out=w1812:errorcluster)  [unwired: 1 out]
                  }
                  frame #7 {
                    n1030 = Wait (ms)(milliseconds to wait=w1817) -> ()  [unwired: 1 out]
                  }
                  frame #8 {
                    n1031 = Concatenate Strings("start ", "\r") -> (w1824:string)
                    n1032 = VISA Write(VISA resource name=w1826, write buffer=w1824, error in (no error)=w1825) -> (VISA resource name out=w1821:refnum<visa-resource-name>, error out=w1820:errorcluster)  [unwired: 1 out]
                  }
                  frame #9 {
                    n1033 = Wait (ms)(milliseconds to wait=w1827) -> ()  [unwired: 1 out]
                  }
                  frame #10 {
                    n1034 = Concatenate Strings("enter main ", "\r") -> (w1834:string)
                    n1035 = VISA Write(VISA resource name=w1833, write buffer=w1834, error in (no error)=w1832) -> (VISA resource name out=w1831:refnum<visa-resource-name>, error out=w1830:errorcluster)  [unwired: 1 out]
                    n1036 = VISA Close(VISA resource name=w1831, error in (no error)=w1830) -> ()  [unwired: 1 out]
                  }
                }
                n1037 = local read "Normal \nRate (ul/hr)  2"() -> (w1752:dbl)
                n1038 = Concatenate Strings("set units 4 ", w1767) -> (w1763:string)
                n1039 = local read "Normal \nVolume (ul) 2"() -> (w1753:dbl)
                n1040 = Number To Decimal String(number=w1752) -> (decimal integer string=w1762:string)  [unwired: 1 in]
                n1041 = Concatenate Strings("set rate ", w1762, w1767) -> (w1760:string)
                n1042 = Number To Decimal String(number=w1753) -> (decimal integer string=w1758:string)  [unwired: 1 in]
                n1043 = Concatenate Strings("set volume ", w1758, w1767) -> (w1757:string)
              }
            }
          }
          event "Inject Pump 1": Value Change {
            n1044 = event-data() -> ()  [unwired: 1 in, 5 out]
            n1045 = case shown="True" "Inject Pump 1" {
              tunnel: w1837 -> [w1840 w1882]
              frame False {
                n1046 = local read "Write Wait"() -> (w1839:i32)
                n1047 = call-poly "VISA Configure Serial Port"("VISA resource name"=w1840) -> ("VISA resource name out"=w1844:refnum<visa-resource-name>, "error out"=w1845:errorcluster)  [unwired: 13 in]
                n1048 = Concatenate Strings("enter pump1", "\r") -> (w1842:string)
                n1049 = flat-sequence {
                  tunnel: w1845 -> [w1856]
                  tunnel: w1844 -> [w1858]
                  tunnel: [w1857] -> w1853
                  tunnel: [w1855] -> w1852
                  tunnel: w1842 -> [w1854]
                  tunnel: w1853 -> [w1861]
                  tunnel: w1852 -> [w1860]
                  tunnel: [w1861] -> w1851
                  tunnel: [w1860] -> w1850
                  tunnel: w1839 -> [w1859]
                  tunnel: [w1865] -> w1849
                  tunnel: [w1864] -> w1848
                  tunnel: w1851 -> [w1863]
                  tunnel: w1850 -> [w1862]
                  tunnel: w1849 -> [w1871]
                  tunnel: [w1871] -> w1847
                  tunnel: w1848 -> [w1870]
                  tunnel: [w1870] -> w1846
                  tunnel: w1839 -> [w1869]
                  tunnel: w1847 -> [w1875]
                  tunnel: w1846 -> [w1874]
                  frame #0 {
                    n1050 = VISA Write(VISA resource name=w1858, write buffer=w1854, error in (no error)=w1856) -> (VISA resource name out=w1857:refnum<visa-resource-name>, error out=w1855:errorcluster)  [unwired: 1 out]
                  }
                  frame #1 {
                    n1051 = Wait (ms)(milliseconds to wait=w1859) -> ()  [unwired: 1 out]
                  }
                  frame #2 {
                    n1052 = Concatenate Strings("stop ", "\r") -> (w1868:string)
                    n1053 = VISA Write(VISA resource name=w1863, write buffer=w1868, error in (no error)=w1862) -> (VISA resource name out=w1865:refnum<visa-resource-name>, error out=w1864:errorcluster)  [unwired: 1 out]
                  }
                  frame #3 {
                    n1054 = Wait (ms)(milliseconds to wait=w1869) -> ()  [unwired: 1 out]
                  }
                  frame #4 {
                    n1055 = Concatenate Strings("enter main ", "\r") -> (w1876:string)
                    n1056 = VISA Write(VISA resource name=w1875, write buffer=w1876, error in (no error)=w1874) -> (VISA resource name out=w1873:refnum<visa-resource-name>, error out=w1872:errorcluster)  [unwired: 1 out]
                    n1057 = VISA Close(VISA resource name=w1873, error in (no error)=w1872) -> ()  [unwired: 1 out]
                  }
                }
              }
              frame True {
                w1895 = "\r"
                n1058 = call-poly "VISA Configure Serial Port"("VISA resource name"=w1882) -> ("VISA resource name out"=w1884:refnum<visa-resource-name>, "error out"=w1883:errorcluster)  [unwired: 13 in]
                n1059 = local read "Write Wait"() -> (w1879:i32)
                n1060 = flat-sequence {
                  tunnel: w1883 -> [w1918]
                  tunnel: w1884 -> [w1920]
                  tunnel: [w1919] -> w1915
                  tunnel: [w1917] -> w1914
                  tunnel: w1894 -> [w1916]
                  tunnel: w1915 -> [w1923]
                  tunnel: [w1923] -> w1913
                  tunnel: w1914 -> [w1922]
                  tunnel: [w1922] -> w1912
                  tunnel: w1879 -> [w1921]
                  tunnel: [w1928] -> w1911
                  tunnel: w1891 -> [w1927]
                  tunnel: [w1924] -> w1910
                  tunnel: w1913 -> [w1926]
                  tunnel: w1912 -> [w1925]
                  tunnel: w1911 -> [w1931]
                  tunnel: [w1931] -> w1909
                  tunnel: [w1930] -> w1908
                  tunnel: w1910 -> [w1930]
                  tunnel: w1879 -> [w1929]
                  tunnel: w1909 -> [w1936]
                  tunnel: [w1935] -> w1907
                  tunnel: w1888 -> [w1934]
                  tunnel: w1908 -> [w1933]
                  tunnel: [w1932] -> w1906
                  tunnel: w1907 -> [w1939]
                  tunnel: [w1939] -> w1905
                  tunnel: [w1938] -> w1904
                  tunnel: w1906 -> [w1938]
                  tunnel: w1879 -> [w1937]
                  tunnel: w1905 -> [w1944]
                  tunnel: [w1943] -> w1903
                  tunnel: w1885 -> [w1942]
                  tunnel: w1904 -> [w1941]
                  tunnel: [w1940] -> w1902
                  tunnel: [w1947] -> w1901
                  tunnel: w1903 -> [w1947]
                  tunnel: [w1946] -> w1900
                  tunnel: w1902 -> [w1946]
                  tunnel: w1879 -> [w1945]
                  tunnel: w1901 -> [w1954]
                  tunnel: w1900 -> [w1953]
                  tunnel: [w1949] -> w1899
                  tunnel: [w1948] -> w1898
                  tunnel: w1899 -> [w1957]
                  tunnel: [w1957] -> w1897
                  tunnel: w1898 -> [w1956]
                  tunnel: [w1956] -> w1896
                  tunnel: w1879 -> [w1955]
                  tunnel: w1897 -> [w1961]
                  tunnel: w1896 -> [w1960]
                  frame #0 {
                    n1061 = VISA Write(VISA resource name=w1920, write buffer=w1916, error in (no error)=w1918) -> (VISA resource name out=w1919:refnum<visa-resource-name>, error out=w1917:errorcluster)  [unwired: 1 out]
                  }
                  frame #1 {
                    n1062 = Wait (ms)(milliseconds to wait=w1921) -> ()  [unwired: 1 out]
                  }
                  frame #2 {
                    n1063 = VISA Write(VISA resource name=w1926, write buffer=w1927, error in (no error)=w1925) -> (VISA resource name out=w1928:refnum<visa-resource-name>, error out=w1924:errorcluster)  [unwired: 1 out]
                  }
                  frame #3 {
                    n1064 = Wait (ms)(milliseconds to wait=w1929) -> ()  [unwired: 1 out]
                  }
                  frame #4 {
                    n1065 = VISA Write(VISA resource name=w1936, write buffer=w1934, error in (no error)=w1933) -> (VISA resource name out=w1935:refnum<visa-resource-name>, error out=w1932:errorcluster)  [unwired: 1 out]
                  }
                  frame #5 {
                    n1066 = Wait (ms)(milliseconds to wait=w1937) -> ()  [unwired: 1 out]
                  }
                  frame #6 {
                    n1067 = VISA Write(VISA resource name=w1944, write buffer=w1942, error in (no error)=w1941) -> (VISA resource name out=w1943:refnum<visa-resource-name>, error out=w1940:errorcluster)  [unwired: 1 out]
                  }
                  frame #7 {
                    n1068 = Wait (ms)(milliseconds to wait=w1945) -> ()  [unwired: 1 out]
                  }
                  frame #8 {
                    n1069 = Concatenate Strings("start ", "\r") -> (w1952:string)
                    n1070 = VISA Write(VISA resource name=w1954, write buffer=w1952, error in (no error)=w1953) -> (VISA resource name out=w1949:refnum<visa-resource-name>, error out=w1948:errorcluster)  [unwired: 1 out]
                  }
                  frame #9 {
                    n1071 = Wait (ms)(milliseconds to wait=w1955) -> ()  [unwired: 1 out]
                  }
                  frame #10 {
                    n1072 = Concatenate Strings("enter main ", "\r") -> (w1962:string)
                    n1073 = VISA Write(VISA resource name=w1961, write buffer=w1962, error in (no error)=w1960) -> (VISA resource name out=w1959:refnum<visa-resource-name>, error out=w1958:errorcluster)  [unwired: 1 out]
                    n1074 = VISA Close(VISA resource name=w1959, error in (no error)=w1958) -> ()  [unwired: 1 out]
                  }
                }
                n1075 = Concatenate Strings("enter pump1", w1895) -> (w1894:string)
                n1076 = local read "Normal \nRate (ul/hr)"() -> (w1880:dbl)
                n1077 = Concatenate Strings("set units 4 ", w1895) -> (w1891:string)
                n1078 = local read "Normal \nVolume (ul)"() -> (w1881:dbl)
                n1079 = Number To Decimal String(number=w1880) -> (decimal integer string=w1890:string)  [unwired: 1 in]
                n1080 = Concatenate Strings("set rate ", w1890, w1895) -> (w1888:string)
                n1081 = Number To Decimal String(number=w1881) -> (decimal integer string=w1886:string)  [unwired: 1 in]
                n1082 = Concatenate Strings("set volume ", w1886, w1895) -> (w1885:string)
              }
            }
          }
          event "Normal \nVolume (ul)": Value Change {
            n1083 = event-data() -> ()  [unwired: 1 in, 5 out]
            n1084 = call-poly "VISA Configure Serial Port"("VISA resource name"=w1980) -> ("VISA resource name out"=w1982:refnum<visa-resource-name>, "error out"=w1981:errorcluster)  [unwired: 13 in]
            n1085 = local read "Write Wait"() -> (w1965:i32)
            n1086 = Concatenate Strings("enter pump1", "\r") -> (w1984:string)
            n1087 = flat-sequence {
              tunnel: w1981 -> [w1994]
              tunnel: w1982 -> [w1996]
              tunnel: [w1995] -> w1974
              tunnel: [w1993] -> w1973
              tunnel: w1984 -> [w1992]
              tunnel: w1974 -> [w1999]
              tunnel: [w1999] -> w1972
              tunnel: w1973 -> [w1998]
              tunnel: [w1998] -> w1970
              tunnel: w1965 -> [w1997]
              tunnel: w1972 -> [w2003]
              tunnel: [w2004] -> w1971
              tunnel: w1970 -> [w2002]
              tunnel: [w2001] -> w1969
              tunnel: w1966 -> [w2000]
              tunnel: w1971 -> [w2007]
              tunnel: w1969 -> [w2006]
              tunnel: [w2007] -> w1991
              tunnel: [w2006] -> w1990
              tunnel: w1965 -> [w2005]
              tunnel: [w2012] -> w1989
              tunnel: [w2011] -> w1988
              tunnel: w1991 -> [w2010]
              tunnel: w1990 -> [w2009]
              tunnel: w1975 -> [w2008]
              tunnel: w1989 -> [w2015]
              tunnel: [w2015] -> w1987
              tunnel: w1988 -> [w2014]
              tunnel: [w2014] -> w1986
              tunnel: w1965 -> [w2013]
              tunnel: w1987 -> [w2019]
              tunnel: w1986 -> [w2018]
              frame #0 {
                n1088 = VISA Write(VISA resource name=w1996, write buffer=w1992, error in (no error)=w1994) -> (VISA resource name out=w1995:refnum<visa-resource-name>, error out=w1993:errorcluster)  [unwired: 1 out]
              }
              frame #1 {
                n1089 = Wait (ms)(milliseconds to wait=w1997) -> ()  [unwired: 1 out]
              }
              frame #2 {
                n1090 = VISA Write(VISA resource name=w2003, write buffer=w2000, error in (no error)=w2002) -> (VISA resource name out=w2004:refnum<visa-resource-name>, error out=w2001:errorcluster)  [unwired: 1 out]
              }
              frame #3 {
                n1091 = Wait (ms)(milliseconds to wait=w2005) -> ()  [unwired: 1 out]
              }
              frame #4 {
                n1092 = VISA Write(VISA resource name=w2010, write buffer=w2008, error in (no error)=w2009) -> (VISA resource name out=w2012:refnum<visa-resource-name>, error out=w2011:errorcluster)  [unwired: 1 out]
              }
              frame #5 {
                n1093 = Wait (ms)(milliseconds to wait=w2013) -> ()  [unwired: 1 out]
              }
              frame #6 {
                n1094 = Concatenate Strings("enter main ", "\r") -> (w2020:string)
                n1095 = VISA Write(VISA resource name=w2019, write buffer=w2020, error in (no error)=w2018) -> (VISA resource name out=w2017:refnum<visa-resource-name>, error out=w2016:errorcluster)  [unwired: 1 out]
                n1096 = VISA Close(VISA resource name=w2017, error in (no error)=w2016) -> ()  [unwired: 1 out]
              }
            }
            n1097 = Concatenate Strings("set units 4", "\r") -> (w1966:string)
            n1098 = Number To Decimal String(number="Normal \nVolume (ul)") -> (decimal integer string=w1977:string)  [unwired: 1 in]
            n1099 = Concatenate Strings("set volume", w1977, "\r") -> (w1975:string)
          }
          event "Normal \nRate (ul/hr)": Value Change {
            n1100 = event-data() -> ()  [unwired: 1 in, 5 out]
            n1101 = call-poly "VISA Configure Serial Port"("VISA resource name"=w2025) -> ("VISA resource name out"=w2033:refnum<visa-resource-name>, "error out"=w2032:errorcluster)  [unwired: 13 in]
            n1102 = local read "Write Wait"() -> (w2023:i32)
            n1103 = Concatenate Strings("enter pump1", "\r") -> (w2035:string)
            n1104 = flat-sequence {
              tunnel: w2032 -> [w2052]
              tunnel: w2033 -> [w2054]
              tunnel: [w2053] -> w2048
              tunnel: [w2051] -> w2047
              tunnel: w2035 -> [w2050]
              tunnel: w2048 -> [w2057]
              tunnel: [w2057] -> w2046
              tunnel: w2047 -> [w2056]
              tunnel: [w2056] -> w2045
              tunnel: w2023 -> [w2055]
              tunnel: w2046 -> [w2061]
              tunnel: [w2062] -> w2044
              tunnel: w2045 -> [w2060]
              tunnel: [w2059] -> w2043
              tunnel: w2026 -> [w2058]
              tunnel: w2044 -> [w2065]
              tunnel: w2043 -> [w2064]
              tunnel: [w2065] -> w2042
              tunnel: [w2064] -> w2041
              tunnel: w2023 -> [w2063]
              tunnel: [w2070] -> w2040
              tunnel: [w2069] -> w2039
              tunnel: w2042 -> [w2068]
              tunnel: w2041 -> [w2067]
              tunnel: w2029 -> [w2066]
              tunnel: w2040 -> [w2073]
              tunnel: [w2073] -> w2038
              tunnel: w2039 -> [w2072]
              tunnel: [w2072] -> w2037
              tunnel: w2023 -> [w2071]
              tunnel: w2038 -> [w2077]
              tunnel: w2037 -> [w2076]
              frame #0 {
                n1105 = VISA Write(VISA resource name=w2054, write buffer=w2050, error in (no error)=w2052) -> (VISA resource name out=w2053:refnum<visa-resource-name>, error out=w2051:errorcluster)  [unwired: 1 out]
              }
              frame #1 {
                n1106 = Wait (ms)(milliseconds to wait=w2055) -> ()  [unwired: 1 out]
              }
              frame #2 {
                n1107 = VISA Write(VISA resource name=w2061, write buffer=w2058, error in (no error)=w2060) -> (VISA resource name out=w2062:refnum<visa-resource-name>, error out=w2059:errorcluster)  [unwired: 1 out]
              }
              frame #3 {
                n1108 = Wait (ms)(milliseconds to wait=w2063) -> ()  [unwired: 1 out]
              }
              frame #4 {
                n1109 = VISA Write(VISA resource name=w2068, write buffer=w2066, error in (no error)=w2067) -> (VISA resource name out=w2070:refnum<visa-resource-name>, error out=w2069:errorcluster)  [unwired: 1 out]
              }
              frame #5 {
                n1110 = Wait (ms)(milliseconds to wait=w2071) -> ()  [unwired: 1 out]
              }
              frame #6 {
                n1111 = Concatenate Strings("enter main ", "\r") -> (w2078:string)
                n1112 = VISA Write(VISA resource name=w2077, write buffer=w2078, error in (no error)=w2076) -> (VISA resource name out=w2075:refnum<visa-resource-name>, error out=w2074:errorcluster)  [unwired: 1 out]
                n1113 = VISA Close(VISA resource name=w2075, error in (no error)=w2074) -> ()  [unwired: 1 out]
              }
            }
            n1114 = Concatenate Strings("set units 4", "\r") -> (w2026:string)
            n1115 = Number To Decimal String(number="Normal \nRate (ul/hr)") -> (decimal integer string=w2024:string)  [unwired: 1 in]
            n1116 = Concatenate Strings("set rate", w2024, "\r") -> (w2029:string)
          }
          event "Normal \nRate (ul/hr)  2": Value Change {
            n1117 = event-data() -> ()  [unwired: 1 in, 5 out]
            n1118 = call-poly "VISA Configure Serial Port"("VISA resource name"=w2083) -> ("VISA resource name out"=w2091:refnum<visa-resource-name>, "error out"=w2090:errorcluster)  [unwired: 13 in]
            n1119 = local read "Write Wait"() -> (w2081:i32)
            n1120 = Concatenate Strings("enter pump2", "\r") -> (w2093:string)
            n1121 = flat-sequence {
              tunnel: w2090 -> [w2110]
              tunnel: w2091 -> [w2112]
              tunnel: [w2111] -> w2106
              tunnel: [w2109] -> w2105
              tunnel: w2093 -> [w2108]
              tunnel: w2106 -> [w2115]
              tunnel: [w2115] -> w2104
              tunnel: w2105 -> [w2114]
              tunnel: [w2114] -> w2103
              tunnel: w2081 -> [w2113]
              tunnel: w2104 -> [w2119]
              tunnel: [w2120] -> w2102
              tunnel: w2103 -> [w2118]
              tunnel: [w2117] -> w2101
              tunnel: w2084 -> [w2116]
              tunnel: w2102 -> [w2123]
              tunnel: w2101 -> [w2122]
              tunnel: [w2123] -> w2100
              tunnel: [w2122] -> w2099
              tunnel: w2081 -> [w2121]
              tunnel: [w2128] -> w2098
              tunnel: [w2127] -> w2097
              tunnel: w2100 -> [w2126]
              tunnel: w2099 -> [w2125]
              tunnel: w2087 -> [w2124]
              tunnel: w2098 -> [w2131]
              tunnel: [w2131] -> w2096
              tunnel: w2097 -> [w2130]
              tunnel: [w2130] -> w2095
              tunnel: w2081 -> [w2129]
              tunnel: w2096 -> [w2135]
              tunnel: w2095 -> [w2134]
              frame #0 {
                n1122 = VISA Write(VISA resource name=w2112, write buffer=w2108, error in (no error)=w2110) -> (VISA resource name out=w2111:refnum<visa-resource-name>, error out=w2109:errorcluster)  [unwired: 1 out]
              }
              frame #1 {
                n1123 = Wait (ms)(milliseconds to wait=w2113) -> ()  [unwired: 1 out]
              }
              frame #2 {
                n1124 = VISA Write(VISA resource name=w2119, write buffer=w2116, error in (no error)=w2118) -> (VISA resource name out=w2120:refnum<visa-resource-name>, error out=w2117:errorcluster)  [unwired: 1 out]
              }
              frame #3 {
                n1125 = Wait (ms)(milliseconds to wait=w2121) -> ()  [unwired: 1 out]
              }
              frame #4 {
                n1126 = VISA Write(VISA resource name=w2126, write buffer=w2124, error in (no error)=w2125) -> (VISA resource name out=w2128:refnum<visa-resource-name>, error out=w2127:errorcluster)  [unwired: 1 out]
              }
              frame #5 {
                n1127 = Wait (ms)(milliseconds to wait=w2129) -> ()  [unwired: 1 out]
              }
              frame #6 {
                n1128 = Concatenate Strings("enter main ", "\r") -> (w2136:string)
                n1129 = VISA Write(VISA resource name=w2135, write buffer=w2136, error in (no error)=w2134) -> (VISA resource name out=w2133:refnum<visa-resource-name>, error out=w2132:errorcluster)  [unwired: 1 out]
                n1130 = VISA Close(VISA resource name=w2133, error in (no error)=w2132) -> ()  [unwired: 1 out]
              }
            }
            n1131 = Concatenate Strings("set units 4", "\r") -> (w2084:string)
            n1132 = Number To Decimal String(number="Normal \nRate (ul/hr)  2") -> (decimal integer string=w2082:string)  [unwired: 1 in]
            n1133 = Concatenate Strings("set rate", w2082, "\r") -> (w2087:string)
          }
          event "Normal \nVolume (ul) 2": Value Change {
            n1134 = event-data() -> ()  [unwired: 1 in, 5 out]
            n1135 = call-poly "VISA Configure Serial Port"("VISA resource name"=w2142) -> ("VISA resource name out"=w2146:refnum<visa-resource-name>, "error out"=w2147:errorcluster)  [unwired: 13 in]
            n1136 = local read "Write Wait"() -> (w2139:i32)
            n1137 = Concatenate Strings("enter pump2", "\r") -> (w2144:string)
            n1138 = flat-sequence {
              tunnel: w2147 -> [w2168]
              tunnel: w2146 -> [w2170]
              tunnel: [w2169] -> w2165
              tunnel: [w2167] -> w2164
              tunnel: w2144 -> [w2166]
              tunnel: w2165 -> [w2173]
              tunnel: [w2173] -> w2163
              tunnel: w2164 -> [w2172]
              tunnel: [w2172] -> w2162
              tunnel: w2139 -> [w2171]
              tunnel: w2163 -> [w2177]
              tunnel: [w2178] -> w2161
              tunnel: w2162 -> [w2176]
              tunnel: [w2175] -> w2160
              tunnel: w2153 -> [w2174]
              tunnel: w2161 -> [w2181]
              tunnel: w2160 -> [w2180]
              tunnel: [w2181] -> w2159
              tunnel: [w2180] -> w2158
              tunnel: w2139 -> [w2179]
              tunnel: [w2186] -> w2157
              tunnel: [w2185] -> w2156
              tunnel: w2159 -> [w2184]
              tunnel: w2158 -> [w2183]
              tunnel: w2150 -> [w2182]
              tunnel: w2157 -> [w2189]
              tunnel: [w2189] -> w2155
              tunnel: w2156 -> [w2188]
              tunnel: [w2188] -> w2154
              tunnel: w2139 -> [w2187]
              tunnel: w2155 -> [w2193]
              tunnel: w2154 -> [w2192]
              frame #0 {
                n1139 = VISA Write(VISA resource name=w2170, write buffer=w2166, error in (no error)=w2168) -> (VISA resource name out=w2169:refnum<visa-resource-name>, error out=w2167:errorcluster)  [unwired: 1 out]
              }
              frame #1 {
                n1140 = Wait (ms)(milliseconds to wait=w2171) -> ()  [unwired: 1 out]
              }
              frame #2 {
                n1141 = VISA Write(VISA resource name=w2177, write buffer=w2174, error in (no error)=w2176) -> (VISA resource name out=w2178:refnum<visa-resource-name>, error out=w2175:errorcluster)  [unwired: 1 out]
              }
              frame #3 {
                n1142 = Wait (ms)(milliseconds to wait=w2179) -> ()  [unwired: 1 out]
              }
              frame #4 {
                n1143 = VISA Write(VISA resource name=w2184, write buffer=w2182, error in (no error)=w2183) -> (VISA resource name out=w2186:refnum<visa-resource-name>, error out=w2185:errorcluster)  [unwired: 1 out]
              }
              frame #5 {
                n1144 = Wait (ms)(milliseconds to wait=w2187) -> ()  [unwired: 1 out]
              }
              frame #6 {
                n1145 = Concatenate Strings("enter main ", "\r") -> (w2194:string)
                n1146 = VISA Write(VISA resource name=w2193, write buffer=w2194, error in (no error)=w2192) -> (VISA resource name out=w2191:refnum<visa-resource-name>, error out=w2190:errorcluster)  [unwired: 1 out]
                n1147 = VISA Close(VISA resource name=w2191, error in (no error)=w2190) -> ()  [unwired: 1 out]
              }
            }
            n1148 = Concatenate Strings("set units 4", "\r") -> (w2153:string)
            n1149 = Number To Decimal String(number="Normal \nVolume (ul) 2") -> (decimal integer string=w2140:string)  [unwired: 1 in]
            n1150 = Concatenate Strings("set volume", w2140, "\r") -> (w2150:string)
          }
        }
        n1151 = node-c288() -> ()  [unwired: 1 in, 1 out]
      }
      n1152 = node-c288(w1526) -> ()  [unwired: 1 out]
    }
    frame Enabled {
      n1153 = node-c288(2 ("Processor")) -> (w2206:T12)  [unwired: 3 in]
      n1154 = timed-loop "Pump Control" {
        timing: w2206 -> [_]
        timing-out: [_] -> w2205
        tunnel: refnum<visa-resource-name> "COM5" ("VISA resource name") -> [w2208]
        stop <- w2207 stop-if-true
        n1155 = node-c288() -> ()  [unwired: 1 in, 1 out]
        n1156 = event shown="[2] \"Inject Sample\": Value Change" {
          selector: _ -> [_ _ _ _ _]
          dyn-events: _ -> [_ _ _ _ _]
          timeout: _ -> [_ _ _ _ _]
          tunnel: w2208 -> [w2214 _ w2288 w2315 w2320]
          tunnel: [_ w2286 _ _ _] -> w2207
          event "Flush Sample": Value Change {
            n1157 = event-data() -> ()  [unwired: 1 in, 5 out]
            n1158 = local read "Write Wait"() -> (w2228:i32)
            n1159 = flat-sequence {
              tunnel: [w2252] -> w2248
              tunnel: [w2251] -> w2247
              tunnel: "CLD" -> [w2250]
              tunnel: w2214 -> [w2249]
              tunnel: w2248 -> [w2255]
              tunnel: [w2255] -> w2246
              tunnel: w2247 -> [w2254]
              tunnel: [w2254] -> w2245
              tunnel: w2228 -> [w2253]
              tunnel: [w2260] -> w2244
              tunnel: [w2257] -> w2243
              tunnel: w2246 -> [w2259]
              tunnel: w2245 -> [w2258]
              tunnel: "MODVOL" -> [w2256]
              tunnel: w2244 -> [w2263]
              tunnel: [w2263] -> w2242
              tunnel: [w2262] -> w2241
              tunnel: w2243 -> [w2262]
              tunnel: w2228 -> [w2261]
              tunnel: w2242 -> [w2268]
              tunnel: [w2267] -> w2240
              tunnel: w2230 -> [w2266]
              tunnel: w2241 -> [w2265]
              tunnel: [w2264] -> w2239
              tunnel: w2240 -> [w2271]
              tunnel: [w2271] -> w2238
              tunnel: [w2270] -> w2237
              tunnel: w2239 -> [w2270]
              tunnel: w2228 -> [w2269]
              tunnel: w2238 -> [w2276]
              tunnel: [w2275] -> w2236
              tunnel: w2232 -> [w2274]
              tunnel: w2237 -> [w2273]
              tunnel: [w2272] -> w2235
              tunnel: [w2279] -> w2233
              tunnel: w2236 -> [w2279]
              tunnel: [w2278] -> w2234
              tunnel: w2235 -> [w2278]
              tunnel: w2228 -> [w2277]
              tunnel: w2234 -> [w2284]
              tunnel: w2233 -> [w2285]
              tunnel: [w2283] -> w2223
              tunnel: "RUN " -> [w2282]
              frame #0 {
                n1160 = call "Write to pump 2.vi"("String to write"=w2250, "VISA resource name"=w2249) -> ("error out"=w2251:errorcluster, "VISA resource name out"=w2252:refnum<visa-resource-name>)  [unwired: 8 in]
              }
              frame #1 {
                n1161 = Wait (ms)(milliseconds to wait=w2253) -> ()  [unwired: 1 out]
              }
              frame #2 {
                n1162 = call "Write to pump 2.vi"("error in (no error)"=w2258, "String to write"=w2256, "VISA resource name"=w2259) -> ("error out"=w2257:errorcluster, "VISA resource name out"=w2260:refnum<visa-resource-name>)  [unwired: 7 in]
              }
              frame #3 {
                n1163 = Wait (ms)(milliseconds to wait=w2261) -> ()  [unwired: 1 out]
              }
              frame #4 {
                n1164 = call "Write to pump 2.vi"("error in (no error)"=w2265, "String to write"=w2266, "VISA resource name"=w2268) -> ("error out"=w2264:errorcluster, "VISA resource name out"=w2267:refnum<visa-resource-name>)  [unwired: 7 in]
              }
              frame #5 {
                n1165 = Wait (ms)(milliseconds to wait=w2269) -> ()  [unwired: 1 out]
              }
              frame #6 {
                n1166 = call "Write to pump 2.vi"("error in (no error)"=w2273, "String to write"=w2274, "VISA resource name"=w2276) -> ("error out"=w2272:errorcluster, "VISA resource name out"=w2275:refnum<visa-resource-name>)  [unwired: 7 in]
              }
              frame #7 {
                n1167 = Wait (ms)(milliseconds to wait=w2277) -> ()  [unwired: 1 out]
              }
              frame #8 {
                w2281 = TRUE ("Inject Pump 3")
                n1168 = Tick Count (ms)() -> (millisecond timer value=→"Flush Sample Start Time":u32)
                n1169 = call "Write to pump 2.vi"("error in (no error)"=w2284, "String to write"=w2282, "VISA resource name"=w2285) -> ("error out"=w2283:errorcluster)  [unwired: 7 in, 1 out]
                n1170 = local write "Inject Sample"(w2281) -> ()
                "Flushing Sample" <- w2281
              }
            }
            n1171 = Number To Fractional String(number="Flush \nRate (ul/min)  3") -> (F-format string=w2216:string)  [unwired: 3 in]
            n1172 = String Subset(string=w2216, length (rest)=6 ("length (rest)")) -> (substring=w2215:string)  [unwired: 1 in]
            n1173 = Concatenate Strings("RAT", w2215, "UM") -> (w2230:string)
            n1174 = Divide(x="Flush\nVolume (ul)  3", y=1000.0) -> (x/y=w2221:dbl)
            n1175 = Number To Fractional String(number=w2221) -> (F-format string=w2220:string)  [unwired: 3 in]
            n1176 = Divide(x="Flush\nVolume (ul)  3", y="Flush \nRate (ul/min)  3") -> (x/y=w2211:dbl)
            n1177 = Multiply(x=w2211, y=60.0) -> (x*y=→"Sample flush time (s)":dbl)
            n1178 = String Subset(string=w2220, length (rest)=6 ("length (rest)")) -> (substring=w2219:string)  [unwired: 1 in]
            n1179 = Concatenate Strings("TGT", w2219) -> (w2232:string)
            "error out" <- w2223
          }
          event "Stop": Value Change {
            n1180 = event-data() -> ()  [unwired: 1 in, 5 out]
            n1181 = local read "Stop"() -> (w2286:bool)
          }
          event "Inject Sample": Value Change {
            n1182 = event-data() -> ()  [unwired: 1 in, 5 out]
            n1183 = case shown="True" "Inject Sample" {
              tunnel: w2288 -> [w2290 w2291]
              frame False {
                n1184 = call "Write to pump 2.vi"("String to write"="STP", "VISA resource name"=w2290) -> ()  [unwired: 8 in, 2 out]
              }
              frame True {
                n1185 = local read "Normal \nRate (ul/hr)  3"() -> (w2292:dbl)
                n1186 = Number To Fractional String(number=w2292) -> (F-format string=w2295:string)  [unwired: 3 in]
                n1187 = String Subset(string=w2295, length (rest)=6 ("length (rest)")) -> (substring=w2293:string)  [unwired: 1 in]
                n1188 = flat-sequence {
                  tunnel: "RUN " -> [w2307]
                  tunnel: [w2309] -> _
                  tunnel: [w2308] -> _
                  tunnel: w2291 -> [w2306]
                  frame #0 {
                    n1189 = call "Write to pump 2.vi"("String to write"=w2307, "VISA resource name"=w2306) -> ("error out"=w2308:errorcluster, "VISA resource name out"=w2309:refnum<visa-resource-name>)  [unwired: 8 in]
                  }
                }
                n1190 = Concatenate Strings("RAT", w2293, "UH" ("string")) -> ()  [unwired: 1 out]
                n1191 = local read "Normal \nVolume (ul) 3"() -> (w2301:dbl)
                n1192 = Divide(x=w2301, y=1000.0) -> (x/y=w2296:dbl)
                n1193 = Number To Fractional String(number=w2296) -> (F-format string=w2299:string)  [unwired: 3 in]
                n1194 = String Subset(string=w2299, length (rest)=6 ("length (rest)")) -> (substring=w2297:string)  [unwired: 1 in]
                n1195 = Concatenate Strings("TGT", w2297) -> ()  [unwired: 1 out]
              }
            }
          }
          event "Normal \nRate (ul/hr)  3": Value Change {
            n1196 = event-data() -> ()  [unwired: 1 in, 5 out]
            n1197 = Number To Fractional String(number="Normal \nRate (ul/hr)  3") -> (F-format string=w2313:string)  [unwired: 3 in]
            n1198 = String Subset(string=w2313, length (rest)=6 ("length (rest)")) -> (substring=w2311:string)  [unwired: 1 in]
            n1199 = Concatenate Strings("RAT", w2311, "UH") -> (w2314:string)
            n1200 = call "Write to pump 2.vi"("String to write"=w2314, "VISA resource name"=w2315) -> ()  [unwired: 8 in, 2 out]
          }
          event "Clear Volume": Value Change {
            n1201 = event-data() -> ()  [unwired: 1 in, 5 out]
            n1202 = Divide(x="Normal \nVolume (ul) 3", y=1000.0) -> (x/y=w2333:dbl)
            n1203 = Number To Fractional String(number=w2333) -> (F-format string=w2336:string)  [unwired: 3 in]
            n1204 = String Subset(string=w2336, length (rest)=6 ("length (rest)")) -> (substring=w2334:string)  [unwired: 1 in]
            n1205 = flat-sequence {
              tunnel: [w2343] -> w2331
              tunnel: [w2342] -> w2330
              tunnel: w2320 -> [w2341]
              tunnel: w2319 -> [w2340]
              tunnel: [w2345] -> w2328
              tunnel: [w2344] -> w2329
              tunnel: w2325 -> [w2346]
              tunnel: w2331 -> [w2345]
              tunnel: w2330 -> [w2344]
              tunnel: w2329 -> [w2350]
              tunnel: w2328 -> [w2351]
              tunnel: [w2349] -> _
              tunnel: [w2348] -> _
              tunnel: w2318 -> [w2347]
              frame #0 {
                n1206 = call "Write to pump 2.vi"("String to write"=w2340, "VISA resource name"=w2341) -> ("error out"=w2342:errorcluster, "VISA resource name out"=w2343:refnum<visa-resource-name>)  [unwired: 8 in]
              }
              frame #1 {
                n1207 = Wait (ms)(milliseconds to wait=w2346) -> ()  [unwired: 1 out]
              }
              frame #2 {
                n1208 = call "Write to pump 2.vi"("error in (no error)"=w2350, "String to write"=w2347, "VISA resource name"=w2351) -> ("error out"=w2348:errorcluster, "VISA resource name out"=w2349:refnum<visa-resource-name>)  [unwired: 7 in]
              }
            }
            n1209 = local read "Write Wait"() -> (w2325:i32)
            n1210 = Concatenate Strings("TGT", w2334) -> (w2319:string)
            n1211 = local read "Normal \nRate (ul/hr)  3"() -> (w2321:dbl)
            n1212 = local write "Clear Volume"(FALSE ("Clear Volume")) -> ()
            n1213 = Number To Fractional String(number=w2321) -> (F-format string=w2324:string)  [unwired: 3 in]
            n1214 = String Subset(string=w2324, length (rest)=6 ("length (rest)")) -> (substring=w2322:string)  [unwired: 1 in]
            n1215 = Concatenate Strings("RAT", w2322, "UH" ("string")) -> (w2318:string)
          }
        }
        n1216 = node-c288() -> ()  [unwired: 1 in, 1 out]
      }
      n1217 = node-c288(w2205) -> ()  [unwired: 1 out]
    }
  }
  n1218 = node-c288() -> (w84:T12)  [unwired: 4 in]
  n1219 = timed-loop {
    timing: w84 -> [_]
    timing-out: [_] -> w83
    stop <- w2358 stop-if-true
    n1220 = node-c288() -> ()  [unwired: 1 in, 1 out]
    n1221 = event shown="[1] \"Stop\": Value Change" {
      selector: _ -> [_ _]
      dyn-events: _ -> [_ _]
      timeout: _ -> [_ _]
      tunnel: [_ "Stop"] -> w2358
      event Timeout {
        n1222 = event-data() -> ()  [unwired: 1 in, 2 out]
      }
      event "Stop": Value Change {
        n1223 = event-data() -> ()  [unwired: 1 in, 4 out]
      }
    }
    n1224 = node-c288() -> ()  [unwired: 1 in, 1 out]
  }
  n1225 = case shown="True" w73 {
    tunnel: w78 -> [_ w2364]
    tunnel: w77 -> [_ w2363]
    tunnel: w76 -> [_ w2362]
    frame False {
    }
    frame True {
      w2366 = T15 3 items=["no dialog", "OK message", "continue or stop message", "OK message + warnings", "continue/stop + warnings"] ("type of dialog (OK msg:1)")
      w2365 = T15 3 items=["no dialog", "OK message", "continue or stop message", "OK message + warnings", "continue/stop + warnings"] ("type of dialog (OK msg:1)")
      n1226 = call <vilib>:"DAQmx Clear Task.vi"("task in"=w2364, "error in"=w2362) -> ("error out"=w2367:errorcluster)  [unwired: 13 in]
      n1227 = call <vilib>:"DAQmx Clear Task.vi"("task in"=w2363) -> ("error out"=w2368:errorcluster)  [unwired: 14 in]
      n1228 = call <vilib>:"Simple Error Handler.vi"("type of dialog (OK msg:1)"=w2366, "error in (no error)"=w2367) -> ()  [unwired: 3 in, 5 out]
      n1229 = call <vilib>:"Simple Error Handler.vi"("type of dialog (OK msg:1)"=w2365, "error in (no error)"=w2368) -> ()  [unwired: 3 in, 5 out]
    }
  }
  n1230 = case shown="\"Force Feedback\", Default" "?" {
    frame "Force Feedback", Default {
    }
    frame "Raster scan" {
    }
  }
  n1231 = node-c288(w83) -> ()  [unwired: 1 out]
  n1232 = node-c288(w86) -> ()  [unwired: 1 out]
  n1233 = local write "Pause Mouse/Mirror Connection"(FALSE ("Pause Mouse/Mirror Connection")) -> ()
  n1234 = local write "Stop"(FALSE ("Stop all")) -> ()
  "CoordinatesMousePressed" <- T4 {"Horizontal"=0, "Vertical"=0} ("Coords when pressed")
  "Deflection" <- T4 {"Horizontal"=0, "Vertical"=0} ("Coords when pressed")
